vi "myRIO_BRig_RT_v0,82__PortC.vi"() -> ()   [LabVIEW 2014]
uses:
  myRIO_BRig_RT__Case_Exp_stateList.ctl
  myRIO_BRig_RT__Case_NonExp_stateList.ctl
  <vilib>/Platform/TimedLoop/XDataNode/timing_clust.ctl
  <vilib>/Platform/TimedLoop/XDataNode/nitl_modes.ctl
  <vilib>/Platform/TimedLoop/XDataNode/wakeup.ctl
  <vilib>/WebDAVClient/Advanced/SessionHandle.ctl
  <vilib>/myRIO/Common/Instrument Driver Framework/myRIO v1.0/UART/vis/myRIO v1.0 Close UART.vi
  <vilib>/FPGAPlugInAG/myRIO-1900/niLvFpga_Open_myRIO-1900.vi
  <vilib>/rvi/interface/common/dynamic/niFpgaDynamicAddResources.vi
  <vilib>/Utility/error.llb/Error Cluster From Error Code.vi
  <vilib>/rvi/errors/niLvFpgaAdjustHostInterfaceError.vi
  <vilib>/FPGAPlugInAG/Dynamic/niLvFpga_Close_Dynamic.vi
  <vilib>/myRIO/Common/Instrument Driver Framework/Utilities/vis/FPGA Ref Manager.vi
  <vilib>/myRIO/Common/Instrument Driver Framework/myRIO v1.0/myRIO v1.0 Reset FPGA.vi
  <vilib>/myRIO/Common/Instrument Driver Framework/myRIO v1.0/IRQ/vis/myRIO v1.0 IRQ Info FGV.vi
  <vilib>/myRIO/Common/Instrument Driver Framework/myRIO v1.0/IRQ/vis/myRIO v1.0 Timer IRQ Info FGV.vi
  <vilib>/myRIO/Common/Instrument Driver Framework/myRIO v1.0/IRQ/vis/myRIO v1.0 ISR Agent.vi
  <vilib>/rvi/interface/nirviOpenFPGA/nirviOpenFPGA.xnode
  myRIO_BRig_FPGA_v3,71__PortC__build.lvbitx
  myRIO_BRig_FPGA_v3,71__PortC.vi
  <vilib>/rvi/interface/nirviReadWriteControl/nirviReadWriteControl.xnode
  <vilib>/Platform/TimedLoop/XDataNode/XDataNode.xnode
  <vilib>/rvi/interface/nirviCloseFPGA/nirviCloseFPGA.xnode
  <vilib>/Platform/TimedLoop/XDataNode/XDNodeRunTimeDep.lvlib
  <vilib>/rvi/interface/Simulation/niFpgaSimulationCallBeginRW.vi
  <vilib>/myRIO/Instrument Drivers/Utilities/Utilities.lvlib
  <vilib>/WebDAVClient/NI_WebDAV.lvlib
  NiFpgaLv.dll
panel:
  in  "MTrig_CueLed":bool
  out "Threshold":bool
  out "tLoop":dbl
  in  "Tcycle_Cue_LED_max":u16=1000 caption="Max" min=5 max=5000 step=5
  in  "Tcycle_Cue_LED_min":u16=1000 caption="Min" min=5 max=5000 step=5
  in  "Tcycle_CuePenalty_LED":u16=1000 caption="Penalty" min=1 max=10000 step=1
  out "power_l2":dbl
  in  "MTrig_Laser_Switch":bool
  in  "Cue1Param_AudioLed_Count_NS":u16
  in  "Cue1Param_AudioLed_Count_Switch":u16
  in  "Cue1Param_AudioLed_Probability_NS":u16
  in  "Cue1Param_CueType_NS":u16(slide) max=2 step=1 scale=0.0..2.0
  in  "Cue1Param_AudioLed_Probability_Switch":u16
  in  "Cue1Param_CueType_Switch":u16(slide) max=2 step=1 scale=0.0..2.0
  in  "CueLed_Freq":dbl=10.0
  in  "CueLed_Tpeak":dbl=2.0
  in  "Laser_power_step_l2":dbl
  in  "Laser_power_max_l2":dbl
  in  "Laser_power_min_l2":dbl
  in  "Laser_Tshutter_l2":dbl=2.0
  in  "Laser_Freq_l2":dbl=10.0
  in  "Laser_Tpeak_l2":dbl=2.0
  in  "Laser_duration_l2":u16
  in  "LC_Sel_Count_NS_l2":u16
  in  "LC_Sel_Count_Switch_l2":u16
  in  "LC_Sel_Probability_NS_l2":u16
  in  "LC_Sel_Block_NS_l2":u16(slide) max=2 step=1 scale=0.0..2.0
  in  "LC_Sel_OnOff_NS_l2":bool
  in  "LC_Sel_Probability_Switch_l2":u16
  in  "LC_Sel_Block_Switch_l2":u16(slide) max=2 step=1 scale=0.0..2.0
  in  "LC_Sel_OnOff_Switch_l2":bool
  in  "LC_Sel_Tdelay_NS_l2":u16
  in  "LC_Sel_Tdelay_Switch_l2":u16
  in  "LC_Cue1_Count_NS_l2":u16
  in  "LC_Cue1_Count_Switch_l2":u16
  in  "LC_Cue1_delayOpt_NS_l2":bool
  in  "LC_ENL1_delayOpt_NS_l2":bool
  in  "LC_ENL1_Count_NS_l2":u16
  in  "LC_ENL1_Count_Switch_l2":u16
  in  "LC_Cue1_delayOpt_Switch_l2":bool
  in  "LC_ENL1_delayOpt_Switch_l2":bool
  in  "LC_Cue1_Probability_NS_l2":u16
  in  "LC_Cue1_Block_NS_l2":u16(slide) max=2 step=1 scale=0.0..2.0
  in  "LC_Cue1_OnOff_NS_l2":bool
  in  "LC_Cue1_Probability_Switch_l2":u16
  in  "LC_Cue1_Block_Switch_l2":u16(slide) max=2 step=1 scale=0.0..2.0
  in  "LC_Cue1_OnOff_Switch_l2":bool
  in  "LC_ENL1_Probability_NS_l2":u16 max=100 step=1
  in  "LC_ENL1_Block_NS_l2":u16(slide) max=2 step=1 scale=0.0..2.0
  in  "LC_ENL1_OnOff_NS_l2":bool
  in  "LC_ENL1_Probability_Switch_l2":u16 max=100 step=1
  in  "LC_ENL1_Block_Switch_l2":u16(slide) max=2 step=1 scale=0.0..2.0
  in  "LC_Cue1_Tdelay_NS_l2":u16
  in  "LC_ENL1_Tdelay_NS_l2":u16
  in  "LC_Cue1_Tdelay_Switch_l2":u16
  in  "LC_ENL1_Tdelay_Switch_l2":u16
  in  "LC_ENL1_OnOff_Switch_l2":bool
  in  "LC_Wrong_Probability_l2":u16
  in  "LC_Wrong_Trial_l2":u16(slide) max=2 step=1 scale=0.0..2.0
  in  "LC_Wrong_Block_l2":u16(slide) max=2 step=1 scale=0.0..2.0
  in  "LC_Wrong_OnOff_l2":bool
  in  "LC_Reward_Probability_l2":u16
  in  "LC_Reward_Trial_l2":u16(slide) max=2 step=1 scale=0.0..2.0
  in  "LC_Reward_Block_l2":u16(slide) max=2 step=1 scale=0.0..2.0
  in  "LC_Reward_OnOff_l2":bool
  in  "LC_Wrong_Tdelay_l2":u16
  in  "LC_Reward_Tdelay_l2":u16
  in  "LC_Sel_Count_NS_l1":u16
  in  "LC_Sel_Count_Switch_l1":u16
  in  "LC_Sel_Probability_NS_l1":u16
  in  "LC_Sel_Block_NS_l1":u16(slide) max=2 step=1 scale=0.0..2.0
  in  "LC_Sel_OnOff_NS_l1":bool
  in  "LC_Sel_Probability_Switch_l1":u16
  in  "LC_Sel_Block_Switch_l1":u16(slide) max=2 step=1 scale=0.0..2.0
  in  "LC_Sel_OnOff_Switch_l1":bool
  in  "LC_Sel_Tdelay_NS_l1":u16
  in  "LC_Sel_Tdelay_Switch_l1":u16
  out "I_connect_TCP":bool
  in  "get_countPerMS":bool
  in  "count_warmup_R_reset":bool
  in  "count_warmup_L_reset":bool
  out "count_warmup_R":u16
  out "count_warmup_L":u16
  out "SolenoidReward":bool
  in  "SolenoidProbability_L":u16=100 caption="Reward Time [ms]" min=1 max=1000 step=1
  in  "SolenoidProbability_R":u16=100 caption="Reward Time [ms]" min=1 max=1000 step=1
  out "power_l1":dbl caption="LaserPower"
  in  "Laser_power_step_l1":dbl
  in  "Laser_power_max_l1":dbl
  in  "Recording":bool
  in  "Laser_power_min_l1":dbl
  in  "FPGA_count2ms":dbl=159.0
  in  "Laser_Tshutter_l1":dbl=2.0
  in  "Laser_Freq_l1":dbl=10.0
  in  "Laser_Tpeak_l1":dbl=2.0
  in  "Laser_duration_l1":u16
  out "error out":errorcluster
  in  "LC_Cue1_Count_NS_l1":u16
  in  "LC_Cue1_Count_Switch_l1":u16
  in  "LC_Cue1_delayOpt_NS_l1":bool
  in  "LC_ENL1_delayOpt_NS_l1":bool
  in  "LC_ENL1_Count_NS_l1":u16
  in  "LC_ENL1_Count_Switch_l1":u16
  in  "LC_Cue1_delayOpt_Switch_l1":bool
  in  "LC_ENL1_delayOpt_Switch_l1":bool
  in  "Tcycle_Cue_Audio_max":u16=1000 caption="Max" min=5 max=5000 step=5
  in  "Tcycle_Cue_Audio_min":u16=1000 caption="Min" min=5 max=5000 step=5
  in  "SendData":bool
  out "cSpout":enum16{"Left", "Right"}(ring) caption="Left or Right Spout"
  out "A4":u32 caption="LickCounter_Right"
  out "A2":u32 caption="LickCounter_Left"
  in  "LR_wrong_Event":bool
  out "SelectWrong":bool
  out "SelectReward":bool
  in  "Left(F)_or_Right(T)":bool
  in  "ignoreWrong":bool
  in  "SelectionState":bool
  in  "LR_wrong_Laser":bool
  in  "LR_reward_Laser":bool
  in  "LR_reward_Event":bool
  out "nRewards_Right":u16 caption="# Rewards Total (Right)"
  out "nRewards_Left":u16 caption="# Rewards Total (Left)"
  out "nRewards_cur":u16 caption="# Rewards in Current Block"
  out "TpB_target":u16 caption="Target Trials Per Block"
  out "cState_NonExp":T1 caption="WarmUp State"
  out "iBlock":u16 caption="Current Block"
  out "cState":T2 caption="Experimental State"
  out "iTrial":u16 caption="Current Trial"
  in  "warmupType":u8(slide) max=2 step=1 scale=0.0..2.0
  in  "TestConnection":bool
  in  "warmup":bool caption="WarmUp"
  in  "Data Set Prefix":string="Exp1_TM2"
  out "Connected To Host?":bool
  in  "Host Password":string="sabalab"
  in  "Host UserName":string="Test2"
  in  "sp_RightSpout":u16(slide)=2 max=2 step=1 scale=0.0..2.0
  in  "sp_LeftSpout":u16(slide)=2 max=2 step=1 scale=0.0..2.0
  in  "BUR_max":u16 caption="Count Reward Structure  (0 = off)"
  in  "LC_Wrong_Probability_l1":u16
  in  "LC_Wrong_Trial_l1":u16(slide) max=2 step=1 scale=0.0..2.0
  in  "LC_Wrong_Block_l1":u16(slide) max=2 step=1 scale=0.0..2.0
  in  "LC_Wrong_OnOff_l1":bool
  in  "LC_Reward_Probability_l1":u16
  in  "LC_Reward_Trial_l1":u16(slide) max=2 step=1 scale=0.0..2.0
  in  "LC_Reward_Block_l1":u16(slide) max=2 step=1 scale=0.0..2.0
  in  "LC_Reward_OnOff_l1":bool
  in  "LC_Cue1_Probability_NS_l1":u16
  in  "LC_Cue1_Block_NS_l1":u16(slide) max=2 step=1 scale=0.0..2.0
  in  "LC_Cue1_OnOff_NS_l1":bool
  in  "LC_Cue1_Probability_Switch_l1":u16
  in  "LC_Cue1_Block_Switch_l1":u16(slide) max=2 step=1 scale=0.0..2.0
  in  "LC_Cue1_OnOff_Switch_l1":bool
  in  "LC_ENL1_Probability_NS_l1":u16 max=100 step=1
  in  "LC_ENL1_Block_NS_l1":u16(slide) max=2 step=1 scale=0.0..2.0
  in  "LC_ENL1_OnOff_NS_l1":bool
  in  "LC_ENL1_Probability_Switch_l1":u16 max=100 step=1
  in  "LC_ENL1_Block_Switch_l1":u16(slide) max=2 step=1 scale=0.0..2.0
  in  "Tcycle_Timeout":u16=1000 caption="Timeout Time [ms]" min=10 max=10000 step=1
  in  "Tcycle_Wrong":u16=1000 caption="Wrong Time [ms]" min=10 max=10000 step=1
  in  "Tcycle_Selection":u16=1000 caption="Answer Time [ms]" min=1 max=10000 step=1
  in  "Tcycle_RewardPost":u16=1000 caption="Consumption Time [ms]" min=250 max=10000 step=250
  in  "Tcycle_Reward_L":u16=500 caption="Reward Time [ms]" min=1 max=1000 step=1
  in  "Tcycle_Reward_R":u16=500 caption="Reward Time [ms]" min=1 max=1000 step=1
  in  "TpB_Max_R":u16=4 caption="Max TrialsPerBlock" min=1 max=12 step=1
  in  "TpB_Min_R":u16=4 caption="Min TrialsPerBlock" min=1 max=12 step=1
  in  "TpB_Max_L":u16=4 caption="Max TrialsPerBlock" min=1 max=12 step=1
  in  "TpB_Min_L":u16=4 caption="Min TrialsPerBlock" min=1 max=12 step=1
  in  "BUR_min":u16 caption="Count Reward Structure\n(0 = off)"
  in  "TrialUntilReward":bool caption="Ignore Wrong Selection"
  in  "CueCycles":u16=1 caption="Cue Structure" min=1 max=1 step=1
  in  "MTrig_Laser_Tcycle":u16=10 caption="Time [ms]"
  in  "MTrig_Laser_trig":bool
  in  "MTrig_Audio_trig__R":bool caption="Trigger Audio"
  in  "MTrig_Audio_trig__L":bool caption="Trigger Audio"
  in  "RewCalib_Trig_R":bool caption="Calibrate_R"
  in  "RewCalib_Trig_L":bool caption="Calibrate_L"
  in  "MTrig_Solenoid_Tcycle__R":u16=300 caption="Time [ms]"
  in  "MTrig_Solenoid_Tcycle__L":u16=300 caption="Time [ms]"
  in  "MTrig_Solenoid_trig__R":bool caption="Solenoid"
  in  "MTrig_Solenoid_trig__L":bool caption="Solenoid"
  in  "STOP_abort":bool caption="Stop LabView\n(Stops myRio and FPGA)"
  in  "STOP_endBlock":bool caption="Stop Experiment\n@ End of Block"
  in  "STOP_endTrial":bool caption="Stop Experiment\n@ End of Trial"
  in  "START":bool caption="Start Experiment"
  in  "Tcycle_CuePenalty_Audio":u16=1000 caption="Penalty" min=1 max=10000 step=1
  in  "Audio_Amp__R":u16=100 caption="Amp"
  in  "Audio_Freq__R":u8=5 caption="Freq [kHz]" max=14 step=1
  in  "Audio_Amp__L":u16=100 caption="Amp"
  in  "Audio_Freq__L":u8=5 caption="Freq [kHz]" max=14 step=1
  in  "LC_Wrong_Tdelay_l1":u16
  in  "LC_Cue1_Tdelay_NS_l1":u16
  in  "LC_ENL1_Tdelay_NS_l1":u16
  in  "LC_Reward_Tdelay_l1":u16
  in  "LC_Cue1_Tdelay_Switch_l1":u16
  in  "LC_ENL1_Tdelay_Switch_l1":u16
  in  "LC_ENL1_OnOff_Switch_l1":bool
  in  "Tcycle_ENLPenalty":u16=100 caption="Penalty" min=10 max=10000 step=10
  in  "Tcycle_ENL_max":u16=1000 caption="Max" min=250 max=10000 step=250
  in  "Tcycle_ENL_min":u16=1000 caption="Min" min=250 max=10000 step=250
  # "Communication (Host PC)"
  # "Recording Rig"
  # "Experimental Run"
  # "Current State"
  # "STOP experiment at"
  # "Global Parameters                                                         Trial Parameters"
  # "Left/Right        Give Reward?        Laser Power [V]"
  # "Laser1      Laser2"
  # "FPGA Count per [ms]"
  # "Experiment Task Structure"
  # "Block                   Trial            Target Trials       # Rewards \n                                                            Per Block             Current"
  # "Min            Max            Penalty"
  # "(1) = Switching\n(2) = Two Choice"
  # "WarmUp State"
  # "Lick Counter"
  # "Enforced\nNonLick"
  # "WarmUp"
  # "Left           Right"
  # "Cue then reward (no lick)\n \nLeft                    Right"
  # "# Rewards Total\n                                                                  Left                    Right"
  # "Cue Audio"
  # "Experimental State"
  # "Cue LED"
  # "Selection\n \n\n \nReward\n    Dispense\n    Time\n \n    Dispense\n    Probability\n \n\n    Consumption\n    Time\n\nWrong Choice\n \n \nTimeout Penalty"
  # "Left                  Right"
  # "Manual Control"
  # "Min"
  # "Max"
  # "Solenoid\n \nLeft              Right"
  # "Speaker\n \nLeft                    Right"
  # "Laser 1  |  Laser 2"
  # "Trial Per Block Structure \n               Left                        Right"
  # "Time\n[ms]"
  # "Time\n[ms]"
  # "Time = Cue Min"
  # "Min"
  # "Cue LED"
  # "Power = Min"
  # "Max"
  # "Cue1 Control\n                                  Cue Type           LED Probability [%]      Count"
  # "Laser1 Control\n                               On/Off      Block        Probability [%]   Delay [ms]                              Count"
  # "Laser2 Control\n                               On/Off      Block        Probability [%]   Delay [ms]                              Count"
  # "Audio or LED"
  # "Cue 1"
  # "Enforced\nNonLick\n      1"
  # "Enforced\nNonLick\n      1"
  # "from end"
  # "from end"
  # "Switch\nTrial"
  # "Switch\nTrial"
  # "Switch\nTrial"
  # "from start"
  # "from start"
  # "from end"
  # "from end"
  # "NonSwitch\nTrials"
  # "NonSwitch\nTrials"
  # "NonSwitch\nTrials"
  # "from start"
  # "from start"
  # "Cue 1"
  # "Cue 1"
  # "from end"
  # "from end"
  # "Switch\nTrial"
  # "Switch\nTrial"
  # "Cue Audio Parameters"
  # "Cue LED Parameters"
  # "from start"
  # "from start"
  # "Left                  Right"
  # "Frequency\n[Hz]"
  # "Frequency\n[kHz]"
  # "from end"
  # "from end"
  # "NonSwitch\nTrials"
  # "NonSwitch\nTrials"
  # "Timing [ms]\n                    Peak Width"
  # "from start"
  # "from start"
  # "Amp\n(0 - 32,000)"
  # "Selection"
  # "Selection"
  # "from start"
  # "from start"
  # "Switch\nTrial"
  # "Switch\nTrial"
  # "Speaker\nPattern\nDuring Cue"
  # "from start"
  # "from start"
  # "NonSwitch\nTrials"
  # "NonSwitch\nTrials"
  # "Laser1 Parameters"
  # "Laser2 Parameters"
  # "Laser1 Response\n                               On/Off      Block       Trial       Probability [%]   Delay [ms]"
  # "Laser2 Response\n                               On/Off      Block       Trial       Probability [%]   Delay [ms]"
  # "Frequency\n[Hz]"
  # "Frequency\n[Hz]"
  # "Timing [ms]\n Duration     Peak Width   Shutter"
  # "Timing [ms]\n Duration     Peak Width   Shutter"
  # "Selection Reward"
  # "Selection Reward"
  # "Laser Power [V]\nMin          Max              Step"
  # "Laser Power [V]\nMin          Max              Step"
  # "Selection Wrong"
  # "Selection Wrong"
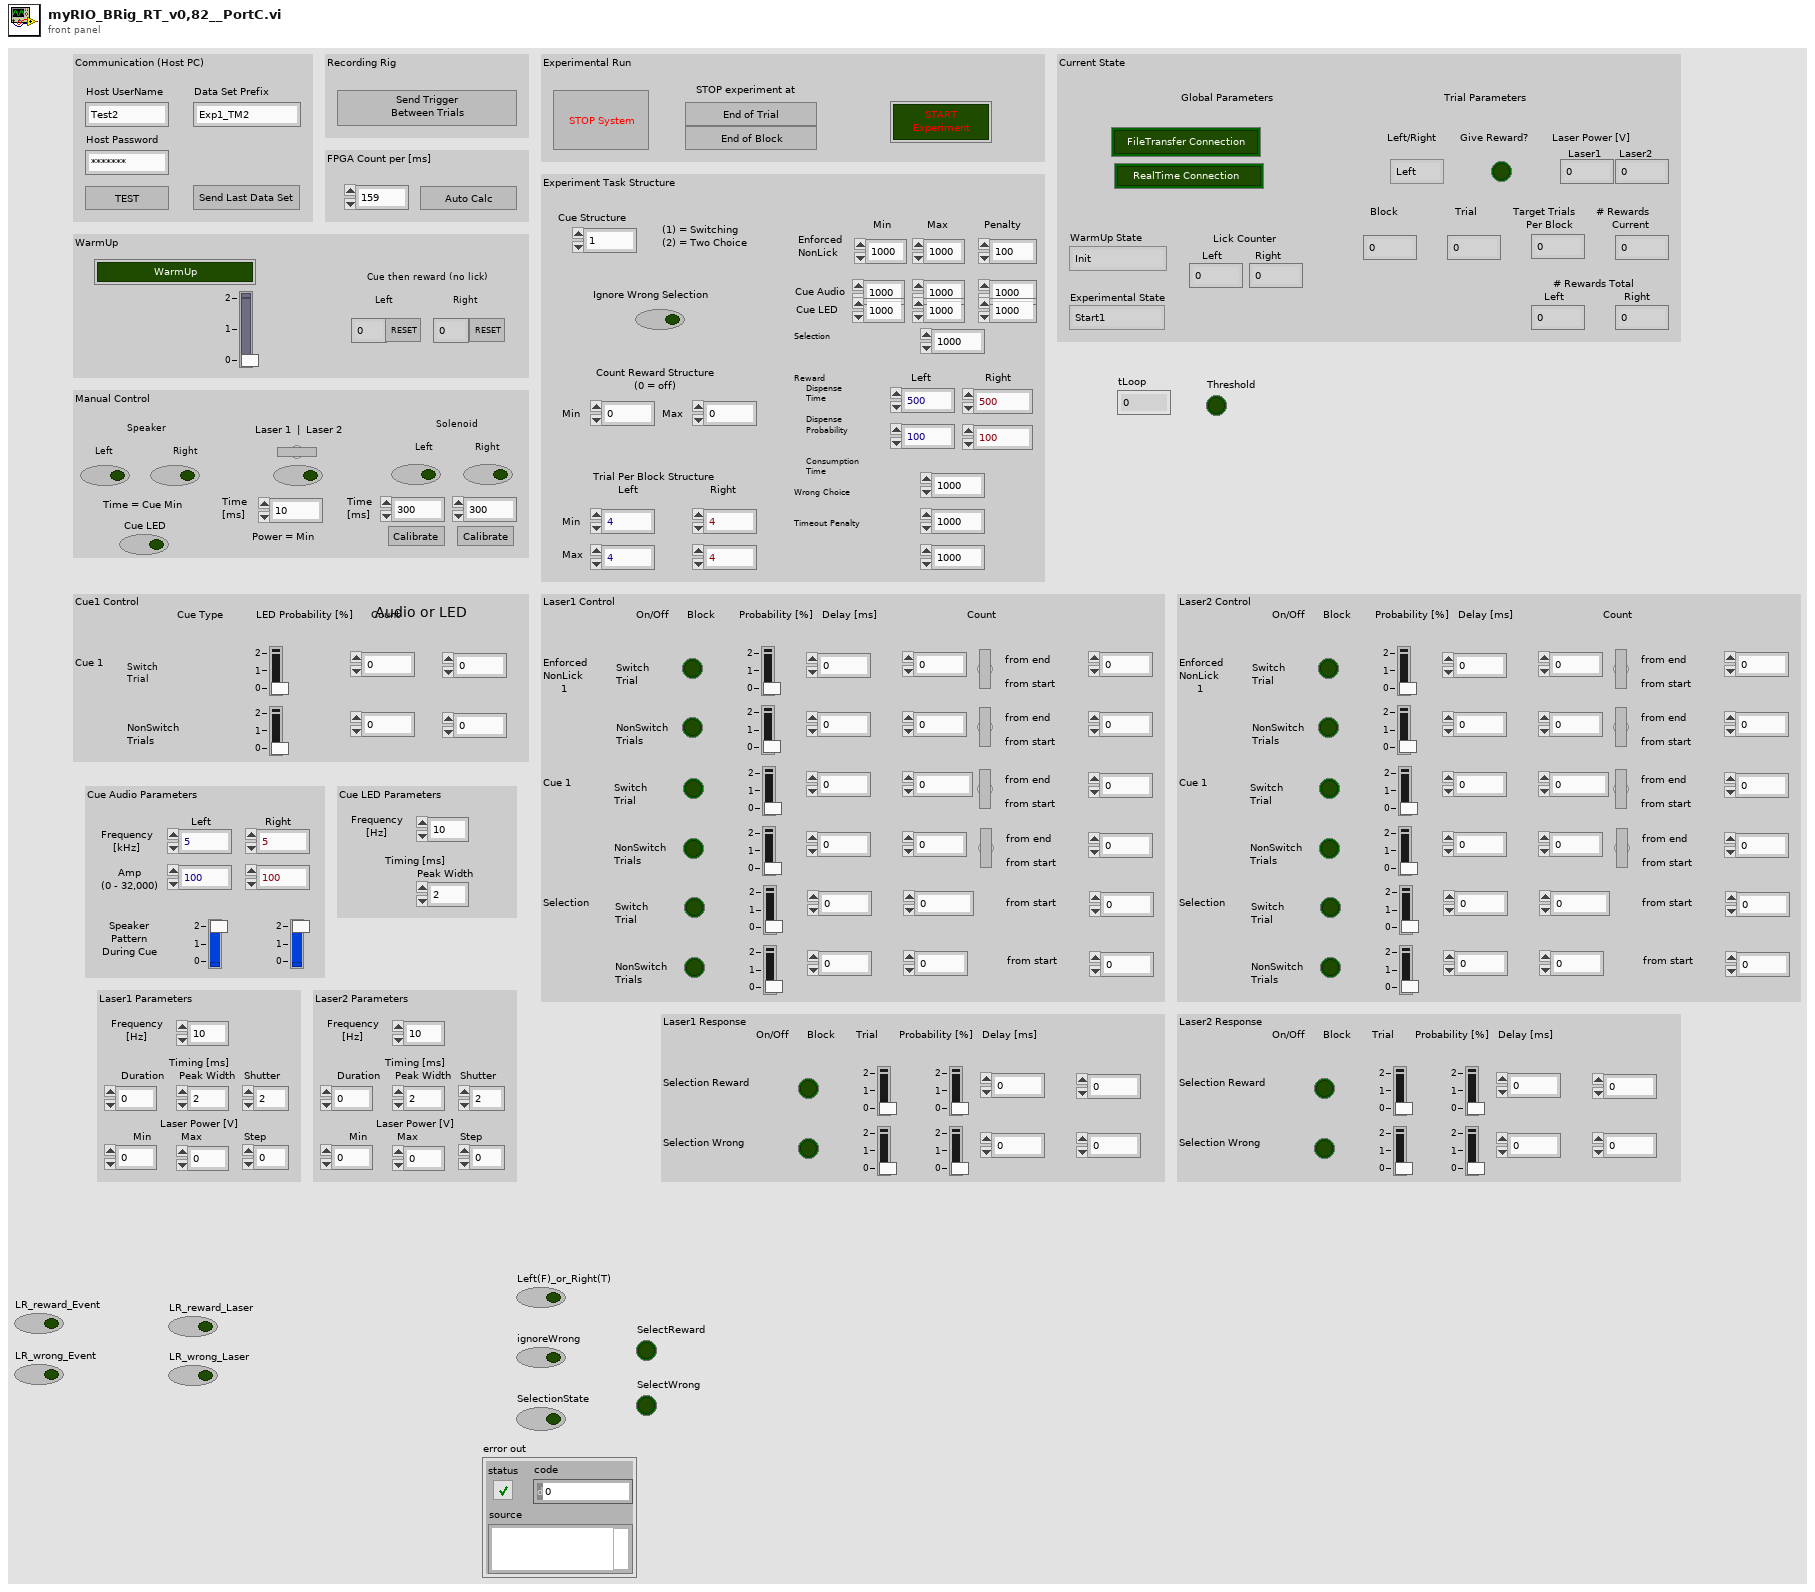
[diagram p1: front panel]
types:
  T1 = typedef "myRIO_BRig_RT__Case_NonExp_stateList.ctl" = enum16{"Init", "UploadSettings_pre", "UploadSettings_Read_dataExp", "UploadSettings_dataExp_1", "UploadSettings_dataExp_2", "UploadSettings_Read_dataLC", "UploadSettings_dataLC_1", "UploadSettings_dataLC_2", "UploadSettings_dataLC_3", "UploadSettings_dataLC_4", "UploadSettings_Read_dataMTrig", "UploadSettings_dataMTrig_1", "UploadSettings_post", "Idle_pre", "IdleEmpty", "IdleEmpty2", "IdleEmpty3", "IdleEmpty4", "Idle", "Idle_2", "Idle_3", "Idle_4", "Idle_5", "Idle_6", "Idle_post", "Cue_pre__pre", "Cue_pre", "Cue", "Cue_LED", "Cue_post", "RewardCalibration_pre", "DispenseWater_pre__pre", "DispenseWater_pre", "DispenseWater", "DispenseWater_post", "TestConnection", "SendData", "Get_FPGA_count_per_ms", "End"}
  T2 = typedef "myRIO_BRig_RT__Case_Exp_stateList.ctl" = enum16{"Start1", "Start2", "Start3", "saveSettings1", "saveSettings2", "saveSettings3", "saveSettings4", "saveSettings_LC_ENL_l1", "saveSettings_LC_ENL_l2", "saveSettings_LC_Cue_l1", "saveSettings_LC_Cue_l2", "saveSettings6_LC_l1_Other", "SaveSettings6_LC_l2_Other", "setSettings_Audio", "setSettings_Laser", "initBlock_pre", "initBlock", "initBlock2", "initBlock_post", "initTrial_pre", "initTrial", "initTrial2", "initTrial3", "initTrial4", "initTrial_LC_ENL1", "initTrial_LC_Cue1", "initTrial_LC_Cue1_2", "initTrial_LC_Sel", "initTrial_post", "ENL1_pre", "ENL1", "ENL1_post", "ENL1Penalty_pre", "ENL1Penalty", "ENL2_pre", "ENL2", "ENL2Penalty_pre", "ENL2Penalty", "Cue1_pre", "Cue1", "Cue1_post", "Cue1Penalty_pre", "Cue1Penalty", "Cue2_pre", "Cue2", "Cue2Penalty_pre", "Cue2Penalty", "Selection_pre", "Selection", "Select_post", "SelectReward_pre", "SelectReward", "SelectRewardPost_pre", "SelectRewardPost", "SelectWrong_pre", "SelectWrong", "SelectWrong_post", "SelectTimeout_pre", "SelectTimeout", "SelectTimeout_post", "endTrial_pre", "endTrial1", "endTrial2", "endTrial3", "endTrial_post", "endBlock_pre", "endBlock", "endBlock_post", "endExp", "commConnect", "commUpload_pre", "commUpload_dataBlock", "commUpload_dataCurrent", "commUpload_dataExp", "commUpload_dataLC", "commUpload_dataTrial", "commUpload_post", "saveData_pre", "saveData_dataBlock", "saveData_dataCurrent", "saveData_dataExp", "saveData_dataLC", "saveData_dataTrial", "saveData_post", "empty_endBlock1", "empty_endBlock2", "empty_endTrial1", "empty_endTrial2", "empty_endTrial3", "empty_endTrial4", "empty_endTrial5", "dummyState", "dummyState_endBlock"}
  T3 = typedef "XDNodeRunTimeDep.lvlib/timing_clust.ctl" = cluster{"Expected End [f-1]":u64, "Actual End [f-1]":u64, "Finished Late? [f-1]":bool, "Expected End [i-1]":u64, "Actual End [i-1]":u64, "Finished Late? [i-1]":bool, "Expected Start [i]":u64, "Actual Start [i]":u64, "Expected Start [f]":u64, "Actual Start [f]":u64, "Source Name":string, "Structure Name":string, "Period":i64, "Deadline":i64, "Offset":i64, "Start":i64, "Priority":i32, "Timeout":i32, "Mode":T4, "Wakeup Reason":T5, "Error":errorcluster, "Source Type":string, "Secondary Source Type":string, "Global End Time":u64, "Global Start Time":u64, "Frame Duration":u64, "Iteration Duration":u64, "Assigned CPU":i32, "I/O Scan Engine Mode":u32}
  T4 = typedef "XDNodeRunTimeDep.lvlib/nitl_modes.ctl" = enum32{"No Change", "Process missed periods, maintain original phase", "Discard missed periods, maintain original phase", "Process missed periods, ignore original phase", "Discard missed periods, ignore original phase"}
  T5 = typedef "XDNodeRunTimeDep.lvlib/wakeup.ctl" = enum32{"Normal", "Aborted", "Asynchronous wakeup", "Timing source error", "Timed loop error", "Timeout"}
  T6 = typedef "NI_WebDAV.lvlib/SessionHandle.ctl" = refnum<k1>
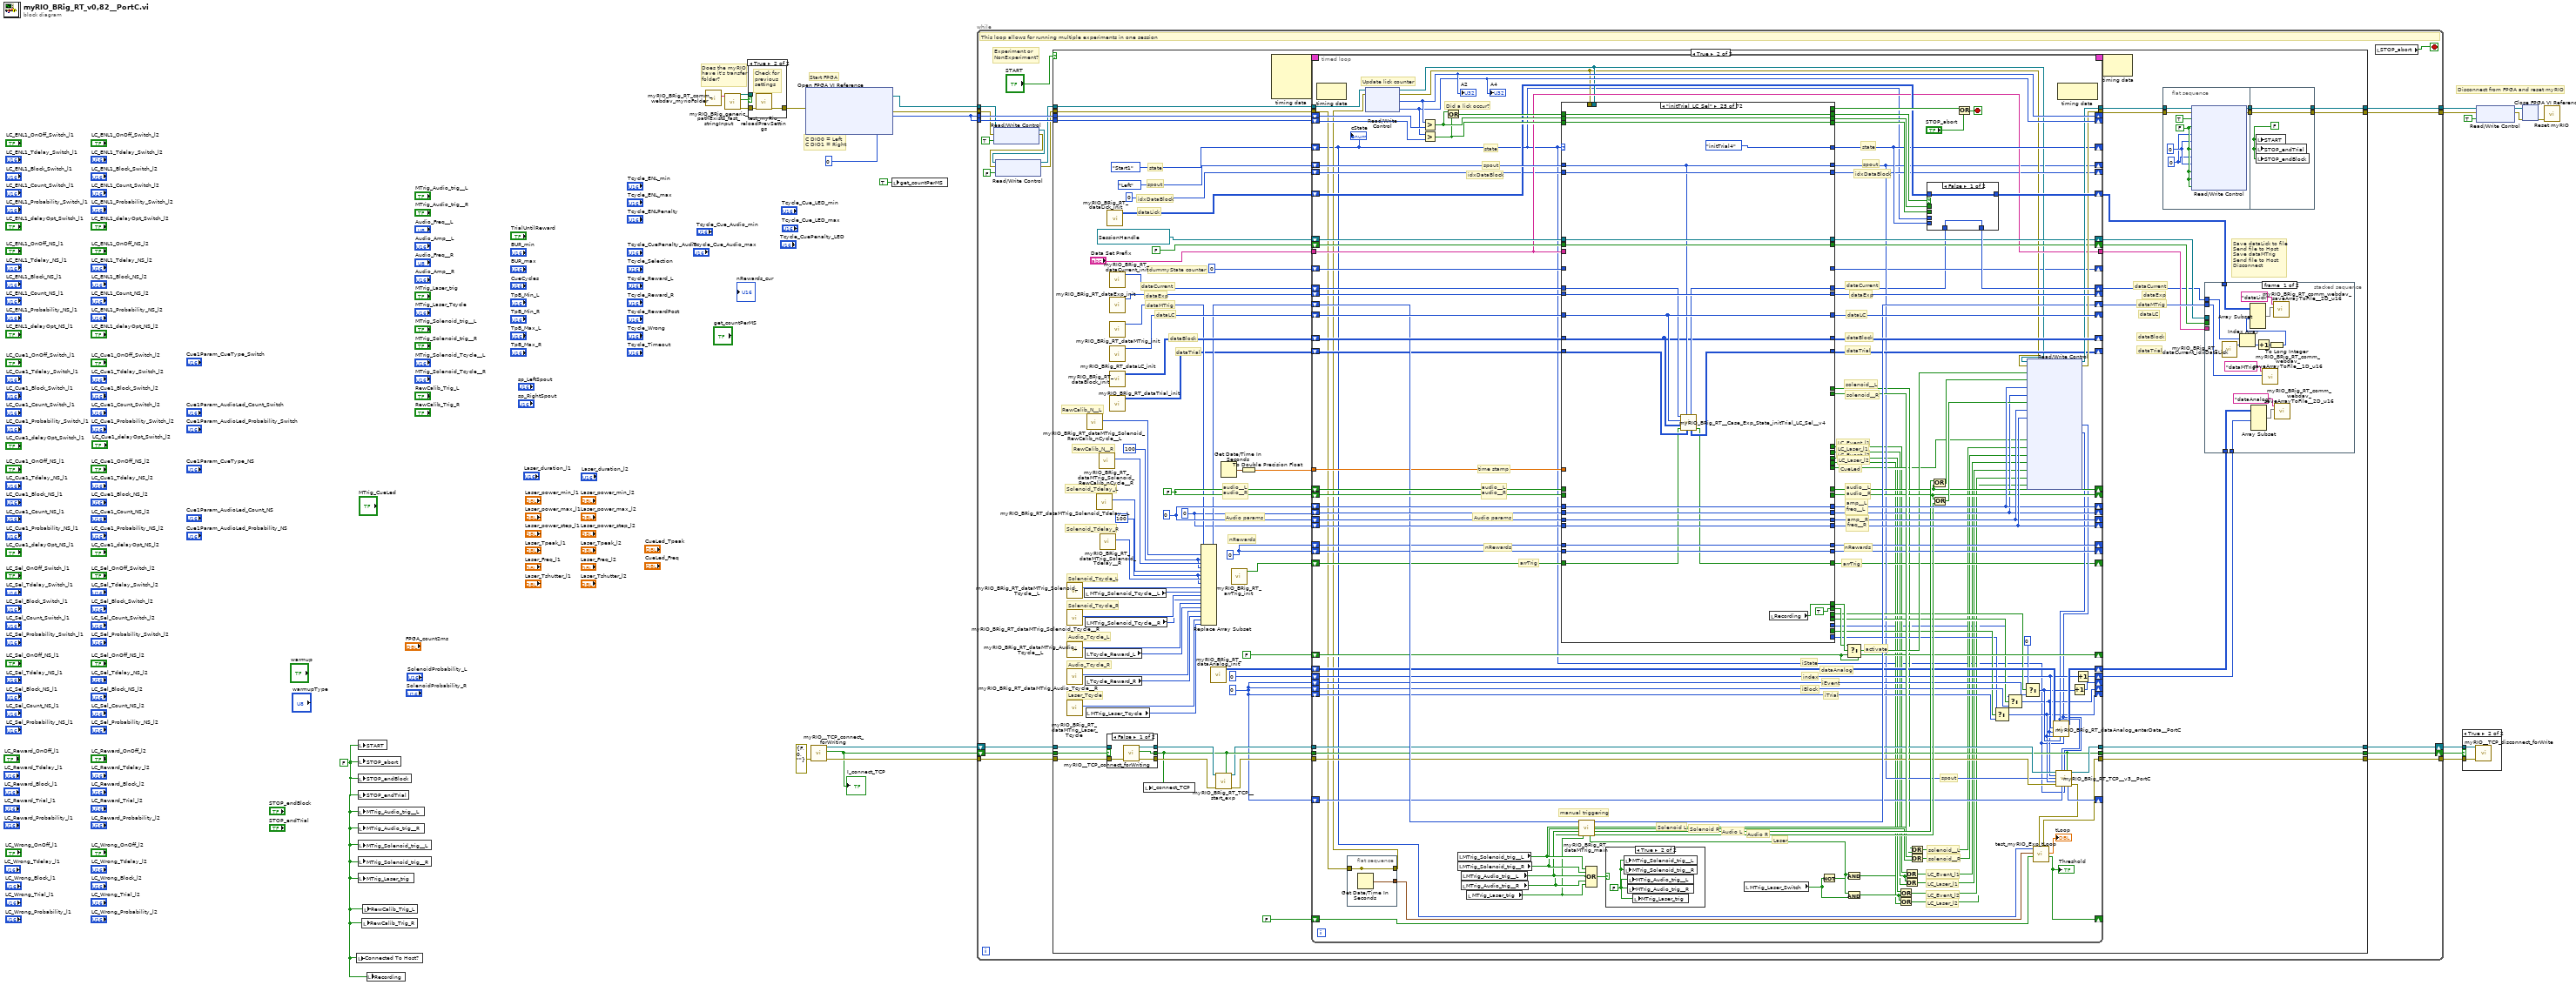
[diagram p0: block diagram]
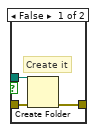
[diagram p3: hidden frame]
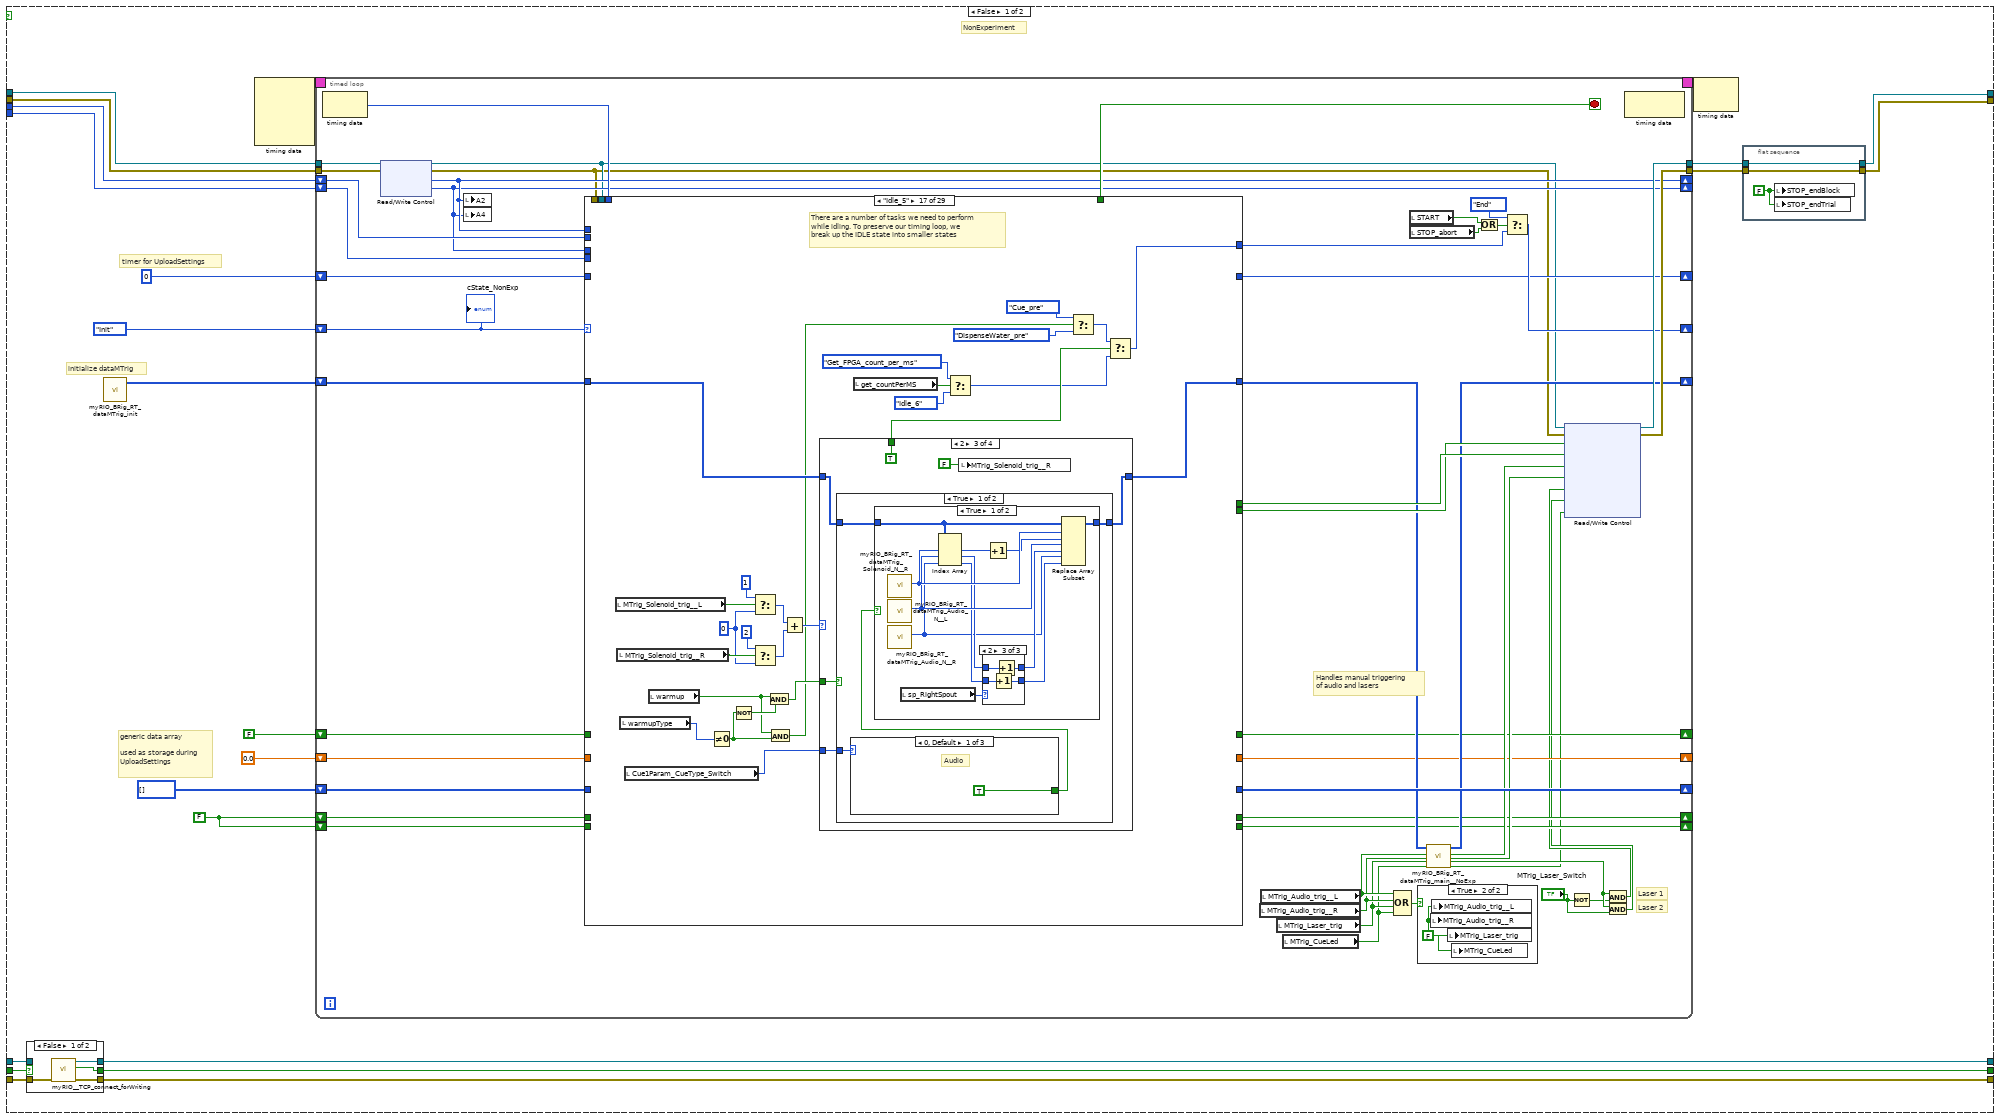
[diagram p4: hidden frame]
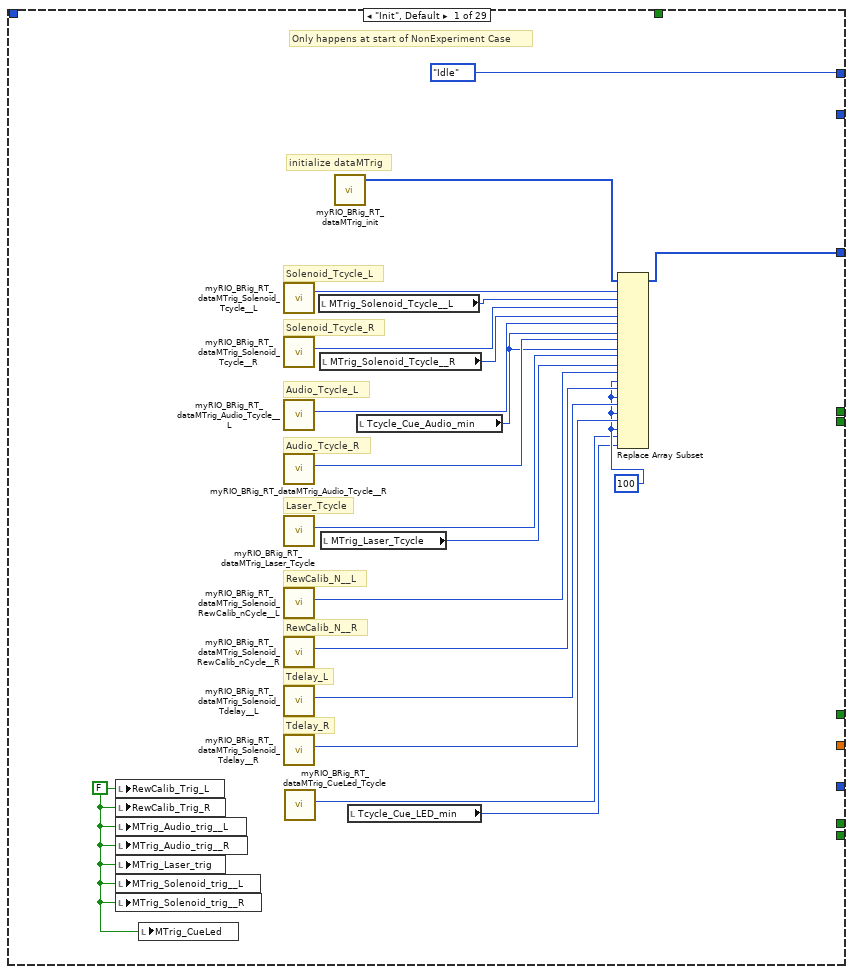
[diagram p7: hidden frame]
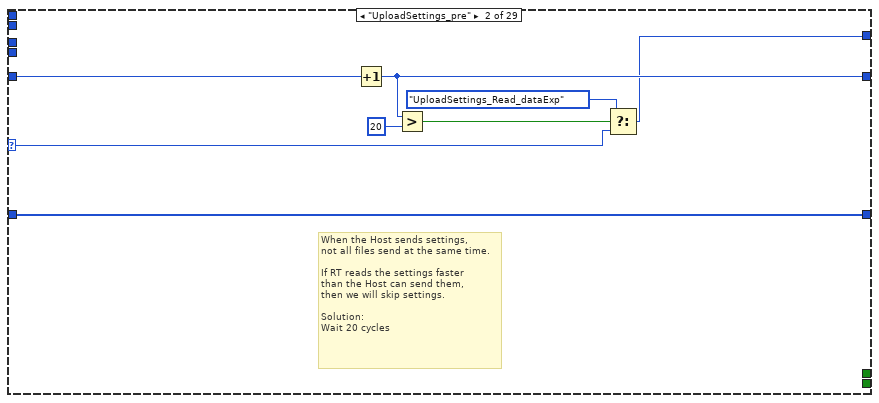
[diagram p8: hidden frame]
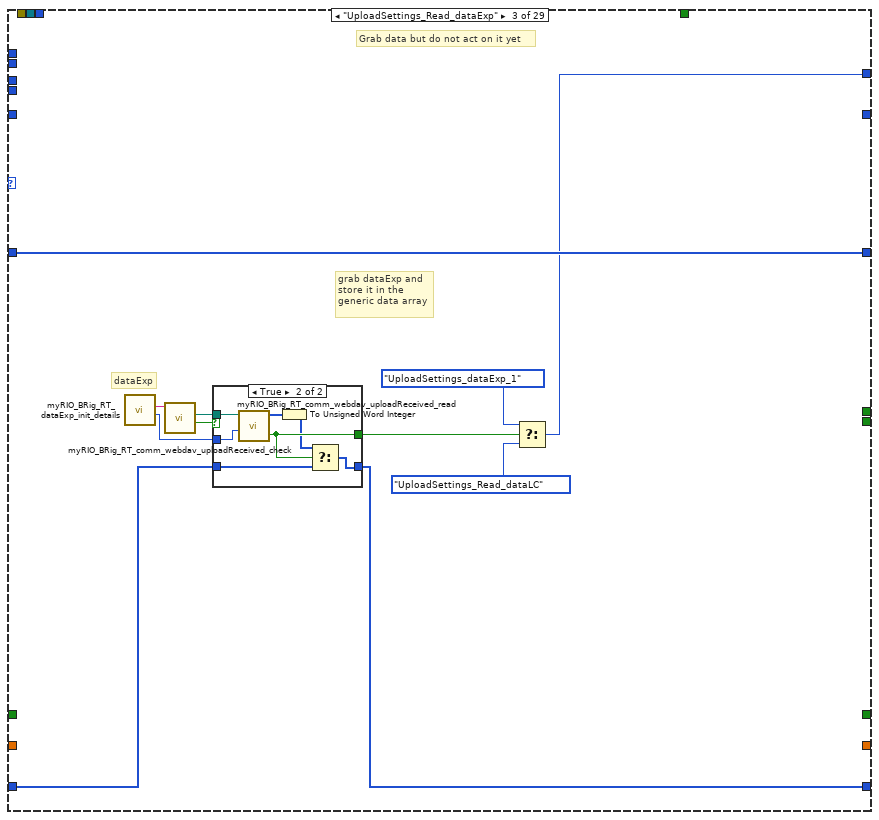
[diagram p9: hidden frame]
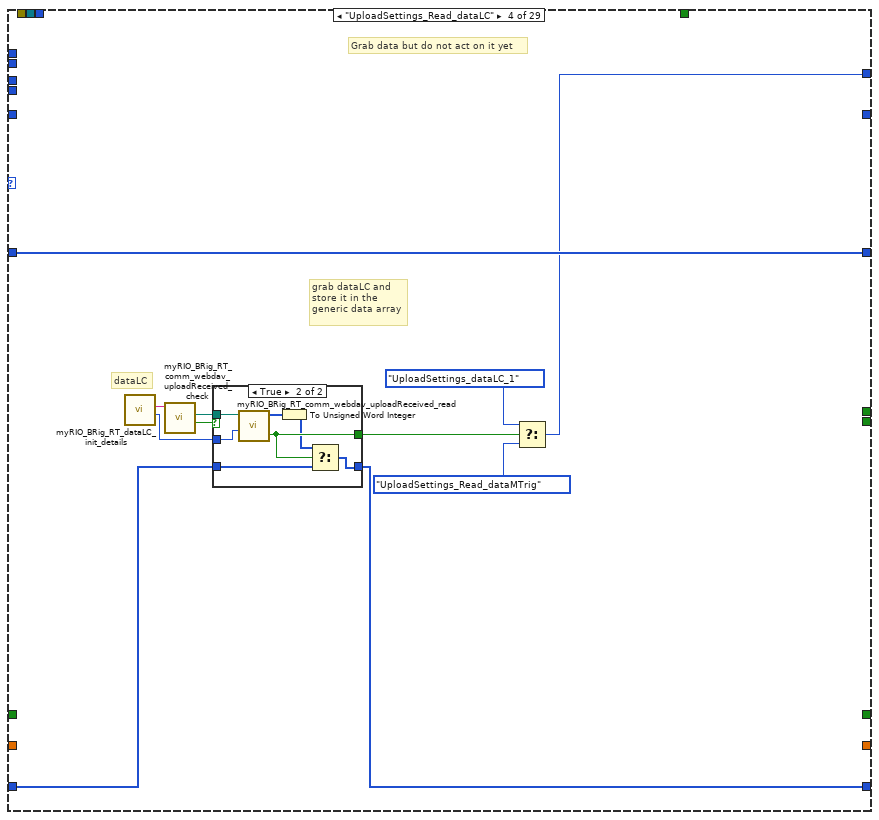
[diagram p11: hidden frame]
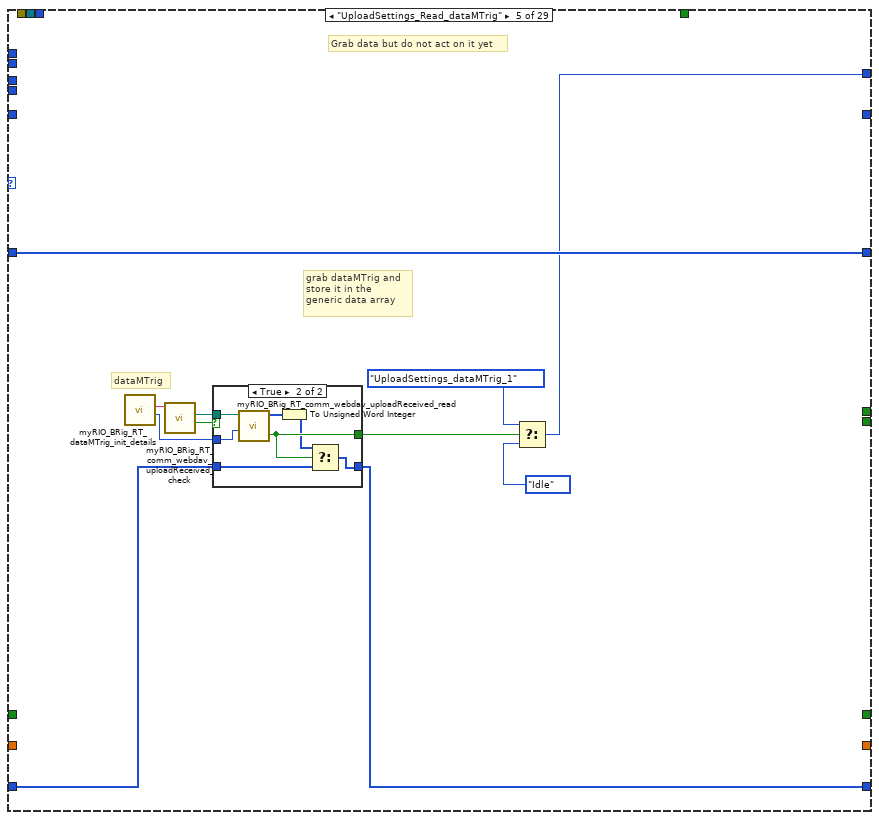
[diagram p13: hidden frame]
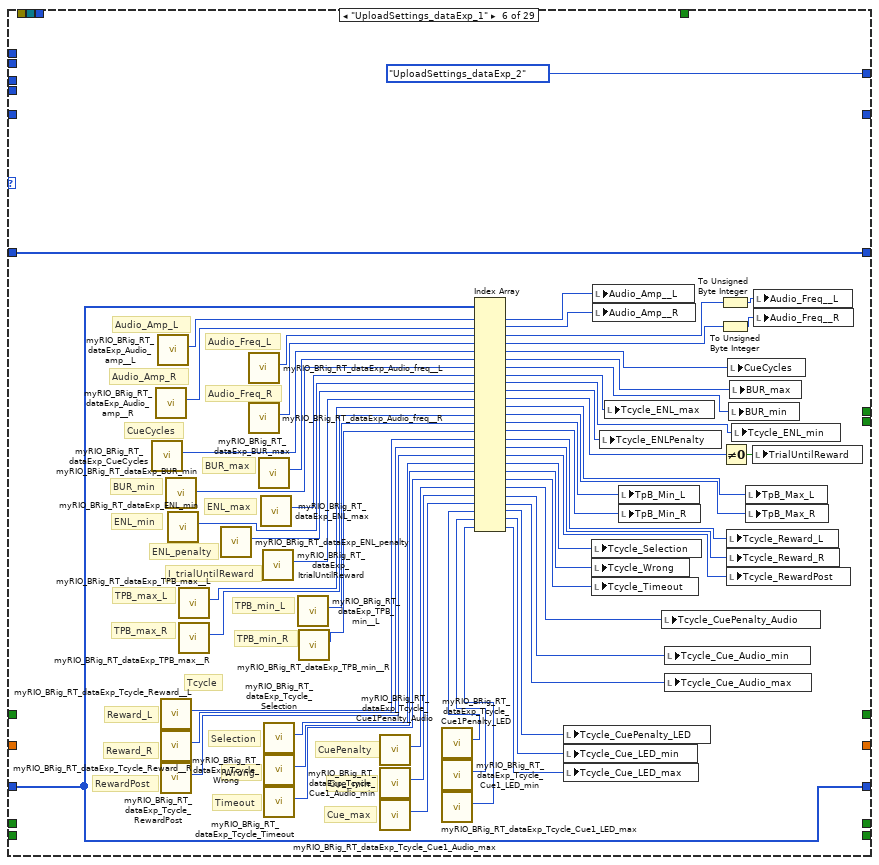
[diagram p15: hidden frame]
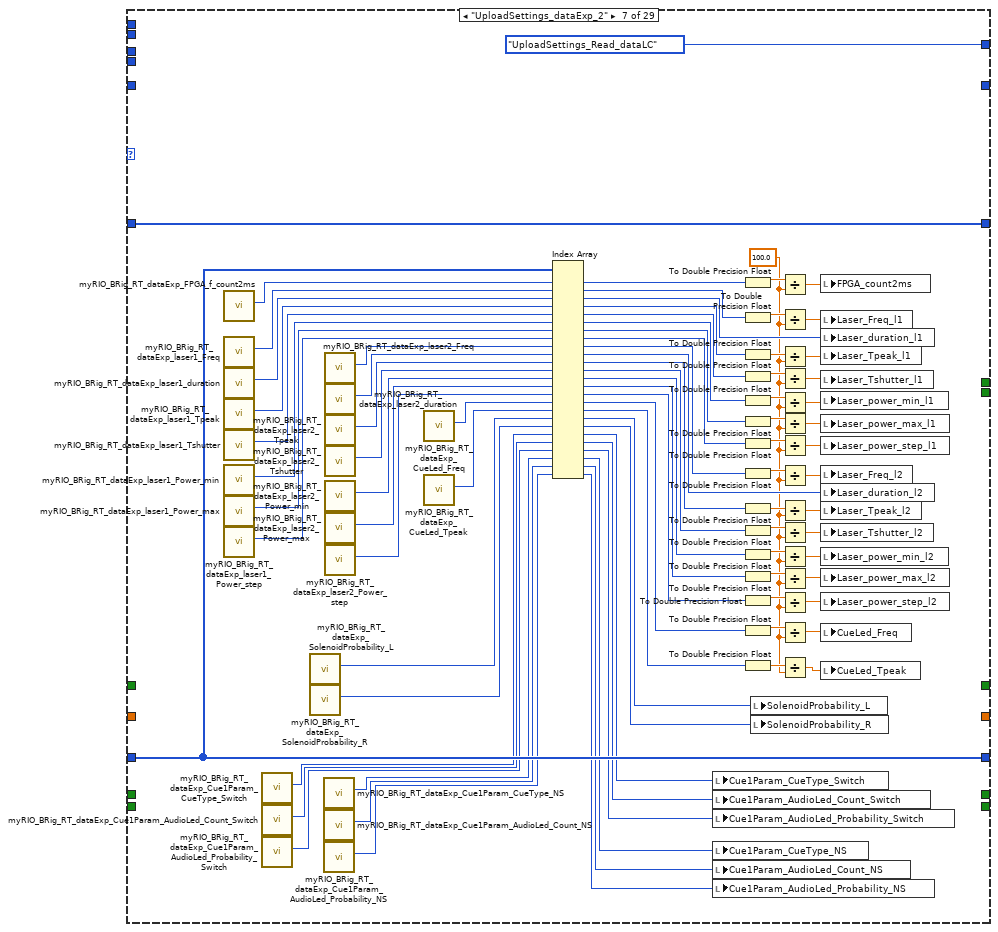
[diagram p16: hidden frame]
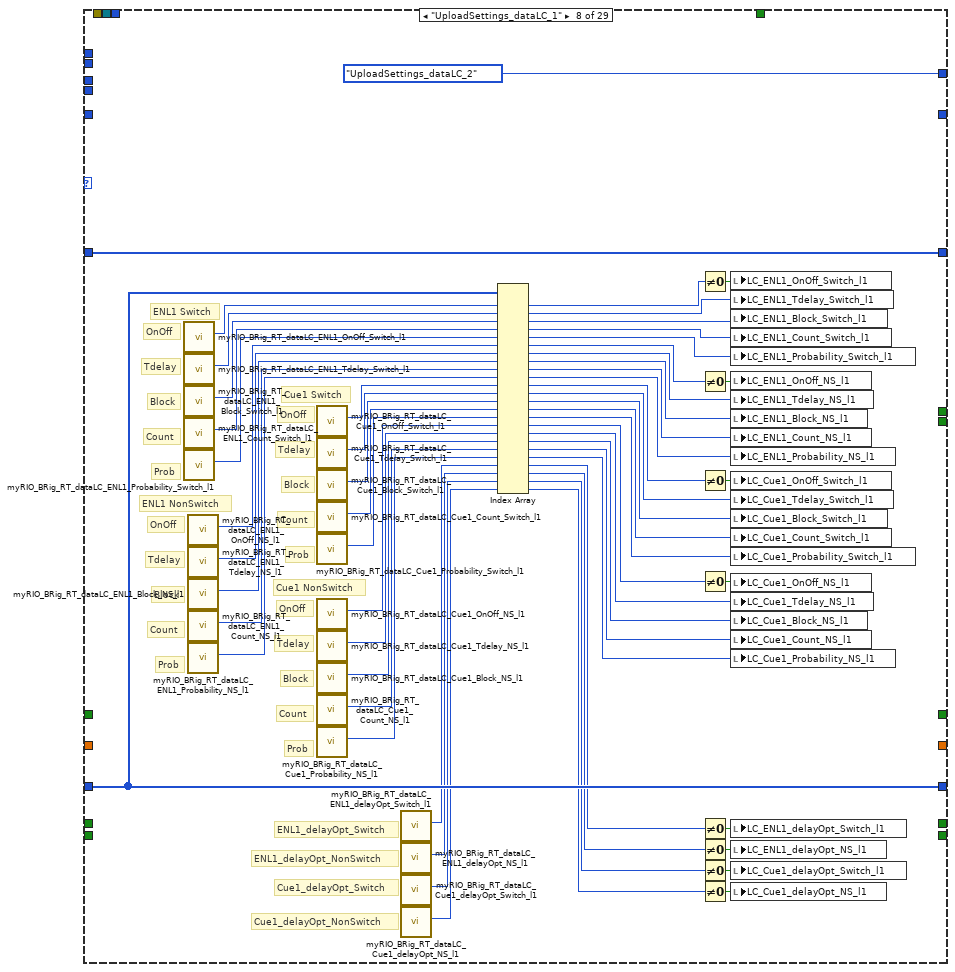
[diagram p17: hidden frame]
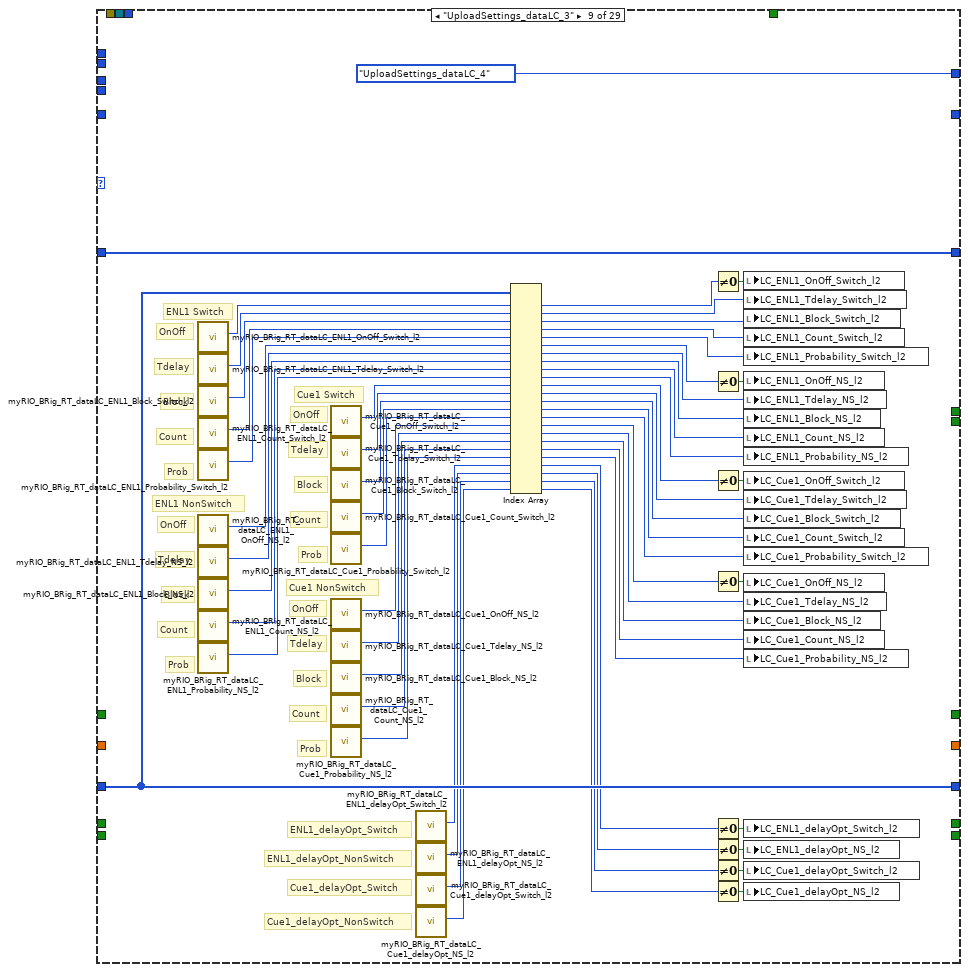
[diagram p18: hidden frame]
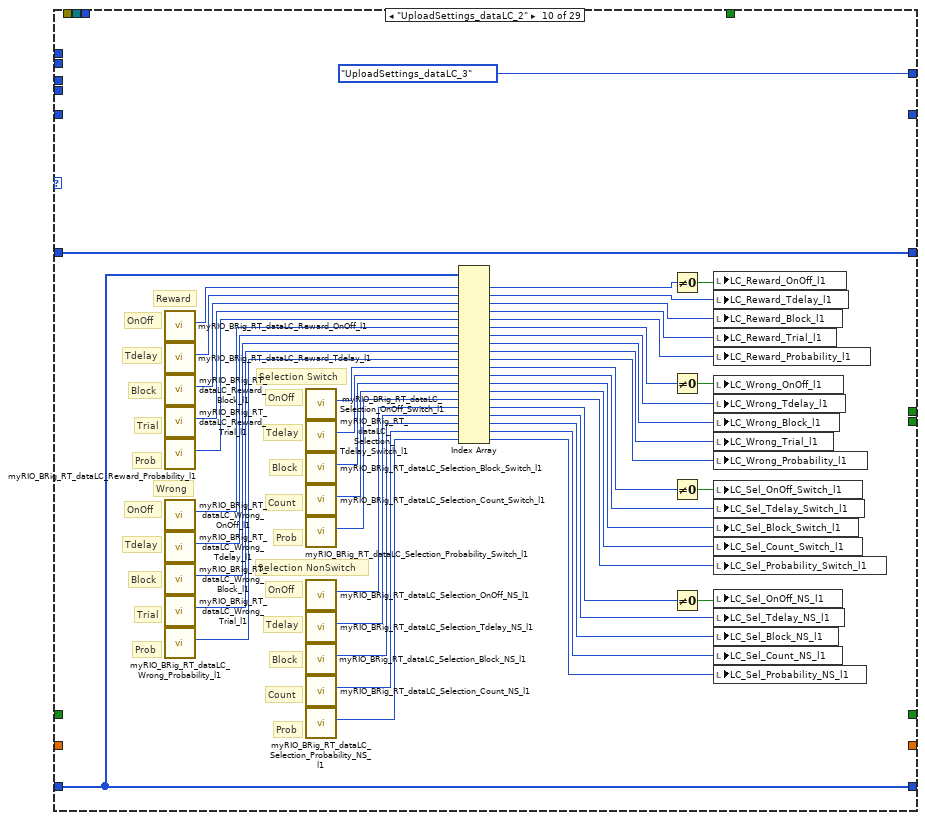
[diagram p19: hidden frame]
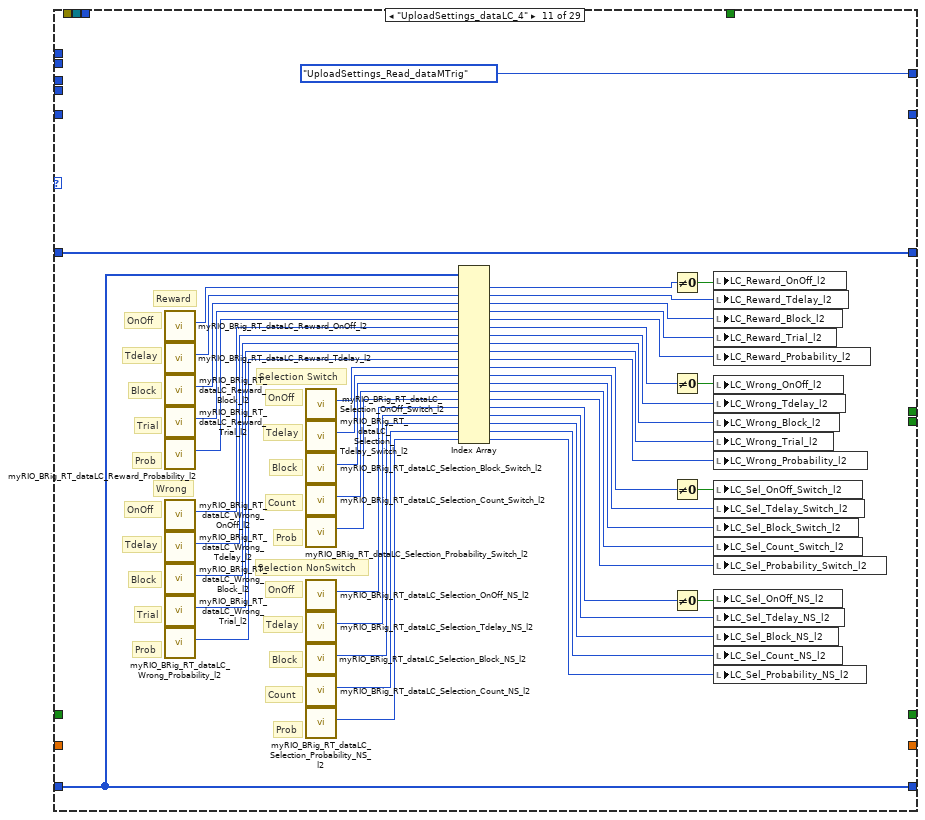
[diagram p20: hidden frame]
diagram:
  w17 = u32 0
  w1 = FALSE
  # "Does the myRIO\nhave it's transfer\nfolder?"
  # "C DIO0 = Left\nC DIO1 = Right"
  # "Start FPGA"
  # "Disconnect from FPGA and reset myRIO"
  n1 = local write "Connected To Host?"(w1) -> ()
  n2 = local write "START"(w1) -> ()
  n3 = local write "STOP_abort"(w1) -> ()
  n4 = local write "STOP_endBlock"(w1) -> ()
  n5 = local write "STOP_endTrial"(w1) -> ()
  n6 = local write "MTrig_Audio_trig__L"(w1) -> ()
  n7 = local write "MTrig_Audio_trig__R"(w1) -> ()
  n8 = local write "MTrig_Solenoid_trig__L"(w1) -> ()
  n9 = local write "MTrig_Solenoid_trig__R"(w1) -> ()
  n10 = local write "MTrig_Laser_trig"(w1) -> ()
  n11 = local write "RewCalib_Trig_R"(w1) -> ()
  n12 = local write "RewCalib_Trig_L"(w1) -> ()
  n13 = local write "Recording"(w1) -> ()
  n14 = call "myRIO_BRig_RT_comm_webdav_myrioFolder.vi"() -> ("output_myrioFolder"=w14:string)  [unwired: 11 in]
  n15 = call "myRIO_BRig_generic_pathExists_fast_stringInput.vi"("input_filePath"=w14) -> ("output_error"=w13:errorcluster, "output_Iexist"=w12:bool, "output_filePath"=w11:path)  [unwired: 8 in]
  n16 = case shown="True" w12 {
    tunnel: w11 -> [w26 _]
    tunnel: w13 -> [w25 w28]
    tunnel: [w24 w27] -> w9
    frame False {
      # "Create it"
      n17 = Create Folder(path (use dialog)=w26, error in=w25) -> (error out=w24:errorcluster)  [unwired: 1 in, 2 out]
    }
    frame True {
      # "Check for\nprevious\nsettings"
      n18 = call "test_myRio_reloadPrevSettings.vi"("input_error"=w28) -> ("output_error"=w27:errorcluster)  [unwired: 10 in]
    }
  }
  n19 = xnode "Open FPGA VI Reference"("error in"=w9) -> ("FPGA VI Reference Out"=w19:refnum<k20>, "error out"=w18:errorcluster)  [unwired: 1 in]
  n20 = call "myRIO__TCP_connect_forWriting.vi"("input_error"=errorcluster {"status"=FALSE, "code"=0, "source"=""}) -> ("output_error"=w7:errorcluster, "output_connected"=w6:bool, "output_hTCP"=w10:refnum<k5>)  [unwired: 8 in]
  "I_connect_TCP" <- w6
  n21 = local write "get_countPerMS"(TRUE ("get_countPerMS")) -> ()
  n22 = while {
    tunnel: w19 -> [w38]
    tunnel: w18 -> [w43]
    tunnel: w17 -> [w46]
    tunnel: w17 -> [w45]
    tunnel: [w36] -> w16
    tunnel: [w35] -> w15
    shift-right: [w32] -> w5
    shift-left: w6 -> [w33]
    tunnel: w7 -> [w31]
    shift-right: [w30] -> w4
    shift-left: w10 -> [w34]
    tunnel: [w29] -> w3
    stop <- w44 stop-if-true
    # "Experiment or\nNonExperiment?"
    # "This loop allows for running multiple experiments in one session"
    n23 = xnode "Read/Write Control"("FPGA VI Reference In"=w38, "error in"=w43, "Counts_Reset"=TRUE) -> ("FPGA VI Reference Out"=w40:refnum<k20>, "error out"=w41:errorcluster)
    n24 = xnode "Read/Write Control"("FPGA VI Reference In"=w40, "error in"=w41, "Counts_Reset"=FALSE) -> ("FPGA VI Reference Out"=w37:refnum<k20>, "error out"=w39:errorcluster)
    n25 = case shown="True" "START" {
      tunnel: w46 -> [w67 w1517]
      tunnel: w45 -> [w66 w1516]
      tunnel: w39 -> [w64 w1448]
      tunnel: w37 -> [w65 w1449]
      tunnel: [w62 w1513] -> w36
      tunnel: [w60 w1508] -> w35
      tunnel: w34 -> [w53 w1459]
      tunnel: [w51 w1463] -> w30
      tunnel: w33 -> [w52 w1461]
      tunnel: [w50 w1462] -> w32
      tunnel: w31 -> [w54 w1460]
      tunnel: [w49 w1458] -> w29
      frame False {
        w57 = FALSE
        # "generic data array\n\nused as storage during\nUploadSettings"
        # "timer for UploadSettings"
        # "initialize dataMTrig"
        # "NonExperiment"
        n26 = case shown="False" w52 {
          selector: w52 -> [_ w76]
          tunnel: w54 -> [w73 w78]
          tunnel: [w74 w78] -> w49
          tunnel: w53 -> [_ w77]
          tunnel: [w75 w77] -> w51
          tunnel: [w72 w76] -> w50
          frame False {
            n27 = call "myRIO__TCP_connect_forWriting.vi"("input_error"=w73) -> ("output_error"=w74:errorcluster, "output_connected"=w72:bool, "output_hTCP"=w75:refnum<k5>)  [unwired: 8 in]
          }
          frame True {
          }
        }
        n28 = call "myRIO_BRig_RT_dataMTrig_init.vi"() -> ("output_dataMTrig"=w68:u16[])  [unwired: 5 in]
        n29 = node-c288() -> (w71:T3)  [unwired: 4 in]
        n30 = timed-loop {
          timing: w71 -> [_]
          timing-out: [_] -> w70
          shift-right: [w117] -> _
          shift-left: w68 -> [w129]
          shift-right: [w111] -> _
          shift-left: myRIO_BRig_RT__Case_NonExp_stateList."Init" ("Enum") -> [w123]
          shift-right: [w105] -> _
          shift-left: w67 -> [w106]
          shift-right: [w103] -> _
          shift-left: w66 -> [w104]
          tunnel: [w125] -> w63
          tunnel: [w124] -> w61
          tunnel: w64 -> [w127]
          tunnel: w65 -> [w126]
          shift-right: [w122] -> _
          shift-left: u16[] [] ("output_data") -> [w121]
          shift-right: [w107] -> _
          shift-left: u16 0 ("Audio_Amp__L") -> [w108]
          shift-right: [w100] -> _
          shift-left: w57 -> [w102]
          shift-right: [w99] -> _
          shift-left: w57 -> [w101]
          shift-right: [w95] -> _
          shift-left: FALSE -> [w96]
          shift-right: [w93] -> _
          shift-left: 0.0 -> [w94]
          stop <- w130 stop-if-true
          # "Laser 2"
          # "Laser 1"
          # "Handles manual triggering\nof audio and lasers"
          n31 = node-c288() -> (w128:i64)  [unwired: 1 in]
          n32 = xnode "Read/Write Control"("FPGA VI Reference In"=w126, "error in"=w127) -> ("FPGA VI Reference Out"=w98:refnum<k20>, "error out"=w97:errorcluster, "A2_LickL"=w105:u32, "A4_LickR"=w103:u32)
          n33 = local write "A2"(w105) -> ()
          n34 = local write "A4"(w103) -> ()
          n35 = case shown="\"Idle_5\"" w123 {
            selector: w123 -> [_ w155 _ _ _ _ _ _ _ _ _ _ _ _ _ _ _ _ _ w1063 w1122 _ _ w1327 _ _ _ w1400 w1441]
            tunnel: [myRIO_BRig_RT__Case_NonExp_stateList."Idle" ("Enum") w153 w160 w179 w198 myRIO_BRig_RT__Case_NonExp_stateList."UploadSettings_dataExp_2" ("Enum") myRIO_BRig_RT__Case_NonExp_stateList."UploadSettings_Read_dataLC" ("Enum") myRIO_BRig_RT__Case_NonExp_stateList."UploadSettings_dataLC_2" ("Enum") myRIO_BRig_RT__Case_NonExp_stateList."UploadSettings_dataLC_4" ("Enum") myRIO_BRig_RT__Case_NonExp_stateList."UploadSettings_dataLC_3" ("f") myRIO_BRig_RT__Case_NonExp_stateList."UploadSettings_Read_dataMTrig" ("f") myRIO_BRig_RT__Case_NonExp_stateList."Idle" ("Enum") w610 w646 myRIO_BRig_RT__Case_NonExp_stateList."Idle_5" ("Enum") w719 w837 w999 w1030 w1058 w1117 myRIO_BRig_RT__Case_NonExp_stateList."DispenseWater_pre" ("Enum") w1273 w1325 w1347 myRIO_BRig_RT__Case_NonExp_stateList."Idle" ("Enum") myRIO_BRig_RT__Case_NonExp_stateList."Idle" ("Enum") w1399 w1441] -> w112
            tunnel: [w143 w152 w170 w189 w208 w276 w360 w413 w472 w525 w572 w588 w614 w661 w705 w724 w842 w997 w1037 w1064 w1123 w1184 w1310 w1332 w1358 w1392 w1397 w1409 w1439] -> w118
            tunnel: [_ _ _ _ _ _ _ _ _ _ _ _ _ _ _ _ _ _ _ _ _ _ _ _ _ _ _ _ TRUE] -> w130
            tunnel: w129 -> [_ w152 w170 w189 w208 w276 w360 w413 w472 w525 w572 w589 w613 w661 w705 w725 w843 w997 w1038 w1065 w1124 w1170 w1306 w1333 w1359 w1392 w1397 w1409 w1439]
            tunnel: w128 -> [_ _ _ _ _ _ _ _ _ _ _ _ _ _ _ _ _ _ _ _ _ _ _ w1337 _ _ _ _ _]
            tunnel: [_ _ w161 w180 w199 w225 w358 w414 w473 w521 w568 w573 _ _ _ _ _ _ w1026 _ w1111 _ _ _ _ _ _ _ _] -> w122
            tunnel: w121 -> [_ _ w162 w181 w200 w225 w358 w414 w473 w521 w568 w573 _ _ _ _ _ _ _ _ w1112 _ _ _ _ _ _ _ _]
            tunnel: [_ _ _ _ _ _ _ _ _ _ _ _ _ _ _ _ _ _ _ _ _ _ _ w1334 _ _ _ _ _] -> w120
            tunnel: [_ _ _ _ _ _ _ _ _ _ _ _ _ _ _ _ _ _ _ _ _ _ _ w1316 _ _ _ _ _] -> w119
            tunnel: w108 -> [_ w159 _ _ _ _ _ _ _ _ _ _ _ _ _ _ _ _ _ _ _ _ _ _ _ _ _ _ _]
            tunnel: [_ w158 _ _ _ _ _ _ _ _ _ _ _ _ _ _ _ _ _ _ _ _ _ _ _ _ _ _ _] -> w107
            tunnel: w106 -> [_ _ _ _ _ _ _ _ _ _ _ _ _ _ _ _ _ _ _ w1069 w1128 _ _ _ _ _ _ _ _]
            tunnel: w105 -> [_ _ _ _ _ _ _ _ _ _ _ _ _ _ _ _ _ _ _ w1070 w1129 _ _ _ _ _ _ _ _]
            tunnel: w104 -> [_ _ _ _ _ _ _ _ _ _ _ _ _ _ _ _ _ _ _ w1067 w1126 _ _ _ _ _ _ _ _]
            tunnel: w103 -> [_ _ _ _ _ _ _ _ _ _ _ _ _ _ _ _ _ _ _ w1068 w1127 _ _ _ _ _ _ _ _]
            tunnel: w102 -> [_ _ _ _ _ _ _ _ _ _ _ _ _ _ _ _ _ _ _ w1055 w1114 _ _ _ _ _ _ _ _]
            tunnel: w101 -> [_ _ _ _ _ _ _ _ _ _ _ _ _ _ _ _ _ _ _ w1054 w1113 _ _ _ _ _ _ _ _]
            tunnel: [_ _ _ _ _ _ _ _ _ _ _ _ _ _ _ _ _ _ w1028 w1055 w1114 _ _ _ _ _ _ _ _] -> w100
            tunnel: [_ _ _ _ _ _ _ _ _ _ _ _ _ _ _ _ _ _ w1027 w1054 w1113 _ _ _ _ _ _ _ _] -> w99
            tunnel: w98 -> [_ _ _ _ _ _ _ _ _ _ _ _ w603 w619 w707 _ _ _ _ _ w1110 _ _ _ _ _ _ w1404 _]
            tunnel: w97 -> [_ _ _ _ _ _ _ _ _ _ _ _ w602 w620 w706 _ _ _ _ _ w1109 _ _ _ _ _ _ w1403 _]
            tunnel: w96 -> [_ _ _ _ _ _ _ _ _ _ _ _ _ _ _ _ _ _ _ _ _ _ _ _ _ _ _ w1408 _]
            tunnel: [_ _ _ _ _ _ _ _ _ _ _ _ _ _ _ _ _ _ _ _ _ _ _ _ _ _ _ TRUE _] -> w95
            tunnel: w94 -> [_ _ _ _ _ _ _ _ _ _ _ _ _ _ _ _ _ _ _ _ _ _ _ _ _ _ _ w1406 _]
            tunnel: [_ _ _ _ _ _ _ _ _ _ _ _ _ _ _ _ _ _ _ _ _ _ _ _ _ _ _ w1405 _] -> w93
            frame "Init", Default {
              w134 = FALSE ("RewCalib_Trig_L")
              w135 = u16 100 ("new element/subarray")
              # "Only happens at start of NonExperiment Case"
              # "Tdelay_R"
              # "Tdelay_L"
              # "RewCalib_N__R"
              # "RewCalib_N__L"
              # "Solenoid_Tcycle_R"
              # "Solenoid_Tcycle_L"
              # "Laser_Tcycle"
              # "Audio_Tcycle_R"
              # "Audio_Tcycle_L"
              # "initialize dataMTrig"
              n36 = local write "RewCalib_Trig_L"(w134) -> ()
              n37 = local write "RewCalib_Trig_R"(w134) -> ()
              n38 = local write "MTrig_Audio_trig__L"(w134) -> ()
              n39 = local write "MTrig_Audio_trig__R"(w134) -> ()
              n40 = local write "MTrig_Laser_trig"(w134) -> ()
              n41 = local write "MTrig_Solenoid_trig__L"(w134) -> ()
              n42 = local write "MTrig_Solenoid_trig__R"(w134) -> ()
              n43 = local write "MTrig_CueLed"(w134) -> ()
              n44 = call "myRIO_BRig_RT_dataMTrig_Solenoid_Tcycle__L.vi"() -> ("output_Solenoid_Tcycle__L"=w145:i32)  [unwired: 11 in]
              n45 = call "myRIO_BRig_RT_dataMTrig_Solenoid_Tcycle__R.vi"() -> ("output_Solenoid_Tcycle__R"=w146:i32)  [unwired: 11 in]
              n46 = call "myRIO_BRig_RT_dataMTrig_Audio_Tcycle__L.vi"() -> ("output_Audio_Tcycle__L"=w147:i32)  [unwired: 11 in]
              n47 = call "myRIO_BRig_RT_dataMTrig_Audio_Tcycle__R.vi"() -> ("output_Audio_Tcycle__R"=w148:i32)  [unwired: 11 in]
              n48 = call "myRIO_BRig_RT_dataMTrig_Laser_Tcycle.vi"() -> ("output_Laser_Tcycle"=w149:i32)  [unwired: 11 in]
              n49 = call "myRIO_BRig_RT_dataMTrig_Solenoid_RewCalib_nCycle__L.vi"() -> ("output_Solenoid_RewCalib_nCycle__L"=w141:i32)  [unwired: 11 in]
              n50 = call "myRIO_BRig_RT_dataMTrig_Solenoid_RewCalib_nCycle__R.vi"() -> ("output_Solenoid_RewCalib_nCycle__R"=w140:i32)  [unwired: 11 in]
              n51 = call "myRIO_BRig_RT_dataMTrig_Solenoid_Tdelay__L.vi"() -> ("output_Solenoid_Tdelay__L"=w139:i32)  [unwired: 11 in]
              n52 = call "myRIO_BRig_RT_dataMTrig_Solenoid_Tdelay__R.vi"() -> ("output_Solenoid_Tdelay__R"=w138:i32)  [unwired: 11 in]
              n53 = call "myRIO_BRig_RT_dataMTrig_CueLed_Tcycle.vi"() -> ("output_CueLed_Tcycle"=w133:i32)  [unwired: 11 in]
              n54 = local read "MTrig_Solenoid_Tcycle__L"() -> (w150:u16)
              n55 = local read "MTrig_Solenoid_Tcycle__R"() -> (w151:u16)
              n56 = local read "MTrig_Laser_Tcycle"() -> (w136:u16)
              n57 = call "myRIO_BRig_RT_dataMTrig_init.vi"() -> ("output_dataMTrig"=w144:u16[])  [unwired: 5 in]
              n58 = local read "Tcycle_Cue_LED_min"() -> (w132:u16)
              n59 = local read "Tcycle_Cue_Audio_min"() -> (w137:u16)
              n60 = Replace Array Subset(array=w144, new element #1=w150, index #1=w145, new element #2=w151, index #2=w146, new element #3=w137, index #3=w147, new element #4=w137, index #4=w148, new element #5=w136, index #5=w149, new element #6=w135, index #6=w141, new element #7=w135, index #7=w140, new element #8=w135, index #8=w139, new element #9=w135, index #9=w138, new element #10=w132, index #10=w133) -> (w143:u16[])
            }
            frame "UploadSettings_pre" {
              # "When the Host sends settings,\nnot all files send at the same time.\n\nIf RT reads the settings faster\nthan the Host can send them,\nthen we will skip settings.\n\nSolution:\nWait 20 cycles"
              n61 = Increment(x=w159) -> (x+1=w158:u16)
              n62 = Greater?(x=w158, y=u16 20) -> (0:w156:bool)
              n63 = Select(t=myRIO_BRig_RT__Case_NonExp_stateList."UploadSettings_Read_dataExp", s=w156, f=w155) -> (s? t:f=w153:T1)
            }
            frame "UploadSettings_Read_dataExp" {
              # "Grab data but do not act on it yet"
              # "grab dataExp and\nstore it in the\ngeneric data array"
              # "dataExp"
              n64 = call "myRIO_BRig_RT_dataExp_init_details.vi"() -> ("output_dataSize"=w166:i32, "output_dataName"=w169:string)  [unwired: 10 in]
              n65 = call "myRIO_BRig_RT_comm_webdav_uploadReceived_check.vi"("input_dataName"=w169) -> ("output_Iexist"=w168:bool, "output_dataPath"=w167:path)  [unwired: 9 in]
              n66 = case shown="True" w168 {
                tunnel: w167 -> [_ w178]
                tunnel: w166 -> [_ w177]
                tunnel: [_ w176] -> w165
                tunnel: w162 -> [w171 w175]
                tunnel: [w171 w172] -> w161
                frame False {
                }
                frame True {
                  n67 = call "myRIO_BRig_RT_comm_webdav_uploadReceived_read.vi"("input_dataSize"=w177, "input_filePath"=w178) -> ("output_Ivalid"=w176:bool, "output_data"=w174:i64[])  [unwired: 8 in]
                  n68 = To Unsigned Word Integer(number=w174) -> (unsigned 16bit integer=w173:u16[])
                  n69 = Select(t=w173, s=w176, f=w175) -> (s? t:f=w172:u16[])
                }
              }
              n70 = Select(t=myRIO_BRig_RT__Case_NonExp_stateList."UploadSettings_dataExp_1", s=w165, f=myRIO_BRig_RT__Case_NonExp_stateList."UploadSettings_Read_dataLC" ("t")) -> (s? t:f=w160:T1)
            }
            frame "UploadSettings_Read_dataLC" {
              # "Grab data but do not act on it yet"
              # "grab dataLC and\nstore it in the\ngeneric data array"
              # "dataLC"
              n71 = call "myRIO_BRig_RT_dataLC_init_details.vi"() -> ("output_dataSize"=w185:i32, "output_dataName"=w188:string)  [unwired: 10 in]
              n72 = call "myRIO_BRig_RT_comm_webdav_uploadReceived_check.vi"("input_dataName"=w188) -> ("output_Iexist"=w187:bool, "output_dataPath"=w186:path)  [unwired: 9 in]
              n73 = case shown="True" w187 {
                tunnel: w186 -> [_ w197]
                tunnel: w185 -> [_ w196]
                tunnel: [_ w195] -> w184
                tunnel: w181 -> [w190 w194]
                tunnel: [w190 w191] -> w180
                frame False {
                }
                frame True {
                  n74 = call "myRIO_BRig_RT_comm_webdav_uploadReceived_read.vi"("input_dataSize"=w196, "input_filePath"=w197) -> ("output_Ivalid"=w195:bool, "output_data"=w193:i64[])  [unwired: 8 in]
                  n75 = To Unsigned Word Integer(number=w193) -> (unsigned 16bit integer=w192:u16[])
                  n76 = Select(t=w192, s=w195, f=w194) -> (s? t:f=w191:u16[])
                }
              }
              n77 = Select(t=myRIO_BRig_RT__Case_NonExp_stateList."UploadSettings_dataLC_1", s=w184, f=myRIO_BRig_RT__Case_NonExp_stateList."UploadSettings_Read_dataMTrig" ("t")) -> (s? t:f=w179:T1)
            }
            frame "UploadSettings_Read_dataMTrig" {
              # "Grab data but do not act on it yet"
              # "grab dataMTrig and\nstore it in the\ngeneric data array"
              # "dataMTrig"
              n78 = call "myRIO_BRig_RT_dataMTrig_init_details.vi"() -> ("output_dataSize"=w204:i32, "output_dataName"=w207:string)  [unwired: 10 in]
              n79 = call "myRIO_BRig_RT_comm_webdav_uploadReceived_check.vi"("input_dataName"=w207) -> ("output_Iexist"=w206:bool, "output_dataPath"=w205:path)  [unwired: 9 in]
              n80 = case shown="True" w206 {
                tunnel: w205 -> [_ w216]
                tunnel: w204 -> [_ w215]
                tunnel: [_ w214] -> w203
                tunnel: w200 -> [w209 w213]
                tunnel: [w209 w210] -> w199
                frame False {
                }
                frame True {
                  n81 = call "myRIO_BRig_RT_comm_webdav_uploadReceived_read.vi"("input_dataSize"=w215, "input_filePath"=w216) -> ("output_Ivalid"=w214:bool, "output_data"=w212:i64[])  [unwired: 8 in]
                  n82 = To Unsigned Word Integer(number=w212) -> (unsigned 16bit integer=w211:u16[])
                  n83 = Select(t=w211, s=w214, f=w213) -> (s? t:f=w210:u16[])
                }
              }
              n84 = Select(t=myRIO_BRig_RT__Case_NonExp_stateList."UploadSettings_dataMTrig_1", s=w203, f=myRIO_BRig_RT__Case_NonExp_stateList."Idle" ("t")) -> (s? t:f=w198:T1)
            }
            frame "UploadSettings_dataExp_1" {
              # "Cue_max"
              # "Cue_min"
              # "CuePenalty"
              # "Timeout"
              # "Wrong"
              # "Selection"
              # "RewardPost"
              # "Reward_R"
              # "Reward_L"
              # "Tcycle"
              # "TPB_min_R"
              # "TPB_min_L"
              # "TPB_max_R"
              # "TPB_max_L"
              # "I_trialUntilReward"
              # "ENL_penalty"
              # "ENL_min"
              # "ENL_max"
              # "BUR_max"
              # "BUR_min"
              # "CueCycles"
              # "Audio_Freq_R"
              # "Audio_Freq_L"
              # "Audio_Amp_R"
              # "Audio_Amp_L"
              n85 = call "myRIO_BRig_RT_dataExp_CueCycles.vi"() -> ("output_CueCycles"=w268:i32)  [unwired: 11 in]
              n86 = call "myRIO_BRig_RT_dataExp_Audio_amp__R.vi"() -> ("output_Audio_amp__R"=w272:i32)  [unwired: 11 in]
              n87 = call "myRIO_BRig_RT_dataExp_Audio_amp__L.vi"() -> ("output_Audio_amp__L"=w274:i32)  [unwired: 11 in]
              n88 = call "myRIO_BRig_RT_dataExp_Tcycle_Reward__L.vi"() -> ("output_Tcycle_Reward__L"=w245:i32)  [unwired: 11 in]
              n89 = call "myRIO_BRig_RT_dataExp_Tcycle_Reward__R.vi"() -> ("output_Tcycle_Reward__R"=w244:i32)  [unwired: 11 in]
              n90 = call "myRIO_BRig_RT_dataExp_Tcycle_RewardPost.vi"() -> ("output_Tcycle_RewardPost"=w243:i32)  [unwired: 11 in]
              n91 = call "myRIO_BRig_RT_dataExp_BUR_min.vi"() -> ("output_BUR_min"=w265:i32)  [unwired: 11 in]
              n92 = call "myRIO_BRig_RT_dataExp_ENL_min.vi"() -> ("output_ENL_min"=w261:i32)  [unwired: 11 in]
              n93 = call "myRIO_BRig_RT_dataExp_TPB_max__L.vi"() -> ("output_TPB_max__L"=w253:i32)  [unwired: 11 in]
              n94 = call "myRIO_BRig_RT_dataExp_TPB_max__R.vi"() -> ("output_TPB_max__R"=w252:i32)  [unwired: 11 in]
              n95 = call "myRIO_BRig_RT_dataExp_ENL_penalty.vi"() -> ("output_ENL_penalty"=w260:i32)  [unwired: 11 in]
              n96 = call "myRIO_BRig_RT_dataExp_Audio_freq__L.vi"() -> ("output_Audio_freq__L"=w270:i32)  [unwired: 11 in]
              n97 = call "myRIO_BRig_RT_dataExp_Audio_freq__R.vi"() -> ("output_Audio_freq__R"=w269:i32)  [unwired: 11 in]
              n98 = call "myRIO_BRig_RT_dataExp_BUR_max.vi"() -> ("output_BUR_max"=w266:i32)  [unwired: 11 in]
              n99 = call "myRIO_BRig_RT_dataExp_ENL_max.vi"() -> ("output_ENL_max"=w262:i32)  [unwired: 11 in]
              n100 = call "myRIO_BRig_RT_dataExp_ItrialUntilReward.vi"() -> ("output_I_trialUntilReward"=w256:i32)  [unwired: 11 in]
              n101 = call "myRIO_BRig_RT_dataExp_Tcycle_Selection.vi"() -> ("output_Tcycle_Selection"=w242:i32)  [unwired: 11 in]
              n102 = call "myRIO_BRig_RT_dataExp_Tcycle_Wrong.vi"() -> ("output_Tcycle_Wrong"=w241:i32)  [unwired: 11 in]
              n103 = call "myRIO_BRig_RT_dataExp_Tcycle_Timeout.vi"() -> ("output_Tcycle_Timeout"=w240:i32)  [unwired: 11 in]
              n104 = call "myRIO_BRig_RT_dataExp_TPB_min__L.vi"() -> ("output_TPB_min__L"=w251:i32)  [unwired: 11 in]
              n105 = call "myRIO_BRig_RT_dataExp_TPB_min__R.vi"() -> ("output_TPB_min__R"=w250:i32)  [unwired: 11 in]
              n106 = call "myRIO_BRig_RT_dataExp_Tcycle_Cue1Penalty_Audio.vi"() -> ("output_Tcycle_Cue1Penalty_Audio"=w233:i32)  [unwired: 11 in]
              n107 = call "myRIO_BRig_RT_dataExp_Tcycle_Cue1_Audio_min.vi"() -> ("output_Tcycle_Cue1_Audio_min"=w232:i32)  [unwired: 11 in]
              n108 = call "myRIO_BRig_RT_dataExp_Tcycle_Cue1_Audio_max.vi"() -> ("output_Tcycle_Cue1_Audio_max"=w231:i32)  [unwired: 11 in]
              n109 = call "myRIO_BRig_RT_dataExp_Tcycle_Cue1Penalty_LED.vi"() -> ("output_Tcycle_Cue1Penalty_LED"=w222:i32)  [unwired: 11 in]
              n110 = call "myRIO_BRig_RT_dataExp_Tcycle_Cue1_LED_min.vi"() -> ("output_Tcycle_Cue1_LED_min"=w221:i32)  [unwired: 11 in]
              n111 = call "myRIO_BRig_RT_dataExp_Tcycle_Cue1_LED_max.vi"() -> ("output_Tcycle_Cue1_LED_max"=w220:i32)  [unwired: 11 in]
              n112 = Index Array(array=w225, index #1=w274, index #2=w272, index #3=w270, index #4=w269, index #5=w268, index #6=w266, index #7=w265, index #8=w262, index #9=w261, index #10=w260, index #11=w256, index #12=w253, index #13=w252, index #14=w251, index #15=w250, index #16=w245, index #17=w244, index #18=w243, index #19=w242, index #20=w241, index #21=w240, index #22=w233, index #23=w232, index #24=w231, index #25=w222, index #26=w221, index #27=w220) -> (element #1=w273:u16, element #2=w271:u16, element #3=w228:u16, element #4=w227:u16, element #5=w267:u16, element #6=w264:u16, element #7=w263:u16, element #8=w259:u16, element #9=w258:u16, element #10=w257:u16, element #11=w254:u16, element #12=w249:u16, element #13=w248:u16, element #14=w247:u16, element #15=w246:u16, element #16=w239:u16, element #17=w238:u16, element #18=w237:u16, element #19=w236:u16, element #20=w235:u16, element #21=w234:u16, element #22=w230:u16, element #23=w224:u16, element #24=w223:u16, element #25=w219:u16, element #26=w218:u16, element #27=w217:u16)
              n113 = local write "Tcycle_CuePenalty_LED"(w219) -> ()
              n114 = local write "Tcycle_Cue_LED_min"(w218) -> ()
              n115 = local write "Tcycle_Cue_LED_max"(w217) -> ()
              n116 = local write "Tcycle_Selection"(w236) -> ()
              n117 = local write "Tcycle_Wrong"(w235) -> ()
              n118 = local write "Tcycle_Timeout"(w234) -> ()
              n119 = local write "Audio_Amp__L"(w273) -> ()
              n120 = local write "Audio_Amp__R"(w271) -> ()
              n121 = local write "Tcycle_ENLPenalty"(w257) -> ()
              n122 = local write "Tcycle_ENL_max"(w259) -> ()
              n123 = local write "TpB_Min_L"(w247) -> ()
              n124 = local write "TpB_Min_R"(w246) -> ()
              n125 = local write "Tcycle_CuePenalty_Audio"(w230) -> ()
              n126 = local write "Tcycle_Cue_Audio_min"(w224) -> ()
              n127 = local write "Tcycle_Cue_Audio_max"(w223) -> ()
              n128 = To Unsigned Byte Integer(number=w228) -> (unsigned 8bit integer=w229:u8)
              n129 = To Unsigned Byte Integer(number=w227) -> (unsigned 8bit integer=w226:u8)
              n130 = Not Equal To 0?(x=w254) -> (x != 0?=w255:bool)
              n131 = local write "Tcycle_Reward_L"(w239) -> ()
              n132 = local write "Tcycle_Reward_R"(w238) -> ()
              n133 = local write "Tcycle_RewardPost"(w237) -> ()
              n134 = local write "CueCycles"(w267) -> ()
              n135 = local write "BUR_min"(w263) -> ()
              n136 = local write "BUR_max"(w264) -> ()
              n137 = local write "Tcycle_ENL_min"(w258) -> ()
              n138 = local write "TpB_Max_L"(w249) -> ()
              n139 = local write "TpB_Max_R"(w248) -> ()
              n140 = local write "TrialUntilReward"(w255) -> ()
              n141 = local write "Audio_Freq__L"(w229) -> ()
              n142 = local write "Audio_Freq__R"(w226) -> ()
            }
            frame "UploadSettings_dataExp_2" {
              w296 = 100.0 ("y")
              n143 = call "myRIO_BRig_RT_dataExp_FPGA_f_count2ms.vi"() -> ("output_FPGA_f_count2ms"=w357:i32)  [unwired: 11 in]
              n144 = call "myRIO_BRig_RT_dataExp_laser1_Freq.vi"() -> ("output_laser1_Freq"=w345:i32)  [unwired: 11 in]
              n145 = call "myRIO_BRig_RT_dataExp_laser1_duration.vi"() -> ("output_laser1_duration"=w344:i32)  [unwired: 11 in]
              n146 = call "myRIO_BRig_RT_dataExp_laser1_Tpeak.vi"() -> ("output_laser1_Tpeak"=w343:i32)  [unwired: 11 in]
              n147 = call "myRIO_BRig_RT_dataExp_laser1_Tshutter.vi"() -> ("output_laser1_Tshutter"=w342:i32)  [unwired: 11 in]
              n148 = call "myRIO_BRig_RT_dataExp_laser1_Power_min.vi"() -> ("output_laser1_Power_min"=w341:i32)  [unwired: 11 in]
              n149 = call "myRIO_BRig_RT_dataExp_laser1_Power_max.vi"() -> ("output_laser1_Power_max"=w340:i32)  [unwired: 11 in]
              n150 = call "myRIO_BRig_RT_dataExp_laser1_Power_step.vi"() -> ("output_laser1_Power_step"=w339:i32)  [unwired: 11 in]
              n151 = call "myRIO_BRig_RT_dataExp_Cue1Param_CueType_Switch.vi"() -> ("output_Cue1Param_CueType_Switch"=w290:i32)  [unwired: 11 in]
              n152 = call "myRIO_BRig_RT_dataExp_Cue1Param_AudioLed_Count_Switch.vi"() -> ("output_Cue1Param_AudioLed_Count_Switch"=w289:i32)  [unwired: 11 in]
              n153 = call "myRIO_BRig_RT_dataExp_Cue1Param_AudioLed_Probability_Switch.vi"() -> ("output_Cue1Param_AudioLed_Probability_Switch"=w288:i32)  [unwired: 11 in]
              n154 = call "myRIO_BRig_RT_dataExp_SolenoidProbability_L.vi"() -> ("output_SolenoidProbability_L"=w292:i32)  [unwired: 11 in]
              n155 = call "myRIO_BRig_RT_dataExp_SolenoidProbability_R.vi"() -> ("output_SolenoidProbability_R"=w291:i32)  [unwired: 11 in]
              n156 = call "myRIO_BRig_RT_dataExp_Cue1Param_CueType_NS.vi"() -> ("output_Cue1Param_CueType_NS"=w287:i32)  [unwired: 11 in]
              n157 = call "myRIO_BRig_RT_dataExp_Cue1Param_AudioLed_Count_NS.vi"() -> ("output_Cue1Param_AudioLed_Count_NS"=w286:i32)  [unwired: 11 in]
              n158 = call "myRIO_BRig_RT_dataExp_Cue1Param_AudioLed_Probability_NS.vi"() -> ("output_Cue1Param_AudioLed_Probability_NS"=w285:i32)  [unwired: 11 in]
              n159 = call "myRIO_BRig_RT_dataExp_laser2_Freq.vi"() -> ("output_laser2_Freq"=w338:i32)  [unwired: 11 in]
              n160 = call "myRIO_BRig_RT_dataExp_laser2_duration.vi"() -> ("output_laser2_duration"=w337:i32)  [unwired: 11 in]
              n161 = call "myRIO_BRig_RT_dataExp_laser2_Tpeak.vi"() -> ("output_laser2_Tpeak"=w336:i32)  [unwired: 11 in]
              n162 = call "myRIO_BRig_RT_dataExp_laser2_Tshutter.vi"() -> ("output_laser2_Tshutter"=w335:i32)  [unwired: 11 in]
              n163 = call "myRIO_BRig_RT_dataExp_laser2_Power_min.vi"() -> ("output_laser2_Power_min"=w334:i32)  [unwired: 11 in]
              n164 = call "myRIO_BRig_RT_dataExp_laser2_Power_max.vi"() -> ("output_laser2_Power_max"=w333:i32)  [unwired: 11 in]
              n165 = call "myRIO_BRig_RT_dataExp_laser2_Power_step.vi"() -> ("output_laser2_Power_step"=w332:i32)  [unwired: 11 in]
              n166 = call "myRIO_BRig_RT_dataExp_CueLed_Freq.vi"() -> ("output_CueLed_Freq"=w301:i32)  [unwired: 11 in]
              n167 = call "myRIO_BRig_RT_dataExp_CueLed_Tpeak.vi"() -> ("output_CueLed_Tpeak"=w294:i32)  [unwired: 11 in]
              n168 = Index Array(array=w358, index #1=w357, index #2=w345, index #3=w344, index #4=w343, index #5=w342, index #6=w341, index #7=w340, index #8=w339, index #9=w338, index #10=w337, index #11=w336, index #12=w335, index #13=w334, index #14=w333, index #15=w332, index #16=w301, index #17=w294, index #18=w292, index #19=w291, index #20=w290, index #21=w289, index #22=w288, index #23=w287, index #24=w286, index #25=w285) -> (element #1=w356:u16, element #2=w331:u16, element #3=w330:u16, element #4=w329:u16, element #5=w328:u16, element #6=w327:u16, element #7=w317:u16, element #8=w316:u16, element #9=w312:u16, element #10=w311:u16, element #11=w310:u16, element #12=w309:u16, element #13=w308:u16, element #14=w303:u16, element #15=w302:u16, element #16=w295:u16, element #17=w293:u16, element #18=w284:u16, element #19=w283:u16, element #20=w282:u16, element #21=w281:u16, element #22=w280:u16, element #23=w279:u16, element #24=w278:u16, element #25=w277:u16)
              n169 = local write "Cue1Param_CueType_Switch"(w282) -> ()
              n170 = local write "Cue1Param_AudioLed_Count_Switch"(w281) -> ()
              n171 = local write "Cue1Param_AudioLed_Probability_Switch"(w280) -> ()
              n172 = local write "Cue1Param_CueType_NS"(w279) -> ()
              n173 = local write "Cue1Param_AudioLed_Count_NS"(w278) -> ()
              n174 = local write "Cue1Param_AudioLed_Probability_NS"(w277) -> ()
              n175 = To Double Precision Float(number=w356) -> (double precision float=w355:dbl)
              n176 = To Double Precision Float(number=w331) -> (double precision float=w353:dbl)
              n177 = To Double Precision Float(number=w329) -> (double precision float=w350:dbl)
              n178 = To Double Precision Float(number=w328) -> (double precision float=w349:dbl)
              n179 = To Double Precision Float(number=w327) -> (double precision float=w351:dbl)
              n180 = To Double Precision Float(number=w317) -> (double precision float=w322:dbl)
              n181 = To Double Precision Float(number=w316) -> (double precision float=w318:dbl)
              n182 = To Double Precision Float(number=w312) -> (double precision float=w323:dbl)
              n183 = To Double Precision Float(number=w310) -> (double precision float=w325:dbl)
              n184 = To Double Precision Float(number=w309) -> (double precision float=w326:dbl)
              n185 = To Double Precision Float(number=w308) -> (double precision float=w324:dbl)
              n186 = To Double Precision Float(number=w303) -> (double precision float=w306:dbl)
              n187 = To Double Precision Float(number=w302) -> (double precision float=w307:dbl)
              n188 = To Double Precision Float(number=w295) -> (double precision float=w300:dbl)
              n189 = To Double Precision Float(number=w293) -> (double precision float=w299:dbl)
              n190 = local write "SolenoidProbability_L"(w284) -> ()
              n191 = local write "SolenoidProbability_R"(w283) -> ()
              n192 = Divide(x=w355, y=w296) -> (x/y=w354:dbl)
              n193 = Divide(x=w353, y=w296) -> (x/y=w352:dbl)
              n194 = Divide(x=w350, y=w296) -> (x/y=w347:dbl)
              n195 = Divide(x=w349, y=w296) -> (x/y=w346:dbl)
              n196 = Divide(x=w351, y=w296) -> (x/y=w348:dbl)
              n197 = Divide(x=w322, y=w296) -> (x/y=w320:dbl)
              n198 = Divide(x=w318, y=w296) -> (x/y=w319:dbl)
              n199 = Divide(x=w323, y=w296) -> (x/y=w321:dbl)
              n200 = Divide(x=w325, y=w296) -> (x/y=w315:dbl)
              n201 = Divide(x=w326, y=w296) -> (x/y=w314:dbl)
              n202 = Divide(x=w324, y=w296) -> (x/y=w313:dbl)
              n203 = Divide(x=w306, y=w296) -> (x/y=w305:dbl)
              n204 = Divide(x=w307, y=w296) -> (x/y=w304:dbl)
              n205 = Divide(x=w300, y=w296) -> (x/y=w298:dbl)
              n206 = Divide(x=w299, y=w296) -> (x/y=w297:dbl)
              n207 = local write "FPGA_count2ms"(w354) -> ()
              n208 = local write "Laser_Freq_l1"(w352) -> ()
              n209 = local write "Laser_duration_l1"(w330) -> ()
              n210 = local write "Laser_Tpeak_l1"(w347) -> ()
              n211 = local write "Laser_Tshutter_l1"(w346) -> ()
              n212 = local write "Laser_power_min_l1"(w348) -> ()
              n213 = local write "Laser_power_max_l1"(w320) -> ()
              n214 = local write "Laser_power_step_l1"(w319) -> ()
              n215 = local write "Laser_Freq_l2"(w321) -> ()
              n216 = local write "Laser_duration_l2"(w311) -> ()
              n217 = local write "Laser_Tpeak_l2"(w315) -> ()
              n218 = local write "Laser_Tshutter_l2"(w314) -> ()
              n219 = local write "Laser_power_min_l2"(w313) -> ()
              n220 = local write "Laser_power_max_l2"(w305) -> ()
              n221 = local write "Laser_power_step_l2"(w304) -> ()
              n222 = local write "CueLed_Freq"(w298) -> ()
              n223 = local write "CueLed_Tpeak"(w297) -> ()
            }
            frame "UploadSettings_dataLC_1" {
              # "Cue1_delayOpt_NonSwitch"
              # "ENL1_delayOpt_NonSwitch"
              # "Cue1_delayOpt_Switch"
              # "ENL1_delayOpt_Switch"
              # "Count"
              # "Tdelay"
              # "Prob"
              # "OnOff"
              # "Block"
              # "Count"
              # "Tdelay"
              # "Prob"
              # "OnOff"
              # "Block"
              # "Count"
              # "Tdelay"
              # "Prob"
              # "OnOff"
              # "Block"
              # "ENL1 Switch"
              # "Cue1 NonSwitch"
              # "Cue1 Switch"
              # "ENL1 NonSwitch"
              # "Count"
              # "Tdelay"
              # "Prob"
              # "OnOff"
              # "Block"
              n224 = call "myRIO_BRig_RT_dataLC_ENL1_OnOff_Switch_l1.vi"() -> ("output_ENL1_OnOff_Switch_l1"=w412:i32)  [unwired: 11 in]
              n225 = call "myRIO_BRig_RT_dataLC_ENL1_Tdelay_Switch_l1.vi"() -> ("output_ENL1_Tdelay_Switch_l1"=w411:i32)  [unwired: 11 in]
              n226 = call "myRIO_BRig_RT_dataLC_ENL1_Block_Switch_l1.vi"() -> ("output_ENL1_Block_Switch_l1"=w410:i32)  [unwired: 11 in]
              n227 = call "myRIO_BRig_RT_dataLC_ENL1_Count_Switch_l1.vi"() -> ("output_ENL1_Count_Switch_l1"=w409:i32)  [unwired: 11 in]
              n228 = call "myRIO_BRig_RT_dataLC_ENL1_Probability_Switch_l1.vi"() -> ("output_ENL1_Probability_Switch_l1"=w408:i32)  [unwired: 11 in]
              n229 = call "myRIO_BRig_RT_dataLC_ENL1_OnOff_NS_l1.vi"() -> ("output_ENL1_OnOff_NS_l1"=w407:i32)  [unwired: 11 in]
              n230 = call "myRIO_BRig_RT_dataLC_ENL1_Tdelay_NS_l1.vi"() -> ("output_ENL1_Tdelay_NS_l1"=w406:i32)  [unwired: 11 in]
              n231 = call "myRIO_BRig_RT_dataLC_ENL1_Block_NS_l1.vi"() -> ("output_ENL1_All_Block"=w405:i32)  [unwired: 11 in]
              n232 = call "myRIO_BRig_RT_dataLC_ENL1_Count_NS_l1.vi"() -> ("output_ENL1_Count_NS_l1"=w404:i32)  [unwired: 11 in]
              n233 = call "myRIO_BRig_RT_dataLC_ENL1_Probability_NS_l1.vi"() -> ("output_ENL1_Probability_NS_l1"=w403:i32)  [unwired: 11 in]
              n234 = call "myRIO_BRig_RT_dataLC_Cue1_OnOff_Switch_l1.vi"() -> ("output_Cue1_OnOff_Switch_l1"=w402:i32)  [unwired: 11 in]
              n235 = call "myRIO_BRig_RT_dataLC_Cue1_Tdelay_Switch_l1.vi"() -> ("output_Cue1_Tdelay_Switch_l1"=w401:i32)  [unwired: 11 in]
              n236 = call "myRIO_BRig_RT_dataLC_Cue1_Block_Switch_l1.vi"() -> ("output_Cue1_Block_Switch_l1"=w400:i32)  [unwired: 11 in]
              n237 = call "myRIO_BRig_RT_dataLC_Cue1_Count_Switch_l1.vi"() -> ("output_Cue1_Count_Switch_l1"=w399:i32)  [unwired: 11 in]
              n238 = call "myRIO_BRig_RT_dataLC_Cue1_Probability_Switch_l1.vi"() -> ("output_Cue1_Probability_Switch_l1"=w398:i32)  [unwired: 11 in]
              n239 = call "myRIO_BRig_RT_dataLC_Cue1_OnOff_NS_l1.vi"() -> ("output_Cue1_OnOff_NS_l1"=w397:i32)  [unwired: 11 in]
              n240 = call "myRIO_BRig_RT_dataLC_Cue1_Tdelay_NS_l1.vi"() -> ("output_Cue1_Tdelay_NS_l1"=w396:i32)  [unwired: 11 in]
              n241 = call "myRIO_BRig_RT_dataLC_Cue1_Block_NS_l1.vi"() -> ("output_Cue1_Block_NS_l1"=w395:i32)  [unwired: 11 in]
              n242 = call "myRIO_BRig_RT_dataLC_Cue1_Count_NS_l1.vi"() -> ("output_Cue1_Count_NS_l1"=w394:i32)  [unwired: 11 in]
              n243 = call "myRIO_BRig_RT_dataLC_Cue1_Probability_NS_l1.vi"() -> ("output_Cue1_l1_All_Probability"=w393:i32)  [unwired: 11 in]
              n244 = call "myRIO_BRig_RT_dataLC_ENL1_delayOpt_Switch_l1.vi"() -> ("output_ENL1_delayOpt_Switch_l1"=w372:i32)  [unwired: 11 in]
              n245 = call "myRIO_BRig_RT_dataLC_ENL1_delayOpt_NS_l1.vi"() -> ("output_ENL1_delayOpt_NS_l1"=w371:i32)  [unwired: 11 in]
              n246 = call "myRIO_BRig_RT_dataLC_Cue1_delayOpt_Switch_l1.vi"() -> ("output_Cue1_delayOpt_Switch_l1"=w370:i32)  [unwired: 11 in]
              n247 = call "myRIO_BRig_RT_dataLC_Cue1_delayOpt_NS_l1.vi"() -> ("output_Cue1_delayOpt_NS_l1"=w369:i32)  [unwired: 11 in]
              n248 = Index Array(array=w414, index #1=w412, index #2=w411, index #3=w410, index #4=w409, index #5=w408, index #6=w407, index #7=w406, index #8=w405, index #9=w404, index #10=w403, index #11=w402, index #12=w401, index #13=w400, index #14=w399, index #15=w398, index #16=w397, index #17=w396, index #18=w395, index #19=w394, index #20=w393, index #21=w372, index #22=w371, index #23=w370, index #24=w369) -> (element #1=w392:u16, element #2=w391:u16, element #3=w390:u16, element #4=w389:u16, element #5=w388:u16, element #6=w387:u16, element #7=w386:u16, element #8=w385:u16, element #9=w384:u16, element #10=w383:u16, element #11=w382:u16, element #12=w381:u16, element #13=w380:u16, element #14=w379:u16, element #15=w378:u16, element #16=w377:u16, element #17=w376:u16, element #18=w375:u16, element #19=w374:u16, element #20=w373:u16, element #21=w364:u16, element #22=w363:u16, element #23=w362:u16, element #24=w361:u16)
              n249 = Not Equal To 0?(x=w392) -> (x != 0?=w416:bool)
              n250 = Not Equal To 0?(x=w387) -> (x != 0?=w415:bool)
              n251 = Not Equal To 0?(x=w382) -> (x != 0?=w418:bool)
              n252 = Not Equal To 0?(x=w377) -> (x != 0?=w417:bool)
              n253 = Not Equal To 0?(x=w364) -> (x != 0?=w366:bool)
              n254 = Not Equal To 0?(x=w363) -> (x != 0?=w367:bool)
              n255 = Not Equal To 0?(x=w362) -> (x != 0?=w368:bool)
              n256 = Not Equal To 0?(x=w361) -> (x != 0?=w365:bool)
              n257 = local write "LC_ENL1_OnOff_Switch_l1"(w416) -> ()
              n258 = local write "LC_ENL1_Tdelay_Switch_l1"(w391) -> ()
              n259 = local write "LC_ENL1_Block_Switch_l1"(w390) -> ()
              n260 = local write "LC_ENL1_Count_Switch_l1"(w389) -> ()
              n261 = local write "LC_ENL1_Probability_Switch_l1"(w388) -> ()
              n262 = local write "LC_ENL1_OnOff_NS_l1"(w415) -> ()
              n263 = local write "LC_ENL1_Tdelay_NS_l1"(w386) -> ()
              n264 = local write "LC_ENL1_Block_NS_l1"(w385) -> ()
              n265 = local write "LC_ENL1_Count_NS_l1"(w384) -> ()
              n266 = local write "LC_ENL1_Probability_NS_l1"(w383) -> ()
              n267 = local write "LC_Cue1_OnOff_Switch_l1"(w418) -> ()
              n268 = local write "LC_Cue1_Tdelay_Switch_l1"(w381) -> ()
              n269 = local write "LC_Cue1_Block_Switch_l1"(w380) -> ()
              n270 = local write "LC_Cue1_Count_Switch_l1"(w379) -> ()
              n271 = local write "LC_Cue1_Probability_Switch_l1"(w378) -> ()
              n272 = local write "LC_Cue1_OnOff_NS_l1"(w417) -> ()
              n273 = local write "LC_Cue1_Tdelay_NS_l1"(w376) -> ()
              n274 = local write "LC_Cue1_Block_NS_l1"(w375) -> ()
              n275 = local write "LC_Cue1_Count_NS_l1"(w374) -> ()
              n276 = local write "LC_Cue1_Probability_NS_l1"(w373) -> ()
              n277 = local write "LC_ENL1_delayOpt_Switch_l1"(w366) -> ()
              n278 = local write "LC_ENL1_delayOpt_NS_l1"(w367) -> ()
              n279 = local write "LC_Cue1_delayOpt_Switch_l1"(w368) -> ()
              n280 = local write "LC_Cue1_delayOpt_NS_l1"(w365) -> ()
            }
            frame "UploadSettings_dataLC_3" {
              # "Cue1_delayOpt_NonSwitch"
              # "ENL1_delayOpt_NonSwitch"
              # "Cue1_delayOpt_Switch"
              # "ENL1_delayOpt_Switch"
              # "Count"
              # "Tdelay"
              # "Prob"
              # "OnOff"
              # "Block"
              # "Count"
              # "Tdelay"
              # "Prob"
              # "OnOff"
              # "Block"
              # "Count"
              # "Tdelay"
              # "Prob"
              # "OnOff"
              # "Block"
              # "ENL1 Switch"
              # "Cue1 NonSwitch"
              # "Cue1 Switch"
              # "ENL1 NonSwitch"
              # "Count"
              # "Tdelay"
              # "Prob"
              # "OnOff"
              # "Block"
              n281 = call "myRIO_BRig_RT_dataLC_ENL1_OnOff_Switch_l2.vi"() -> ("output_ENL1_OnOff_Switch_l2"=w439:i32)  [unwired: 11 in]
              n282 = call "myRIO_BRig_RT_dataLC_ENL1_Tdelay_Switch_l2.vi"() -> ("output_ENL1_Tdelay_Switch_l2"=w440:i32)  [unwired: 11 in]
              n283 = call "myRIO_BRig_RT_dataLC_ENL1_Block_Switch_l2.vi"() -> ("output_ENL1_Block_Switch_l2"=w441:i32)  [unwired: 11 in]
              n284 = call "myRIO_BRig_RT_dataLC_ENL1_Count_Switch_l2.vi"() -> ("output_ENL1_Count_Switch_l2"=w442:i32)  [unwired: 11 in]
              n285 = call "myRIO_BRig_RT_dataLC_ENL1_Probability_Switch_l2.vi"() -> ("output_ENL1_Probability_Switch_l2"=w443:i32)  [unwired: 11 in]
              n286 = call "myRIO_BRig_RT_dataLC_ENL1_OnOff_NS_l2.vi"() -> ("output_ENL1_OnOff_NS_l2"=w434:i32)  [unwired: 11 in]
              n287 = call "myRIO_BRig_RT_dataLC_ENL1_Tdelay_NS_l2.vi"() -> ("output_ENL1_Tdelay_NS_l2"=w435:i32)  [unwired: 11 in]
              n288 = call "myRIO_BRig_RT_dataLC_ENL1_Block_NS_l2.vi"() -> ("output_ENL1_Block_NS_l2"=w436:i32)  [unwired: 11 in]
              n289 = call "myRIO_BRig_RT_dataLC_ENL1_Count_NS_l2.vi"() -> ("output_ENL1_Count_NS_l2"=w437:i32)  [unwired: 11 in]
              n290 = call "myRIO_BRig_RT_dataLC_ENL1_Probability_NS_l2.vi"() -> ("output_ENL1_Probability_NS_l2"=w438:i32)  [unwired: 11 in]
              n291 = call "myRIO_BRig_RT_dataLC_Cue1_OnOff_Switch_l2.vi"() -> ("output_Cue1_OnOff_Switch_l2"=w429:i32)  [unwired: 11 in]
              n292 = call "myRIO_BRig_RT_dataLC_Cue1_Tdelay_Switch_l2.vi"() -> ("output_Cue1_Tdelay_Switch_l2"=w430:i32)  [unwired: 11 in]
              n293 = call "myRIO_BRig_RT_dataLC_Cue1_Block_Switch_l2.vi"() -> ("output_Cue1_Block_Switch_l2"=w431:i32)  [unwired: 11 in]
              n294 = call "myRIO_BRig_RT_dataLC_Cue1_Count_Switch_l2.vi"() -> ("output_Cue1_Count_Switch_l2"=w432:i32)  [unwired: 11 in]
              n295 = call "myRIO_BRig_RT_dataLC_Cue1_Probability_Switch_l2.vi"() -> ("output_Cue1_l2_First_Probability"=w433:i32)  [unwired: 11 in]
              n296 = call "myRIO_BRig_RT_dataLC_Cue1_OnOff_NS_l2.vi"() -> ("output_Cue1_OnOff_NS_l2"=w424:i32)  [unwired: 11 in]
              n297 = call "myRIO_BRig_RT_dataLC_Cue1_Tdelay_NS_l2.vi"() -> ("output_Cue1_Tdelay_NS_l2"=w425:i32)  [unwired: 11 in]
              n298 = call "myRIO_BRig_RT_dataLC_Cue1_Block_NS_l2.vi"() -> ("output_Cue1_Block_NS_l2"=w426:i32)  [unwired: 11 in]
              n299 = call "myRIO_BRig_RT_dataLC_Cue1_Count_NS_l2.vi"() -> ("output_Cue1_Count_NS_l2"=w427:i32)  [unwired: 11 in]
              n300 = call "myRIO_BRig_RT_dataLC_Cue1_Probability_NS_l2.vi"() -> ("output_Cue1_l2_All_Probability"=w428:i32)  [unwired: 11 in]
              n301 = call "myRIO_BRig_RT_dataLC_ENL1_delayOpt_Switch_l2.vi"() -> ("output_ENL1_delayOpt_Switch_l2"=w420:i32)  [unwired: 11 in]
              n302 = call "myRIO_BRig_RT_dataLC_ENL1_delayOpt_NS_l2.vi"() -> ("output_ENL1_delayOpt_NS_l2"=w421:i32)  [unwired: 11 in]
              n303 = call "myRIO_BRig_RT_dataLC_Cue1_delayOpt_Switch_l2.vi"() -> ("output_Cue1_delayOpt_Switch_l2"=w422:i32)  [unwired: 11 in]
              n304 = call "myRIO_BRig_RT_dataLC_Cue1_delayOpt_NS_l2.vi"() -> ("output_Cue1_delayOpt_NS_l2"=w423:i32)  [unwired: 11 in]
              n305 = Index Array(array=w473, index #1=w439, index #2=w440, index #3=w441, index #4=w442, index #5=w443, index #6=w434, index #7=w435, index #8=w436, index #9=w437, index #10=w438, index #11=w429, index #12=w430, index #13=w431, index #14=w432, index #15=w433, index #16=w424, index #17=w425, index #18=w426, index #19=w427, index #20=w428, index #21=w420, index #22=w421, index #23=w422, index #24=w423) -> (element #1=w471:u16, element #2=w470:u16, element #3=w469:u16, element #4=w468:u16, element #5=w467:u16, element #6=w466:u16, element #7=w465:u16, element #8=w464:u16, element #9=w463:u16, element #10=w462:u16, element #11=w461:u16, element #12=w460:u16, element #13=w459:u16, element #14=w458:u16, element #15=w457:u16, element #16=w456:u16, element #17=w455:u16, element #18=w454:u16, element #19=w453:u16, element #20=w452:u16, element #21=w447:u16, element #22=w446:u16, element #23=w445:u16, element #24=w444:u16)
              n306 = Not Equal To 0?(x=w471) -> (x != 0?=w475:bool)
              n307 = Not Equal To 0?(x=w466) -> (x != 0?=w474:bool)
              n308 = Not Equal To 0?(x=w461) -> (x != 0?=w477:bool)
              n309 = Not Equal To 0?(x=w456) -> (x != 0?=w476:bool)
              n310 = Not Equal To 0?(x=w447) -> (x != 0?=w449:bool)
              n311 = Not Equal To 0?(x=w446) -> (x != 0?=w450:bool)
              n312 = Not Equal To 0?(x=w445) -> (x != 0?=w451:bool)
              n313 = Not Equal To 0?(x=w444) -> (x != 0?=w448:bool)
              n314 = local write "LC_ENL1_OnOff_Switch_l2"(w475) -> ()
              n315 = local write "LC_ENL1_Tdelay_Switch_l2"(w470) -> ()
              n316 = local write "LC_ENL1_Block_Switch_l2"(w469) -> ()
              n317 = local write "LC_ENL1_Count_Switch_l2"(w468) -> ()
              n318 = local write "LC_ENL1_Probability_Switch_l2"(w467) -> ()
              n319 = local write "LC_ENL1_OnOff_NS_l2"(w474) -> ()
              n320 = local write "LC_ENL1_Tdelay_NS_l2"(w465) -> ()
              n321 = local write "LC_ENL1_Block_NS_l2"(w464) -> ()
              n322 = local write "LC_ENL1_Count_NS_l2"(w463) -> ()
              n323 = local write "LC_ENL1_Probability_NS_l2"(w462) -> ()
              n324 = local write "LC_Cue1_OnOff_Switch_l2"(w477) -> ()
              n325 = local write "LC_Cue1_Tdelay_Switch_l2"(w460) -> ()
              n326 = local write "LC_Cue1_Block_Switch_l2"(w459) -> ()
              n327 = local write "LC_Cue1_Count_Switch_l2"(w458) -> ()
              n328 = local write "LC_Cue1_Probability_Switch_l2"(w457) -> ()
              n329 = local write "LC_Cue1_OnOff_NS_l2"(w476) -> ()
              n330 = local write "LC_Cue1_Tdelay_NS_l2"(w455) -> ()
              n331 = local write "LC_Cue1_Block_NS_l2"(w454) -> ()
              n332 = local write "LC_Cue1_Count_NS_l2"(w453) -> ()
              n333 = local write "LC_Cue1_Probability_NS_l2"(w452) -> ()
              n334 = local write "LC_ENL1_delayOpt_Switch_l2"(w449) -> ()
              n335 = local write "LC_ENL1_delayOpt_NS_l2"(w450) -> ()
              n336 = local write "LC_Cue1_delayOpt_Switch_l2"(w451) -> ()
              n337 = local write "LC_Cue1_delayOpt_NS_l2"(w448) -> ()
            }
            frame "UploadSettings_dataLC_2" {
              # "Count"
              # "Tdelay"
              # "Prob"
              # "OnOff"
              # "Block"
              # "Selection NonSwitch"
              # "Count"
              # "Tdelay"
              # "Prob"
              # "OnOff"
              # "Block"
              # "Selection Switch"
              # "Trial"
              # "Tdelay"
              # "Prob"
              # "OnOff"
              # "Block"
              # "Wrong"
              # "Reward"
              # "Trial"
              # "Tdelay"
              # "Prob"
              # "OnOff"
              # "Block"
              n338 = call "myRIO_BRig_RT_dataLC_Reward_OnOff_l1.vi"() -> ("output_Reward_OnOff_l1"=w520:i32)  [unwired: 11 in]
              n339 = call "myRIO_BRig_RT_dataLC_Reward_Tdelay_l1.vi"() -> ("output_Reward_Tdelay_l1"=w519:i32)  [unwired: 11 in]
              n340 = call "myRIO_BRig_RT_dataLC_Reward_Block_l1.vi"() -> ("output_Reward_Block_l1"=w518:i32)  [unwired: 11 in]
              n341 = call "myRIO_BRig_RT_dataLC_Reward_Trial_l1.vi"() -> ("output_Reward_Trial_l1"=w517:i32)  [unwired: 11 in]
              n342 = call "myRIO_BRig_RT_dataLC_Reward_Probability_l1.vi"() -> ("output_Reward_Probability_l1"=w516:i32)  [unwired: 11 in]
              n343 = call "myRIO_BRig_RT_dataLC_Wrong_OnOff_l1.vi"() -> ("output_Wrong_OnOff_l1"=w509:i32)  [unwired: 11 in]
              n344 = call "myRIO_BRig_RT_dataLC_Wrong_Tdelay_l1.vi"() -> ("output_Wrong_Tdelay_l1"=w508:i32)  [unwired: 11 in]
              n345 = call "myRIO_BRig_RT_dataLC_Wrong_Block_l1.vi"() -> ("output_Wrong_Block_l1"=w507:i32)  [unwired: 11 in]
              n346 = call "myRIO_BRig_RT_dataLC_Wrong_Trial_l1.vi"() -> ("output_Wrong_Trial_l1"=w506:i32)  [unwired: 11 in]
              n347 = call "myRIO_BRig_RT_dataLC_Wrong_Probability_l1.vi"() -> ("output_Wrong_Probability_l1"=w505:i32)  [unwired: 11 in]
              n348 = call "myRIO_BRig_RT_dataLC_Selection_OnOff_Switch_l1.vi"() -> ("output_Selection_OnOff_Switch_l1"=w500:i32)  [unwired: 11 in]
              n349 = call "myRIO_BRig_RT_dataLC_Selection_Tdelay_Switch_l1.vi"() -> ("output_Selection_Tdelay_Switch_l1"=w499:i32)  [unwired: 11 in]
              n350 = call "myRIO_BRig_RT_dataLC_Selection_Block_Switch_l1.vi"() -> ("output_Selection_Block_Switch_l1"=w498:i32)  [unwired: 11 in]
              n351 = call "myRIO_BRig_RT_dataLC_Selection_Count_Switch_l1.vi"() -> ("output_Selection_Count_Switch_l1"=w497:i32)  [unwired: 11 in]
              n352 = call "myRIO_BRig_RT_dataLC_Selection_Probability_Switch_l1.vi"() -> ("output_Selection_Probability_Switch_l1"=w496:i32)  [unwired: 11 in]
              n353 = call "myRIO_BRig_RT_dataLC_Selection_OnOff_NS_l1.vi"() -> ("output_Selection_OnOff_NS_l1"=w495:i32)  [unwired: 11 in]
              n354 = call "myRIO_BRig_RT_dataLC_Selection_Tdelay_NS_l1.vi"() -> ("output_Selection_Tdelay_NS_l1"=w494:i32)  [unwired: 11 in]
              n355 = call "myRIO_BRig_RT_dataLC_Selection_Block_NS_l1.vi"() -> ("output_Selection_Block_NS_l1"=w493:i32)  [unwired: 11 in]
              n356 = call "myRIO_BRig_RT_dataLC_Selection_Count_NS_l1.vi"() -> ("output_Selection_Count_NS_l1"=w492:i32)  [unwired: 11 in]
              n357 = call "myRIO_BRig_RT_dataLC_Selection_Probability_NS_l1.vi"() -> ("output_Selection_Probability_NS_l1"=w491:i32)  [unwired: 11 in]
              n358 = Index Array(array=w521, index #1=w520, index #2=w519, index #3=w518, index #4=w517, index #5=w516, index #6=w509, index #7=w508, index #8=w507, index #9=w506, index #10=w505, index #11=w500, index #12=w499, index #13=w498, index #14=w497, index #15=w496, index #16=w495, index #17=w494, index #18=w493, index #19=w492, index #20=w491) -> (element #1=w515:u16, element #2=w514:u16, element #3=w513:u16, element #4=w512:u16, element #5=w511:u16, element #6=w510:u16, element #7=w504:u16, element #8=w503:u16, element #9=w502:u16, element #10=w501:u16, element #11=w488:u16, element #12=w487:u16, element #13=w486:u16, element #14=w485:u16, element #15=w484:u16, element #16=w483:u16, element #17=w482:u16, element #18=w481:u16, element #19=w480:u16, element #20=w479:u16)
              n359 = Not Equal To 0?(x=w515) -> (x != 0?=w523:bool)
              n360 = Not Equal To 0?(x=w510) -> (x != 0?=w522:bool)
              n361 = Not Equal To 0?(x=w488) -> (x != 0?=w490:bool)
              n362 = Not Equal To 0?(x=w483) -> (x != 0?=w489:bool)
              n363 = local write "LC_Reward_OnOff_l1"(w523) -> ()
              n364 = local write "LC_Reward_Tdelay_l1"(w514) -> ()
              n365 = local write "LC_Reward_Block_l1"(w513) -> ()
              n366 = local write "LC_Reward_Trial_l1"(w512) -> ()
              n367 = local write "LC_Reward_Probability_l1"(w511) -> ()
              n368 = local write "LC_Wrong_OnOff_l1"(w522) -> ()
              n369 = local write "LC_Wrong_Tdelay_l1"(w504) -> ()
              n370 = local write "LC_Wrong_Block_l1"(w503) -> ()
              n371 = local write "LC_Wrong_Trial_l1"(w502) -> ()
              n372 = local write "LC_Wrong_Probability_l1"(w501) -> ()
              n373 = local write "LC_Sel_OnOff_Switch_l1"(w490) -> ()
              n374 = local write "LC_Sel_Tdelay_Switch_l1"(w487) -> ()
              n375 = local write "LC_Sel_Block_Switch_l1"(w486) -> ()
              n376 = local write "LC_Sel_Count_Switch_l1"(w485) -> ()
              n377 = local write "LC_Sel_Probability_Switch_l1"(w484) -> ()
              n378 = local write "LC_Sel_OnOff_NS_l1"(w489) -> ()
              n379 = local write "LC_Sel_Tdelay_NS_l1"(w482) -> ()
              n380 = local write "LC_Sel_Block_NS_l1"(w481) -> ()
              n381 = local write "LC_Sel_Count_NS_l1"(w480) -> ()
              n382 = local write "LC_Sel_Probability_NS_l1"(w479) -> ()
            }
            frame "UploadSettings_dataLC_4" {
              # "Count"
              # "Tdelay"
              # "Prob"
              # "OnOff"
              # "Block"
              # "Selection NonSwitch"
              # "Count"
              # "Tdelay"
              # "Prob"
              # "OnOff"
              # "Block"
              # "Selection Switch"
              # "Trial"
              # "Tdelay"
              # "Prob"
              # "OnOff"
              # "Block"
              # "Wrong"
              # "Reward"
              # "Trial"
              # "Tdelay"
              # "Prob"
              # "OnOff"
              # "Block"
              n383 = call "myRIO_BRig_RT_dataLC_Reward_OnOff_l2.vi"() -> ("output_Reward_OnOff_l2"=w531:i32)  [unwired: 11 in]
              n384 = call "myRIO_BRig_RT_dataLC_Reward_Tdelay_l2.vi"() -> ("output_Reward_Tdelay_l2"=w532:i32)  [unwired: 11 in]
              n385 = call "myRIO_BRig_RT_dataLC_Reward_Block_l2.vi"() -> ("output_Reward_Block_l2"=w533:i32)  [unwired: 11 in]
              n386 = call "myRIO_BRig_RT_dataLC_Reward_Trial_l2.vi"() -> ("output_Reward_Trial_l2"=w534:i32)  [unwired: 11 in]
              n387 = call "myRIO_BRig_RT_dataLC_Reward_Probability_l2.vi"() -> ("output_Reward_Probability_l2"=w535:i32)  [unwired: 11 in]
              n388 = call "myRIO_BRig_RT_dataLC_Wrong_OnOff_l2.vi"() -> ("output_Wrong_OnOff_l2"=w526:i32)  [unwired: 11 in]
              n389 = call "myRIO_BRig_RT_dataLC_Wrong_Tdelay_l2.vi"() -> ("output_Wrong_Tdelay_l2"=w527:i32)  [unwired: 11 in]
              n390 = call "myRIO_BRig_RT_dataLC_Wrong_Block_l2.vi"() -> ("output_Wrong_Block_l2"=w528:i32)  [unwired: 11 in]
              n391 = call "myRIO_BRig_RT_dataLC_Wrong_Trial_l2.vi"() -> ("output_Wrong_Trial_l2"=w529:i32)  [unwired: 11 in]
              n392 = call "myRIO_BRig_RT_dataLC_Wrong_Probability_l2.vi"() -> ("output_Wrong_Probability_l2"=w530:i32)  [unwired: 11 in]
              n393 = call "myRIO_BRig_RT_dataLC_Selection_OnOff_Switch_l2.vi"() -> ("output_Selection_OnOff_Switch_l2"=w541:i32)  [unwired: 11 in]
              n394 = call "myRIO_BRig_RT_dataLC_Selection_Tdelay_Switch_l2.vi"() -> ("output_Selection_Tdelay_Switch_l2"=w542:i32)  [unwired: 11 in]
              n395 = call "myRIO_BRig_RT_dataLC_Selection_Block_Switch_l2.vi"() -> ("output_Selection_Block_Switch_l2"=w543:i32)  [unwired: 11 in]
              n396 = call "myRIO_BRig_RT_dataLC_Selection_Count_Switch_l2.vi"() -> ("output_Selection_Count_Switch_l2"=w544:i32)  [unwired: 11 in]
              n397 = call "myRIO_BRig_RT_dataLC_Selection_Probability_Switch_l2.vi"() -> ("output_Selection_Probability_Switch_l1"=w545:i32)  [unwired: 11 in]
              n398 = call "myRIO_BRig_RT_dataLC_Selection_OnOff_NS_l2.vi"() -> ("output_Selection_OnOff_NS_l2"=w536:i32)  [unwired: 11 in]
              n399 = call "myRIO_BRig_RT_dataLC_Selection_Tdelay_NS_l2.vi"() -> ("output_Selection_Tdelay_NS_l2"=w537:i32)  [unwired: 11 in]
              n400 = call "myRIO_BRig_RT_dataLC_Selection_Block_NS_l2.vi"() -> ("output_Selection_Block_NS_l2"=w538:i32)  [unwired: 11 in]
              n401 = call "myRIO_BRig_RT_dataLC_Selection_Count_NS_l2.vi"() -> ("output_Selection_Count_NS_l2"=w539:i32)  [unwired: 11 in]
              n402 = call "myRIO_BRig_RT_dataLC_Selection_Probability_NS_l2.vi"() -> ("output_Selection_Probability_NS_l2"=w540:i32)  [unwired: 11 in]
              n403 = Index Array(array=w568, index #1=w531, index #2=w532, index #3=w533, index #4=w534, index #5=w535, index #6=w526, index #7=w527, index #8=w528, index #9=w529, index #10=w530, index #11=w541, index #12=w542, index #13=w543, index #14=w544, index #15=w545, index #16=w536, index #17=w537, index #18=w538, index #19=w539, index #20=w540) -> (element #1=w567:u16, element #2=w566:u16, element #3=w565:u16, element #4=w564:u16, element #5=w563:u16, element #6=w562:u16, element #7=w561:u16, element #8=w560:u16, element #9=w559:u16, element #10=w558:u16, element #11=w555:u16, element #12=w554:u16, element #13=w553:u16, element #14=w552:u16, element #15=w551:u16, element #16=w550:u16, element #17=w549:u16, element #18=w548:u16, element #19=w547:u16, element #20=w546:u16)
              n404 = Not Equal To 0?(x=w567) -> (x != 0?=w570:bool)
              n405 = Not Equal To 0?(x=w562) -> (x != 0?=w569:bool)
              n406 = Not Equal To 0?(x=w555) -> (x != 0?=w557:bool)
              n407 = Not Equal To 0?(x=w550) -> (x != 0?=w556:bool)
              n408 = local write "LC_Reward_OnOff_l2"(w570) -> ()
              n409 = local write "LC_Reward_Tdelay_l2"(w566) -> ()
              n410 = local write "LC_Reward_Block_l2"(w565) -> ()
              n411 = local write "LC_Reward_Trial_l2"(w564) -> ()
              n412 = local write "LC_Reward_Probability_l2"(w563) -> ()
              n413 = local write "LC_Wrong_OnOff_l2"(w569) -> ()
              n414 = local write "LC_Wrong_Tdelay_l2"(w561) -> ()
              n415 = local write "LC_Wrong_Block_l2"(w560) -> ()
              n416 = local write "LC_Wrong_Trial_l2"(w559) -> ()
              n417 = local write "LC_Wrong_Probability_l2"(w558) -> ()
              n418 = local write "LC_Sel_OnOff_Switch_l2"(w557) -> ()
              n419 = local write "LC_Sel_Tdelay_Switch_l2"(w554) -> ()
              n420 = local write "LC_Sel_Block_Switch_l2"(w553) -> ()
              n421 = local write "LC_Sel_Count_Switch_l2"(w552) -> ()
              n422 = local write "LC_Sel_Probability_Switch_l2"(w551) -> ()
              n423 = local write "LC_Sel_OnOff_NS_l2"(w556) -> ()
              n424 = local write "LC_Sel_Tdelay_NS_l2"(w549) -> ()
              n425 = local write "LC_Sel_Block_NS_l2"(w548) -> ()
              n426 = local write "LC_Sel_Count_NS_l2"(w547) -> ()
              n427 = local write "LC_Sel_Probability_NS_l2"(w546) -> ()
            }
            frame "UploadSettings_dataMTrig_1" {
              # "Tdelay_R"
              # "Tdelay_L"
              # "Tcycle_R"
              # "Tcycle_L"
              # "RewCalib_nCycle_R"
              # "RewCalib_nCycle_L"
              # "Solenoid"
              # "Laser_Tcycle"
              n428 = call "myRIO_BRig_RT_dataMTrig_Laser_Tcycle.vi"() -> ("output_Laser_Tcycle"=w580:i32)  [unwired: 11 in]
              n429 = call "myRIO_BRig_RT_dataMTrig_Solenoid_RewCalib_nCycle__L.vi"() -> ("output_Solenoid_RewCalib_nCycle__L"=w579:i32)  [unwired: 11 in]
              n430 = call "myRIO_BRig_RT_dataMTrig_Solenoid_RewCalib_nCycle__R.vi"() -> ("output_Solenoid_RewCalib_nCycle__R"=w578:i32)  [unwired: 11 in]
              n431 = call "myRIO_BRig_RT_dataMTrig_Solenoid_Tdelay__L.vi"() -> ("output_Solenoid_Tdelay__L"=w575:i32)  [unwired: 11 in]
              n432 = call "myRIO_BRig_RT_dataMTrig_Solenoid_Tdelay__R.vi"() -> ("output_Solenoid_Tdelay__R"=w574:i32)  [unwired: 11 in]
              n433 = call "myRIO_BRig_RT_dataMTrig_Solenoid_Tcycle__L.vi"() -> ("output_Solenoid_Tcycle__L"=w577:i32)  [unwired: 11 in]
              n434 = call "myRIO_BRig_RT_dataMTrig_Solenoid_Tcycle__R.vi"() -> ("output_Solenoid_Tcycle__R"=w576:i32)  [unwired: 11 in]
              n435 = Index Array(array=w573, index #1=w580, index #2=w579, index #3=w578, index #4=w577, index #5=w576, index #6=w575, index #7=w574) -> (element #1=w587:u16, element #2=w586:u16, element #3=w585:u16, element #4=w584:u16, element #5=w583:u16, element #6=w582:u16, element #7=w581:u16)
              n436 = Replace Array Subset(array=w589, new element #1=w587, index #1=w580, new element #2=w586, index #2=w579, new element #3=w585, index #3=w578, new element #4=w584, index #4=w577, new element #5=w583, index #5=w576, new element #6=w582, index #6=w575, new element #7=w581, index #7=w574) -> (w588:u16[])
              n437 = local write "MTrig_Solenoid_Tcycle__L"(w584) -> ()
              n438 = local write "MTrig_Solenoid_Tcycle__R"(w583) -> ()
              n439 = local write "MTrig_Laser_Tcycle"(w587) -> ()
            }
            frame "Idle" {
              # "There are a number of tasks we need to perform\nwhile idling. To preserve our timing loop, we\nbreak up the IDLE state into smaller states"
              # "Laser_Tcycle"
              # "Audio_Tcycle_R"
              # "Audio_Tcycle_L"
              n440 = local read "Laser_power_min_l1"() -> (w597:dbl)
              n441 = local read "Laser_power_min_l2"() -> (w595:dbl)
              n442 = local read "Audio_Amp__R"() -> (w599:u16)
              n443 = local read "Audio_Amp__L"() -> (w601:u16)
              n444 = local read "Audio_Freq__R"() -> (w598:u8)
              n445 = local read "Audio_Freq__L"() -> (w600:u8)
              n446 = Select(t=myRIO_BRig_RT__Case_NonExp_stateList."SendData" ("Enum"), s="SendData", f=myRIO_BRig_RT__Case_NonExp_stateList."Idle_2" ("Enum")) -> (s? t:f=w606:T1)
              n447 = call "myRIO__convert__Voltage_to_FPGAvalue.vi"("input_voltage"=w597) -> ("output_PortC"=w596:i16)  [unwired: 9 in, 1 out]
              n448 = call "myRIO__convert__Voltage_to_FPGAvalue.vi"("input_voltage"=w595) -> ("output_PortC"=w594:i16)  [unwired: 9 in, 1 out]
              n449 = Select(t=myRIO_BRig_RT__Case_NonExp_stateList."TestConnection" ("Enum"), s="TestConnection", f=w606) -> (s? t:f=w610:T1)
              n450 = xnode "Read/Write Control"("FPGA VI Reference In"=w603, "error in"=w602, "audioAmp_L"=w601, "audioFreq_L_kHz"=w600, "audioAmp_R"=w599, "audioFreq_R_kHz"=w598, "AnaOut_0"=w596, "AnaOut_1"=w594) -> ("error out"=w593:errorcluster)  [unwired: 1 out]
              n451 = call "myRIO_BRig_RT_dataMTrig_Audio_Tcycle__L.vi"() -> ("output_Audio_Tcycle__L"=w617:i32)  [unwired: 11 in]
              n452 = call "myRIO_BRig_RT_dataMTrig_Audio_Tcycle__R.vi"() -> ("output_Audio_Tcycle__R"=w616:i32)  [unwired: 11 in]
              n453 = call "myRIO_BRig_RT_dataMTrig_Laser_Tcycle.vi"() -> ("output_Laser_Tcycle"=w615:i32)  [unwired: 11 in]
              n454 = call "myRIO_BRig_RT_dataMTrig_CueLed_Tcycle.vi"() -> ("output_CueLed_Tcycle"=w592:i32)  [unwired: 11 in]
              n455 = local write "error out"(w593) -> ()
              n456 = local read "Tcycle_Cue_Audio_min"() -> (w605:u16)
              n457 = local read "MTrig_Laser_Tcycle"() -> (w604:u16)
              n458 = local read "Tcycle_Cue_LED_min"() -> (w591:u16)
              n459 = Replace Array Subset(array=w613, new element #1=w605, index #1=w617, new element #2=w605, index #2=w616, new element #3=w604, index #3=w615, new element #4=w591, index #4=w592) -> (w614:u16[])
            }
            frame "Idle_2" {
              w640 = u16 0 ("t")
              # "There are a number of tasks we need to perform\nwhile idling. To preserve our timing loop, we\nbreak up the IDLE state into smaller states"
              # "Ncycles"
              # "Ncycles"
              # "RewCalib"
              # "RewCalib"
              # "Solenoid R"
              # "Solenoid L"
              n460 = local read "MTrig_Laser_Switch"() -> (w633:bool)
              n461 = local read "count_warmup_R"() -> (w639:u16)
              n462 = local read "count_warmup_L"() -> (w644:u16)
              n463 = call "myRIO_BRig_RT_dataMTrig_Solenoid_RewCalib_OnOff__R.vi"() -> ("output_Solenoid_RewCalib_OnOff__R"=w655:i32)  [unwired: 11 in]
              n464 = call "myRIO_BRig_RT_dataMTrig_Solenoid_N__R.vi"() -> ("output_Solenoid_N__R"=w654:i32)  [unwired: 11 in]
              n465 = call "myRIO_BRig_RT_dataMTrig_Solenoid_RewCalib_OnOff__L.vi"() -> ("output_Solenoid_RewCalib_OnOff__L"=w670:i32)  [unwired: 11 in]
              n466 = call "myRIO_BRig_RT_dataMTrig_Solenoid_N__L.vi"() -> ("output_Solenoid_N__L"=w658:i32)  [unwired: 11 in]
              n467 = case shown="False" w633 {
                tunnel: "LR_reward_Event" -> [w676 w680]
                tunnel: "LR_wrong_Event" -> [w675 w679]
                tunnel: "LR_reward_Laser" -> [w674 w678]
                tunnel: "LR_wrong_Laser" -> [w673 w677]
                tunnel: [w676 _] -> w628
                tunnel: [w675 _] -> w627
                tunnel: [w674 _] -> w626
                tunnel: [w673 _] -> w625
                tunnel: [_ w680] -> w624
                tunnel: [_ w679] -> w623
                tunnel: [_ w678] -> w622
                tunnel: [_ w677] -> w621
                frame False {
                }
                frame True {
                }
              }
              n468 = Index Array(array=w661, index #1=w670, index #2=w658, index #3=w655, index #4=w654) -> (element #1=w657:u16, element #2=w652:u16, element #3=w653:u16, element #4=w651:u16)
              n469 = Select(t=w640, s="count_warmup_L_reset", f=w644) -> (s? t:f=→"count_warmup_L":u16)
              n470 = Select(t=w640, s="count_warmup_R_reset", f=w639) -> (s? t:f=→"count_warmup_R":u16)
              n471 = local read "RewCalib_Trig_L"() -> (w650:bool)
              n472 = local read "RewCalib_Trig_R"() -> (w649:bool)
              n473 = Equal To 0?(x=w652) -> (x = 0?=w660:bool)
              n474 = Equal To 0?(x=w651) -> (x = 0?=w659:bool)
              n475 = Not Equal To 0?(x=w653) -> (x != 0?=w671:bool)
              n476 = Not Equal To 0?(x=w657) -> (x != 0?=w672:bool)
              n477 = And(x=w660, y=w659) -> (x .and. y?=w664:bool)
              n478 = Or(x=w650, y=w649) -> (x .or. y?=w665:bool)
              n479 = Not Exclusive Or(1:w672, 2:w650) -> (0:w667:bool)
              n480 = xnode "Read/Write Control"("FPGA VI Reference In"=w619, "error in"=w620, "Left(F)_or_Right(T)"="Left(F)_or_Right(T)", "SelectionState"="SelectionState", "ignoreWrong"="ignoreWrong", "LR_reward_Event_l1"=w628, "LR_wrong_Event_l1"=w627, "LR_reward_Laser_l1"=w626, "LR_wrong_Laser_l1"=w625, "LR_reward_Event_l2"=w624, "LR_wrong_Event_l2"=w623, "LR_reward_Laser_l2"=w622, "LR_wrong_laser_l2"=w621) -> ("error out"=w618:errorcluster, "SelectReward"=→"SelectReward":bool, "SelectWrong"=→"SelectWrong":bool)  [unwired: 1 out]
              n481 = Not Exclusive Or(1:w671, 2:w649) -> (0:w669:bool)
              n482 = And(x=w665, y=w664) -> (x .and. y?=w647:bool)
              n483 = Not(x=w667) -> (.not. x?=w666:bool)
              n484 = Not(x=w669) -> (.not. x?=w668:bool)
              n485 = Or(x=w666, y=w668) -> (x .or. y?=w648:bool)
              n486 = Or(x=w647, y=w648) -> (x .or. y?=w663:bool)
              n487 = local write "error out"(w618) -> ()
              n488 = Select(t=myRIO_BRig_RT__Case_NonExp_stateList."RewardCalibration_pre" ("Enum"), s=w663, f=myRIO_BRig_RT__Case_NonExp_stateList."Idle_3" ("Enum")) -> (s? t:f=w646:T1)
            }
            frame "Idle_3" {
              # "There are a number of tasks we need to perform\nwhile idling. To preserve our timing loop, we\nbreak up the IDLE state into smaller states"
              n489 = local read "Laser_Tshutter_l1"() -> (w699:dbl)
              n490 = local read "Laser_duration_l1"() -> (w698:u16)
              n491 = local read "Laser_Tshutter_l2"() -> (w695:dbl)
              n492 = local read "Laser_duration_l2"() -> (w694:u16)
              n493 = local read "Laser_Tpeak_l1"() -> (w701:dbl)
              n494 = local read "Laser_Tpeak_l2"() -> (w697:dbl)
              n495 = local read "CueLed_Tpeak"() -> (w692:dbl)
              n496 = local read "Laser_Freq_l1"() -> (w700:dbl)
              n497 = local read "Laser_Freq_l2"() -> (w696:dbl)
              n498 = local read "CueLed_Freq"() -> (w691:dbl)
              n499 = local read "FPGA_count2ms"() -> (w693:dbl)
              n500 = To Unsigned Word Integer(number=w693) -> (unsigned 16bit integer=w702:u16)
              n501 = call "myRIO_BRig_RT__calc_laser_FPGA_N.vi"("input_FPGA_ms2count"=w693, "input_Tpeak"=w701, "input_Freq"=w700, "input_Tshutter"=w699, "input_duration"=w698) -> ("output_laser_Npeak"=w690:u32, "output_laser_Nvalley"=w688:u32, "output_laser_Nshutter"=w686:u32, "output_laser_Nduration"=w684:u32)  [unwired: 6 in, 1 out]
              n502 = call "myRIO_BRig_RT__calc_laser_FPGA_N.vi"("input_FPGA_ms2count"=w693, "input_Tpeak"=w697, "input_Freq"=w696, "input_Tshutter"=w695, "input_duration"=w694) -> ("output_laser_Npeak"=w689:u32, "output_laser_Nvalley"=w687:u32, "output_laser_Nshutter"=w685:u32, "output_laser_Nduration"=w683:u32)  [unwired: 6 in, 1 out]
              n503 = call "myRIO_BRig_RT__calc_laser_FPGA_N__CueLed.vi"("input_FPGA_ms2count"=w693, "input_Tpeak"=w692, "input_Freq"=w691) -> ("output_laser_Npeak"=w682:u32, "output_laser_Nvalley"=w681:u32)  [unwired: 11 in]
              n504 = xnode "Read/Write Control"("FPGA VI Reference In"=w707, "error in"=w706, "k1__counter_per_ms"=w702, "LC_nPeak_l1"=w690, "LC_nPeak_l2"=w689, "LC_nValley_l1"=w688, "LC_nValley_l2"=w687, "LC_nShutter_l1"=w686, "LC_nShutter_l2"=w685, "LR_reward_nTotal_l1"=w684, "LR_wrong_nTotal_l1"=w684, "LR_reward_nTotal_l2"=w683, "LR_wrong_nTotal_l2"=w683, "CueLed_nPeak"=w682, "CueLed_nValley"=w681) -> ("error out"=w703:errorcluster)  [unwired: 1 out]
              n505 = local write "error out"(w703) -> ()
            }
            frame "Idle_4" {
              w729 = u8 0 ("f")
              # "There are a number of tasks we need to perform\nwhile idling. To preserve our timing loop, we\nbreak up the IDLE state into smaller states"
              n506 = local read "MTrig_Solenoid_trig__L"() -> (w720:bool)
              n507 = local read "MTrig_Solenoid_trig__R"() -> (w730:bool)
              n508 = local read "warmupType"() -> (w713:u8)
              n509 = local read "warmup"() -> (w722:bool)
              n510 = Not Equal To 0?(x=w713) -> (x != 0?=w712:bool)
              n511 = Not(x=w712) -> (.not. x?=w723:bool)
              n512 = Select(t=u8 1, s=w720, f=w729) -> (s? t:f=w728:u8)
              n513 = Select(t=u8 2, s=w730, f=w729) -> (s? t:f=w727:u8)
              n514 = And(x=w722, y=w723) -> (x .and. y?=w721:bool)
              n515 = And(x=w722, y=w712) -> (x .and. y?=w716:bool)
              n516 = Add(x=w728, y=w727) -> (x+y=w726:u8)
              n517 = case shown="3" w726 {
                tunnel: w725 -> [w733 w737 w770 w801]
                tunnel: [w733 w736 w769 w800] -> w724
                tunnel: w721 -> [_ w735 w768 w799]
                tunnel: [_ TRUE TRUE TRUE] -> w718
                frame 0, Default {
                }
                frame 1 {
                  n518 = case shown="False" w735 {
                    tunnel: w737 -> [w750 w765]
                    tunnel: [w749 w764] -> w736
                    frame True {
                      # "Audio_L"
                      # "Solenoid_L"
                      n519 = call "myRIO_BRig_RT_dataMTrig_Solenoid_N__L.vi"() -> ("output_Solenoid_N__L"=w747:i32)  [unwired: 11 in]
                      n520 = call "myRIO_BRig_RT_dataMTrig_Audio_N__L.vi"() -> ("output_Audio_N__L"=w745:i32)  [unwired: 11 in]
                      n521 = call "myRIO_BRig_RT_dataMTrig_Audio_N__R.vi"() -> ("output_Audio_N__R"=w740:i32)  [unwired: 11 in]
                      n522 = local read "sp_LeftSpout"() -> (w744:u16)
                      n523 = Index Array(array=w750, index #1=w747, index #2=w745, index #3=w740) -> (element #1=w748:u16, element #2=w743:u16, element #3=w742:u16)
                      n524 = Increment(x=w748) -> (x+1=w746:u16)
                      n525 = case shown="2" w744 {
                        tunnel: w743 -> [w753 w756 w758]
                        tunnel: w742 -> [w751 w755 w760]
                        tunnel: [w752 w756 w757] -> w741
                        tunnel: [w751 w754 w759] -> w739
                        frame 0, Default {
                          n526 = Increment(x=w753) -> (x+1=w752:u16)
                        }
                        frame 1 {
                          n527 = Increment(x=w755) -> (x+1=w754:u16)
                        }
                        frame 2 {
                          n528 = Increment(x=w760) -> (x+1=w759:u16)
                          n529 = Increment(x=w758) -> (x+1=w757:u16)
                        }
                      }
                      n530 = Replace Array Subset(array=w750, new element #1=w746, index #1=w747, new element #2=w741, index #2=w745, new element #3=w739, index #3=w740) -> (w749:u16[])
                    }
                    frame False {
                      # "Solenoid_L"
                      n531 = call "myRIO_BRig_RT_dataMTrig_Solenoid_N__L.vi"() -> ("output_Solenoid_N__L"=w762:i32)  [unwired: 11 in]
                      n532 = Index Array(array=w765, index=w762) -> (element=w763:u16)
                      n533 = Increment(x=w763) -> (x+1=w761:u16)
                      n534 = Replace Array Subset(array=w765, new element=w761, index=w762) -> (w764:u16[])
                    }
                  }
                  n535 = local write "MTrig_Solenoid_trig__L"(FALSE) -> ()
                }
                frame 2 {
                  n536 = case shown="True" w768 {
                    tunnel: w770 -> [w782 w797]
                    tunnel: [w781 w796] -> w769
                    frame True {
                      # "Solenoid_R"
                      n537 = call "myRIO_BRig_RT_dataMTrig_Solenoid_N__R.vi"() -> ("output_Solenoid_N__R"=w771:i32)  [unwired: 11 in]
                      n538 = call "myRIO_BRig_RT_dataMTrig_Audio_N__L.vi"() -> ("output_Audio_N__L"=w778:i32)  [unwired: 11 in]
                      n539 = call "myRIO_BRig_RT_dataMTrig_Audio_N__R.vi"() -> ("output_Audio_N__R"=w773:i32)  [unwired: 11 in]
                      n540 = local read "sp_RightSpout"() -> (w777:u16)
                      n541 = Index Array(array=w782, index #1=w771, index #2=w778, index #3=w773) -> (element #1=w780:u16, element #2=w776:u16, element #3=w775:u16)
                      n542 = Increment(x=w780) -> (x+1=w779:u16)
                      n543 = case shown="2" w777 {
                        tunnel: w776 -> [w785 w788 w790]
                        tunnel: w775 -> [w783 w787 w792]
                        tunnel: [w784 w788 w789] -> w774
                        tunnel: [w783 w786 w791] -> w772
                        frame 0, Default {
                          n544 = Increment(x=w785) -> (x+1=w784:u16)
                        }
                        frame 1 {
                          n545 = Increment(x=w787) -> (x+1=w786:u16)
                        }
                        frame 2 {
                          n546 = Increment(x=w792) -> (x+1=w791:u16)
                          n547 = Increment(x=w790) -> (x+1=w789:u16)
                        }
                      }
                      n548 = Replace Array Subset(array=w782, new element #1=w779, index #1=w771, new element #2=w774, index #2=w778, new element #3=w772, index #3=w773) -> (w781:u16[])
                    }
                    frame False {
                      # "Solenoid_R"
                      n549 = call "myRIO_BRig_RT_dataMTrig_Solenoid_N__R.vi"() -> ("output_Solenoid_N__R"=w793:i32)  [unwired: 11 in]
                      n550 = Index Array(array=w797, index=w793) -> (element=w795:u16)
                      n551 = Increment(x=w795) -> (x+1=w794:u16)
                      n552 = Replace Array Subset(array=w797, new element=w794, index=w793) -> (w796:u16[])
                    }
                  }
                  n553 = local write "MTrig_Solenoid_trig__R"(FALSE) -> ()
                }
                frame 3 {
                  w802 = FALSE
                  n554 = case shown="True" w799 {
                    tunnel: w801 -> [w816 w824]
                    tunnel: [w815 w823] -> w800
                    frame True {
                      # "Audio_R"
                      # "Solenoid_R"
                      # "Audio_L"
                      # "Solenoid_L"
                      n555 = call "myRIO_BRig_RT_dataMTrig_Solenoid_N__L.vi"() -> ("output_Solenoid_N__L"=w810:i32)  [unwired: 11 in]
                      n556 = call "myRIO_BRig_RT_dataMTrig_Audio_N__L.vi"() -> ("output_Audio_N__L"=w808:i32)  [unwired: 11 in]
                      n557 = call "myRIO_BRig_RT_dataMTrig_Solenoid_N__R.vi"() -> ("output_Solenoid_N__R"=w806:i32)  [unwired: 11 in]
                      n558 = call "myRIO_BRig_RT_dataMTrig_Audio_N__R.vi"() -> ("output_Audio_N__R"=w805:i32)  [unwired: 11 in]
                      n559 = Index Array(array=w816, index #1=w810, index #2=w808, index #3=w806, index #4=w805) -> (element #1=w814:u16, element #2=w813:u16, element #3=w812:u16, element #4=w811:u16)
                      n560 = Increment(x=w811) -> (x+1=w803:u16)
                      n561 = Increment(x=w814) -> (x+1=w809:u16)
                      n562 = Increment(x=w813) -> (x+1=w807:u16)
                      n563 = Increment(x=w812) -> (x+1=w804:u16)
                      n564 = Replace Array Subset(array=w816, new element #1=w809, index #1=w810, new element #2=w807, index #2=w808, new element #3=w804, index #3=w806, new element #4=w803, index #4=w805) -> (w815:u16[])
                    }
                    frame False {
                      # "Solenoid_R"
                      # "Solenoid_L"
                      n565 = call "myRIO_BRig_RT_dataMTrig_Solenoid_N__L.vi"() -> ("output_Solenoid_N__L"=w820:i32)  [unwired: 11 in]
                      n566 = call "myRIO_BRig_RT_dataMTrig_Solenoid_N__R.vi"() -> ("output_Solenoid_N__R"=w817:i32)  [unwired: 11 in]
                      n567 = Index Array(array=w824, index #1=w820, index #2=w817) -> (element #1=w822:u16, element #2=w821:u16)
                      n568 = Increment(x=w822) -> (x+1=w819:u16)
                      n569 = Increment(x=w821) -> (x+1=w818:u16)
                      n570 = Replace Array Subset(array=w824, new element #1=w819, index #1=w820, new element #2=w818, index #2=w817) -> (w823:u16[])
                    }
                  }
                  n571 = local write "MTrig_Solenoid_trig__L"(w802) -> ()
                  n572 = local write "MTrig_Solenoid_trig__R"(w802) -> ()
                }
              }
              n573 = local read "get_countPerMS"() -> (w711:bool)
              n574 = Select(t=myRIO_BRig_RT__Case_NonExp_stateList."Get_FPGA_count_per_ms" ("Enum"), s=w711, f=myRIO_BRig_RT__Case_NonExp_stateList."Idle_6" ("Enum")) -> (s? t:f=w709:T1)
              n575 = Select(t=myRIO_BRig_RT__Case_NonExp_stateList."Cue_pre", s=w716, f=myRIO_BRig_RT__Case_NonExp_stateList."DispenseWater_pre" ("Enum")) -> (s? t:f=w714:T1)
              n576 = Select(t=w714, s=w718, f=w709) -> (s? t:f=w719:T1)
            }
            frame "Idle_5" {
              w847 = u8 0 ("f")
              # "There are a number of tasks we need to perform\nwhile idling. To preserve our timing loop, we\nbreak up the IDLE state into smaller states"
              n577 = local read "MTrig_Solenoid_trig__L"() -> (w838:bool)
              n578 = local read "MTrig_Solenoid_trig__R"() -> (w848:bool)
              n579 = local read "warmupType"() -> (w826:u8)
              n580 = local read "Cue1Param_CueType_Switch"() -> (w825:u16)
              n581 = local read "warmup"() -> (w840:bool)
              n582 = Not Equal To 0?(x=w826) -> (x != 0?=w831:bool)
              n583 = Not(x=w831) -> (.not. x?=w841:bool)
              n584 = Select(t=u8 1, s=w838, f=w847) -> (s? t:f=w846:u8)
              n585 = Select(t=u8 2, s=w848, f=w847) -> (s? t:f=w845:u8)
              n586 = And(x=w840, y=w841) -> (x .and. y?=w839:bool)
              n587 = And(x=w840, y=w831) -> (x .and. y?=w834:bool)
              n588 = Add(x=w846, y=w845) -> (x+y=w844:u8)
              n589 = case shown="2" w844 {
                tunnel: w843 -> [w851 w856 w905 w955]
                tunnel: [w851 w855 w904 w954] -> w842
                tunnel: w839 -> [_ w854 w903 w953]
                tunnel: [_ TRUE TRUE TRUE] -> w836
                tunnel: w825 -> [_ w852 w901 w951]
                frame 0, Default {
                }
                frame 1 {
                  n590 = case shown="True" w854 {
                    tunnel: w856 -> [w861 w900]
                    tunnel: [w860 w899] -> w855
                    tunnel: w852 -> [w859 _]
                    frame True {
                      n591 = case shown="0, Default" w859 {
                        tunnel: [TRUE _ w893] -> w858
                        frame 0, Default {
                          # "Audio"
                        }
                        frame 1 {
                          # "LED"
                        }
                        frame 2 {
                          # "Audio or LED"
                          n592 = local read "Cue1Param_AudioLed_Probability_Switch"() -> (w895:u16)
                          n593 = call "myRIO__convert__Probability_to_TrueFalse.vi"("input_probability_u16"=w895) -> ("output_TF"=w894:bool)  [unwired: 10 in]
                          n594 = Not(x=w894) -> (.not. x?=w893:bool)
                        }
                      }
                      n595 = case shown="True" w858 {
                        tunnel: w861 -> [w873 w891]
                        tunnel: [w872 w890] -> w860
                        frame True {
                          n596 = call "myRIO_BRig_RT_dataMTrig_Solenoid_N__L.vi"() -> ("output_Solenoid_N__L"=w870:i32)  [unwired: 11 in]
                          n597 = call "myRIO_BRig_RT_dataMTrig_Audio_N__L.vi"() -> ("output_Audio_N__L"=w868:i32)  [unwired: 11 in]
                          n598 = call "myRIO_BRig_RT_dataMTrig_Audio_N__R.vi"() -> ("output_Audio_N__R"=w863:i32)  [unwired: 11 in]
                          n599 = local read "sp_LeftSpout"() -> (w867:u16)
                          n600 = Index Array(array=w873, index #1=w870, index #2=w868, index #3=w863) -> (element #1=w871:u16, element #2=w866:u16, element #3=w865:u16)
                          n601 = case shown="2" w867 {
                            tunnel: w866 -> [w876 w879 w881]
                            tunnel: w865 -> [w874 w878 w883]
                            tunnel: [w875 w879 w880] -> w864
                            tunnel: [w874 w877 w882] -> w862
                            frame 0, Default {
                              n602 = Increment(x=w876) -> (x+1=w875:u16)
                            }
                            frame 1 {
                              n603 = Increment(x=w878) -> (x+1=w877:u16)
                            }
                            frame 2 {
                              n604 = Increment(x=w883) -> (x+1=w882:u16)
                              n605 = Increment(x=w881) -> (x+1=w880:u16)
                            }
                          }
                          n606 = Increment(x=w871) -> (x+1=w869:u16)
                          n607 = Replace Array Subset(array=w873, new element #1=w869, index #1=w870, new element #2=w864, index #2=w868, new element #3=w862, index #3=w863) -> (w872:u16[])
                        }
                        frame False {
                          n608 = call "myRIO_BRig_RT_dataMTrig_Solenoid_N__L.vi"() -> ("output_Solenoid_N__L"=w888:i32)  [unwired: 11 in]
                          n609 = call "myRIO_BRig_RT_dataMTrig_CueLed_N.vi"() -> ("output_CueLed_N"=w886:i32)  [unwired: 11 in]
                          n610 = Index Array(array=w891, index #1=w888, index #2=w886) -> (element #1=w889:u16, element #2=w885:u16)
                          n611 = Increment(x=w889) -> (x+1=w887:u16)
                          n612 = Increment(x=w885) -> (x+1=w884:u16)
                          n613 = Replace Array Subset(array=w891, new element #1=w887, index #1=w888, new element #2=w884, index #2=w886) -> (w890:u16[])
                        }
                      }
                    }
                    frame False {
                      # "Solenoid_L"
                      n614 = call "myRIO_BRig_RT_dataMTrig_Solenoid_N__L.vi"() -> ("output_Solenoid_N__L"=w897:i32)  [unwired: 11 in]
                      n615 = Index Array(array=w900, index=w897) -> (element=w898:u16)
                      n616 = Increment(x=w898) -> (x+1=w896:u16)
                      n617 = Replace Array Subset(array=w900, new element=w896, index=w897) -> (w899:u16[])
                    }
                  }
                  n618 = local write "MTrig_Solenoid_trig__L"(FALSE) -> ()
                }
                frame 2 {
                  n619 = case shown="True" w903 {
                    tunnel: w905 -> [w910 w949]
                    tunnel: [w909 w948] -> w904
                    tunnel: w901 -> [w908 _]
                    frame True {
                      n620 = case shown="0, Default" w908 {
                        tunnel: [TRUE _ w942] -> w907
                        frame 0, Default {
                          # "Audio"
                        }
                        frame 1 {
                          # "LED"
                        }
                        frame 2 {
                          # "Audio or LED"
                          n621 = local read "Cue1Param_AudioLed_Probability_Switch"() -> (w944:u16)
                          n622 = call "myRIO__convert__Probability_to_TrueFalse.vi"("input_probability_u16"=w944) -> ("output_TF"=w943:bool)  [unwired: 10 in]
                          n623 = Not(x=w943) -> (.not. x?=w942:bool)
                        }
                      }
                      n624 = case shown="True" w907 {
                        tunnel: w910 -> [w922 w940]
                        tunnel: [w921 w939] -> w909
                        frame True {
                          n625 = call "myRIO_BRig_RT_dataMTrig_Solenoid_N__R.vi"() -> ("output_Solenoid_N__R"=w919:i32)  [unwired: 11 in]
                          n626 = call "myRIO_BRig_RT_dataMTrig_Audio_N__L.vi"() -> ("output_Audio_N__L"=w917:i32)  [unwired: 11 in]
                          n627 = call "myRIO_BRig_RT_dataMTrig_Audio_N__R.vi"() -> ("output_Audio_N__R"=w912:i32)  [unwired: 11 in]
                          n628 = local read "sp_RightSpout"() -> (w916:u16)
                          n629 = Index Array(array=w922, index #1=w919, index #2=w917, index #3=w912) -> (element #1=w920:u16, element #2=w915:u16, element #3=w914:u16)
                          n630 = case shown="2" w916 {
                            tunnel: w915 -> [w925 w928 w930]
                            tunnel: w914 -> [w923 w927 w932]
                            tunnel: [w924 w928 w929] -> w913
                            tunnel: [w923 w926 w931] -> w911
                            frame 0, Default {
                              n631 = Increment(x=w925) -> (x+1=w924:u16)
                            }
                            frame 1 {
                              n632 = Increment(x=w927) -> (x+1=w926:u16)
                            }
                            frame 2 {
                              n633 = Increment(x=w932) -> (x+1=w931:u16)
                              n634 = Increment(x=w930) -> (x+1=w929:u16)
                            }
                          }
                          n635 = Increment(x=w920) -> (x+1=w918:u16)
                          n636 = Replace Array Subset(array=w922, new element #1=w918, index #1=w919, new element #2=w913, index #2=w917, new element #3=w911, index #3=w912) -> (w921:u16[])
                        }
                        frame False {
                          n637 = call "myRIO_BRig_RT_dataMTrig_Solenoid_N__R.vi"() -> ("output_Solenoid_N__R"=w937:i32)  [unwired: 11 in]
                          n638 = call "myRIO_BRig_RT_dataMTrig_CueLed_N.vi"() -> ("output_CueLed_N"=w935:i32)  [unwired: 11 in]
                          n639 = Index Array(array=w940, index #1=w937, index #2=w935) -> (element #1=w938:u16, element #2=w934:u16)
                          n640 = Increment(x=w938) -> (x+1=w936:u16)
                          n641 = Increment(x=w934) -> (x+1=w933:u16)
                          n642 = Replace Array Subset(array=w940, new element #1=w936, index #1=w937, new element #2=w933, index #2=w935) -> (w939:u16[])
                        }
                      }
                    }
                    frame False {
                      # "Solenoid_R"
                      n643 = call "myRIO_BRig_RT_dataMTrig_Solenoid_N__R.vi"() -> ("output_Solenoid_N__R"=w946:i32)  [unwired: 11 in]
                      n644 = Index Array(array=w949, index=w946) -> (element=w947:u16)
                      n645 = Increment(x=w947) -> (x+1=w945:u16)
                      n646 = Replace Array Subset(array=w949, new element=w945, index=w946) -> (w948:u16[])
                    }
                  }
                  n647 = local write "MTrig_Solenoid_trig__R"(FALSE) -> ()
                }
                frame 3 {
                  w950 = FALSE
                  n648 = case shown="True" w953 {
                    tunnel: w955 -> [w959 w996]
                    tunnel: [w958 w995] -> w954
                    tunnel: w951 -> [w957 _]
                    frame True {
                      n649 = case shown="2" w957 {
                        tunnel: [TRUE _ w986] -> w956
                        frame 0, Default {
                          # "Audio"
                        }
                        frame 1 {
                          # "LED"
                        }
                        frame 2 {
                          # "Audio or LED"
                          n650 = local read "Cue1Param_AudioLed_Probability_Switch"() -> (w988:u16)
                          n651 = call "myRIO__convert__Probability_to_TrueFalse.vi"("input_probability_u16"=w988) -> ("output_TF"=w987:bool)  [unwired: 10 in]
                          n652 = Not(x=w987) -> (.not. x?=w986:bool)
                        }
                      }
                      n653 = case shown="True" w956 {
                        tunnel: w959 -> [w973 w984]
                        tunnel: [w972 w983] -> w958
                        frame True {
                          n654 = call "myRIO_BRig_RT_dataMTrig_Solenoid_N__L.vi"() -> ("output_Solenoid_N__L"=w961:i32)  [unwired: 11 in]
                          n655 = call "myRIO_BRig_RT_dataMTrig_Solenoid_N__R.vi"() -> ("output_Solenoid_N__R"=w970:i32)  [unwired: 11 in]
                          n656 = call "myRIO_BRig_RT_dataMTrig_Audio_N__L.vi"() -> ("output_Audio_N__L"=w968:i32)  [unwired: 11 in]
                          n657 = call "myRIO_BRig_RT_dataMTrig_Audio_N__R.vi"() -> ("output_Audio_N__R"=w964:i32)  [unwired: 11 in]
                          n658 = Index Array(array=w973, index #1=w961, index #2=w970, index #3=w968, index #4=w964) -> (element #1=w962:u16, element #2=w971:u16, element #3=w967:u16, element #4=w966:u16)
                          n659 = Increment(x=w962) -> (x+1=w960:u16)
                          n660 = Increment(x=w971) -> (x+1=w969:u16)
                          n661 = Increment(x=w966) -> (x+1=w963:u16)
                          n662 = Increment(x=w967) -> (x+1=w965:u16)
                          n663 = Replace Array Subset(array=w973, new element #1=w960, index #1=w961, new element #2=w969, index #2=w970, new element #3=w965, index #3=w968, new element #4=w963, index #4=w964) -> (w972:u16[])
                        }
                        frame False {
                          n664 = call "myRIO_BRig_RT_dataMTrig_Solenoid_N__L.vi"() -> ("output_Solenoid_N__L"=w974:i32)  [unwired: 11 in]
                          n665 = call "myRIO_BRig_RT_dataMTrig_Solenoid_N__R.vi"() -> ("output_Solenoid_N__R"=w981:i32)  [unwired: 11 in]
                          n666 = call "myRIO_BRig_RT_dataMTrig_CueLed_N.vi"() -> ("output_CueLed_N"=w979:i32)  [unwired: 11 in]
                          n667 = Index Array(array=w984, index #1=w974, index #2=w981, index #3=w979) -> (element #1=w976:u16, element #2=w982:u16, element #3=w978:u16)
                          n668 = Increment(x=w976) -> (x+1=w975:u16)
                          n669 = Increment(x=w982) -> (x+1=w980:u16)
                          n670 = Increment(x=w978) -> (x+1=w977:u16)
                          n671 = Replace Array Subset(array=w984, new element #1=w975, index #1=w974, new element #2=w980, index #2=w981, new element #3=w977, index #3=w979) -> (w983:u16[])
                        }
                      }
                    }
                    frame False {
                      n672 = call "myRIO_BRig_RT_dataMTrig_Solenoid_N__L.vi"() -> ("output_Solenoid_N__L"=w992:i32)  [unwired: 11 in]
                      n673 = call "myRIO_BRig_RT_dataMTrig_Solenoid_N__R.vi"() -> ("output_Solenoid_N__R"=w991:i32)  [unwired: 11 in]
                      n674 = Index Array(array=w996, index #1=w992, index #2=w991) -> (element #1=w994:u16, element #2=w990:u16)
                      n675 = Increment(x=w990) -> (x+1=w989:u16)
                      n676 = Increment(x=w994) -> (x+1=w993:u16)
                      n677 = Replace Array Subset(array=w996, new element #1=w993, index #1=w992, new element #2=w989, index #2=w991) -> (w995:u16[])
                    }
                  }
                  n678 = local write "MTrig_Solenoid_trig__L"(w950) -> ()
                  n679 = local write "MTrig_Solenoid_trig__R"(w950) -> ()
                }
              }
              n680 = local read "get_countPerMS"() -> (w830:bool)
              n681 = Select(t=myRIO_BRig_RT__Case_NonExp_stateList."Get_FPGA_count_per_ms" ("Enum"), s=w830, f=myRIO_BRig_RT__Case_NonExp_stateList."Idle_6" ("Enum")) -> (s? t:f=w828:T1)
              n682 = Select(t=myRIO_BRig_RT__Case_NonExp_stateList."Cue_pre", s=w834, f=myRIO_BRig_RT__Case_NonExp_stateList."DispenseWater_pre" ("Enum")) -> (s? t:f=w832:T1)
              n683 = Select(t=w832, s=w836, f=w828) -> (s? t:f=w837:T1)
            }
            frame "Idle_6" {
              # "There are a number of tasks we need to perform\nwhile idling. To preserve our timing loop, we\nbreak up the IDLE state into smaller states"
              # "use dataMTrig as it is one of the last to transfer"
              n684 = call "myRIO_BRig_RT_comm_webdav_uploadReceived_check_v2,0.vi"("input_dataName"="dataMTrig") -> ("output_Iexist"=w1001:bool)  [unwired: 9 in, 1 out]
              n685 = Select(t=myRIO_BRig_RT__Case_NonExp_stateList."UploadSettings_pre" ("Enum"), s=w1001, f=myRIO_BRig_RT__Case_NonExp_stateList."Idle") -> (s? t:f=w999:T1)
            }
            frame "Cue_pre" {
              w1008 = u16 0 ("new element/subarray")
              # "Audio cue or LED cue?"
              # "Audio, LED, or \"Audio or LED\""
              # "Right Audio?"
              # "Left Audio?"
              # "Left or Right?"
              # "Cue Audio?\n(T=Audio, F=LED)"
              # "Ncycle"
              # "count"
              # "Audio_R"
              # "Ncycle"
              # "count"
              # "Audio_L"
              n686 = local read "Cue1Param_CueType_Switch"() -> (w1032:u16)
              n687 = case shown="2" w1032 {
                tunnel: [TRUE _ w1050] -> w1004
                frame 0, Default {
                  # "Audio"
                }
                frame 1 {
                  # "LED"
                }
                frame 2 {
                  # "Audio or LED"
                  n688 = local read "Cue1Param_AudioLed_Probability_Switch"() -> (w1052:u16)
                  n689 = call "myRIO__convert__Probability_to_TrueFalse.vi"("input_probability_u16"=w1052) -> ("output_TF"=w1051:bool)  [unwired: 10 in]
                  n690 = Not(x=w1051) -> (.not. x?=w1050:bool)
                }
              }
              n691 = call "myRIO_BRig_RT_dataMTrig_Solenoid_N__L.vi"() -> ("output_Solenoid_N__L"=w1042:i32)  [unwired: 11 in]
              n692 = call "myRIO_BRig_RT_dataMTrig_Solenoid_N__R.vi"() -> ("output_Solenoid_N__R"=w1041:i32)  [unwired: 11 in]
              n693 = Index Array(array=w1038, index #1=w1042, index #2=w1041) -> (element #1=w1040:u16, element #2=w1039:u16)
              n694 = Not Equal To 0?(x=w1040) -> (x != 0?=w1028:bool)
              n695 = Not Equal To 0?(x=w1039) -> (x != 0?=w1027:bool)
              n696 = Not(x=w1004) -> (.not. x?=w1003:bool)
              n697 = And(x=w1004, y=w1028) -> (x .and. y?=w1022:bool)
              n698 = And(x=w1004, y=w1027) -> (x .and. y?=w1020:bool)
              n699 = Select(t=myRIO_BRig_RT__Case_NonExp_stateList."Cue", s=w1004, f=myRIO_BRig_RT__Case_NonExp_stateList."Cue") -> (s? t:f=w1030:T1)
              n700 = local read "sp_RightSpout"() -> (w1021:u16)
              n701 = local read "sp_LeftSpout"() -> (w1023:u16)
              n702 = Boolean To (0,1)(Boolean=w1003) -> (0, 1=w1006:i16)
              n703 = To Unsigned Word Integer(number=w1006) -> (unsigned 16bit integer=w1005:u16)
              n704 = case shown="0, Default" w1023 {
                tunnel: [w1046 _ w1048] -> w1019
                tunnel: [_ w1047 w1048] -> w1017
                tunnel: w1022 -> [w1046 w1047 w1048]
                frame 0, Default {
                }
                frame 1 {
                }
                frame 2 {
                }
              }
              n705 = case shown="0, Default" w1021 {
                tunnel: [w1043 _ w1045] -> w1018
                tunnel: [_ w1044 w1045] -> w1016
                tunnel: w1020 -> [w1043 w1044 w1045]
                frame 0, Default {
                }
                frame 1 {
                }
                frame 2 {
                }
              }
              n706 = call "myRIO_BRig_RT_dataMTrig_Audio_c__L.vi"() -> ("output_Audio_c__L"=w1036:i32)  [unwired: 11 in]
              n707 = call "myRIO_BRig_RT_dataMTrig_Audio_N__L.vi"() -> ("output_Audio_N__L"=w1035:i32)  [unwired: 11 in]
              n708 = call "myRIO_BRig_RT_dataMTrig_Audio_c__R.vi"() -> ("output_Audio_c__R"=w1034:i32)  [unwired: 11 in]
              n709 = call "myRIO_BRig_RT_dataMTrig_Audio_N__R.vi"() -> ("output_Audio_N__R"=w1033:i32)  [unwired: 11 in]
              n710 = call "myRIO_BRig_RT_dataMTrig_CueLed_c.vi"() -> ("output_CueLed_c"=w1009:i32)  [unwired: 11 in]
              n711 = call "myRIO_BRig_RT_dataMTrig_CueLed_N.vi"() -> ("output_CueLed_N"=w1007:i32)  [unwired: 11 in]
              n712 = Or(x=w1019, y=w1018) -> (x .or. y?=w1015:bool)
              n713 = Boolean To (0,1)(Boolean=w1015) -> (0, 1=w1013:i16)
              n714 = To Unsigned Word Integer(number=w1013) -> (unsigned 16bit integer=w1012:u16)
              n715 = Or(x=w1017, y=w1016) -> (x .or. y?=w1014:bool)
              n716 = Boolean To (0,1)(Boolean=w1014) -> (0, 1=w1011:i16)
              n717 = To Unsigned Word Integer(number=w1011) -> (unsigned 16bit integer=w1010:u16)
              n718 = Replace Array Subset(array=w1038, new element #1=w1008, index #1=w1036, new element #2=w1012, index #2=w1035, new element #3=w1008, index #3=w1034, new element #4=w1010, index #4=w1033, new element #5=w1008, index #5=w1009, new element #6=w1005, index #6=w1007) -> (w1037:u16[])
              n719 = Initialize Array(u16 0 ("element"), 1 ("dimension size")) -> (w1026:u16[])
            }
            frame "Cue" {
              # "warmupType\n0 = Cue with reward (not possible to be in this state with value==0)\n1 = Cue then reward\n2 = Cue then reward (no lick)"
              # "Audio cue"
              # "lick did not occur or warmupType==1"
              # "lick occurred?"
              # "Ncycle"
              # "Audio_R"
              # "Ncycle"
              # "Audio_L"
              n720 = local read "warmupType"() -> (w1062:u8)
              n721 = Greater?(x=w1068, y=w1067) -> (0:w1071:bool)
              n722 = Greater?(x=w1070, y=w1069) -> (0:w1066:bool)
              n723 = Or(x=w1066, y=w1071) -> (x .or. y?=w1060:bool)
              n724 = Equal?(x=w1062, y=u8 1) -> (x = y?=w1056:bool)
              n725 = Not(x=w1060) -> (.not. x?=w1059:bool)
              n726 = call "myRIO_BRig_RT_dataMTrig_Audio_N__L.vi"() -> ("output_Audio_N__L"=w1073:i32)  [unwired: 11 in]
              n727 = call "myRIO_BRig_RT_dataMTrig_Audio_N__R.vi"() -> ("output_Audio_N__R"=w1072:i32)  [unwired: 11 in]
              n728 = call "myRIO_BRig_RT_dataMTrig_CueLed_N.vi"() -> ("output_CueLed_N"=w1053:i32)  [unwired: 11 in]
              n729 = Or(x=w1059, y=w1056) -> (x .or. y?=w1057:bool)
              n730 = case shown="True" w1057 {
                tunnel: w1073 -> [w1079 w1100]
                tunnel: w1072 -> [w1078 w1099]
                tunnel: w1065 -> [w1081 w1094]
                tunnel: [w1080 w1094] -> w1064
                tunnel: w1063 -> [_ w1092]
                tunnel: [myRIO_BRig_RT__Case_NonExp_stateList."Idle" ("t") w1091] -> w1058
                tunnel: w1056 -> [_ w1090]
                tunnel: w1055 -> [_ w1086]
                tunnel: w1054 -> [_ w1085]
                tunnel: w1053 -> [_ w1084]
                frame False {
                  w1074 = u16 0 ("new element/subarray")
                  # "lick occurred and warmupType==2"
                  n731 = call "myRIO_BRig_RT_dataMTrig_Solenoid_N__R.vi"() -> ("output_Solenoid_N__R"=w1075:i32)  [unwired: 11 in]
                  n732 = call "myRIO_BRig_RT_dataMTrig_Solenoid_N__L.vi"() -> ("output_Solenoid_N__L"=w1076:i32)  [unwired: 11 in]
                  n733 = Replace Array Subset(array=w1081, new element #1=w1074, index #1=w1079, new element #2=w1074, index #2=w1078, new element #3=w1074, index #3=w1076, new element #4=w1074, index #4=w1075) -> (w1080:u16[])
                }
                frame True {
                  n734 = Not(x=w1090) -> (.not. x?=w1089:bool)
                  n735 = Index Array(array=w1094, index #1=w1100, index #2=w1099, index #3=w1084) -> (element #1=w1098:u16, element #2=w1097:u16, element #3=w1083:u16)
                  n736 = Equal To 0?(x=w1098) -> (x = 0?=w1096:bool)
                  n737 = Equal To 0?(x=w1097) -> (x = 0?=w1095:bool)
                  n738 = Equal To 0?(x=w1083) -> (x = 0?=w1082:bool)
                  n739 = Compound Arithmetic op=AND(w1096, w1095, w1082) -> (w1088:bool)
                  n740 = And(x=w1088, y=w1089) -> (x .and. y?=w1087:bool)
                  n741 = case shown="True" w1087 {
                    tunnel: w1086 -> [_ w1108]
                    tunnel: w1085 -> [_ w1103]
                    frame False {
                    }
                    frame True {
                      n742 = local read "count_warmup_R"() -> (w1101:u16)
                      n743 = local read "count_warmup_L"() -> (w1106:u16)
                      n744 = Increment(x=w1101) -> (x+1=w1104:u16)
                      n745 = Increment(x=w1106) -> (x+1=w1107:u16)
                      n746 = Select(t=w1104, s=w1103, f=w1101) -> (s? t:f=w1102:u16)
                      n747 = Select(t=w1107, s=w1108, f=w1106) -> (s? t:f=w1105:u16)
                      n748 = local write "count_warmup_R"(w1102) -> ()
                      n749 = local write "count_warmup_L"(w1105) -> ()
                    }
                  }
                  n750 = Select(t=myRIO_BRig_RT__Case_NonExp_stateList."DispenseWater_pre", s=w1088, f=w1092) -> (s? t:f=w1091:T1)
                }
              }
            }
            frame "Cue_LED" {
              # "LED Cue"
              # "lick did not occur or warmupType==1"
              # "lick occurred?"
              n751 = local read "warmupType"() -> (w1121:u8)
              n752 = Greater?(x=w1127, y=w1126) -> (0:w1130:bool)
              n753 = Greater?(x=w1129, y=w1128) -> (0:w1125:bool)
              n754 = Or(x=w1125, y=w1130) -> (x .or. y?=w1119:bool)
              n755 = Equal?(x=w1121, y=u8 1) -> (x = y?=w1115:bool)
              n756 = Not(x=w1119) -> (.not. x?=w1118:bool)
              n757 = Or(x=w1118, y=w1115) -> (x .or. y?=w1116:bool)
              n758 = case shown="True" w1116 {
                tunnel: w1124 -> [w1137 w1157]
                tunnel: [w1136 w1157] -> w1123
                tunnel: w1122 -> [_ w1143]
                tunnel: [myRIO_BRig_RT__Case_NonExp_stateList."Idle" ("t") w1156] -> w1117
                tunnel: w1115 -> [_ w1142]
                tunnel: w1114 -> [_ w1154]
                tunnel: w1113 -> [_ w1153]
                tunnel: w1112 -> [w1131 w1152]
                tunnel: [w1131 w1145] -> w1111
                tunnel: w1110 -> [_ w1140]
                tunnel: w1109 -> [_ w1139]
                frame False {
                  w1132 = u16 0 ("new element/subarray")
                  # "lick occurred and warmupType==2"
                  n759 = call "myRIO_BRig_RT_dataMTrig_Solenoid_N__R.vi"() -> ("output_Solenoid_N__R"=w1133:i32)  [unwired: 11 in]
                  n760 = call "myRIO_BRig_RT_dataMTrig_Solenoid_N__L.vi"() -> ("output_Solenoid_N__L"=w1134:i32)  [unwired: 11 in]
                  n761 = Replace Array Subset(array=w1137, new element #1=w1132, new element #2=w1132, index #2=w1134, new element #3=w1132, index #3=w1133) -> (w1136:u16[])  [unwired: 1 in]
                }
                frame True {
                  w1150 = 0 ("index")
                  n762 = local read "Tcycle_Cue_LED_min"() -> (w1146:u16)
                  n763 = Index Array(array=w1152, index=w1150) -> (element=w1151:u16)
                  n764 = Increment(x=w1151) -> (x+1=w1149:u16)
                  n765 = Multiply(x=w1149, y=u16 5) -> (x*y=w1147:u16)
                  n766 = Replace Array Subset(array=w1152, new element=w1149, index=w1150) -> (w1145:u16[])
                  n767 = Less?(x=w1147, y=w1146) -> (x < y?=w1141:bool)
                  n768 = Not Or(1:w1142, 2:w1141) -> (0:w1155:bool)
                  n769 = case shown="True" w1155 {
                    tunnel: w1154 -> [_ w1165]
                    tunnel: w1153 -> [_ w1160]
                    frame False {
                    }
                    frame True {
                      n770 = local read "count_warmup_R"() -> (w1158:u16)
                      n771 = local read "count_warmup_L"() -> (w1163:u16)
                      n772 = Increment(x=w1158) -> (x+1=w1161:u16)
                      n773 = Increment(x=w1163) -> (x+1=w1164:u16)
                      n774 = Select(t=w1161, s=w1160, f=w1158) -> (s? t:f=w1159:u16)
                      n775 = Select(t=w1164, s=w1165, f=w1163) -> (s? t:f=w1162:u16)
                      n776 = local write "count_warmup_R"(w1159) -> ()
                      n777 = local write "count_warmup_L"(w1162) -> ()
                    }
                  }
                  n778 = Select(t=w1143, s=w1141, f=myRIO_BRig_RT__Case_NonExp_stateList."DispenseWater_pre" ("t")) -> (s? t:f=w1156:T1)
                  n779 = xnode "Read/Write Control"("FPGA VI Reference In"=w1140, "error in"=w1139, "CueLed_Event"=w1141) -> ("error out"=w1138:errorcluster)  [unwired: 1 out]
                  n780 = local write "error out"(w1138) -> ()
                }
              }
            }
            frame "RewardCalibration_pre" {
              (unwired) FALSE
              w1166 = FALSE
              w1177 = u8 0
              w1193 = u8 0
              # "Are we starting a RewardCalibration?\nOr are we stopping a RewardCalibration?\nOr is a RewardCalibration over?"
              # "RewCalib\nOnOff"
              # "N"
              # "Solenoid R"
              # "RewCalib\nOnOff"
              # "N"
              # "Solenoid L"
              n781 = local read "RewCalib_Trig_L"() -> (w1200:bool)
              n782 = local read "RewCalib_Trig_R"() -> (w1169:bool)
              n783 = call "myRIO_BRig_RT_dataMTrig_Solenoid_N__R.vi"() -> ("output_Solenoid_N__R"=w1171:i32)  [unwired: 11 in]
              n784 = call "myRIO_BRig_RT_dataMTrig_Solenoid_RewCalib_OnOff__R.vi"() -> ("output_Solenoid_RewCalib_OnOff__R"=w1168:i32)  [unwired: 11 in]
              n785 = call "myRIO_BRig_RT_dataMTrig_Solenoid_N__L.vi"() -> ("output_Solenoid_N__L"=w1186:i32)  [unwired: 11 in]
              n786 = call "myRIO_BRig_RT_dataMTrig_Solenoid_RewCalib_OnOff__L.vi"() -> ("output_Solenoid_RewCalib_OnOff__L"=w1187:i32)  [unwired: 11 in]
              n787 = Index Array(array=w1170, index #1=w1171, index #2=w1168) -> (element #1=w1181:u16, element #2=w1176:u16)
              n788 = Index Array(array=w1170, index #1=w1186, index #2=w1187) -> (element #1=w1197:u16, element #2=w1192:u16)
              n789 = Equal To 0?(x=w1181) -> (x = 0?=w1182:bool)
              n790 = Not Equal To 0?(x=w1176) -> (x != 0?=w1179:bool)
              n791 = Equal To 0?(x=w1197) -> (x = 0?=w1198:bool)
              n792 = Not Equal To 0?(x=w1192) -> (x != 0?=w1195:bool)
              n793 = local write "MTrig_Solenoid_trig__L"(w1166) -> ()
              n794 = local write "MTrig_Solenoid_trig__R"(w1166) -> ()
              n795 = Select(t=u8 1, s=w1169, f=w1177) -> (s? t:f=w1173:u8)
              n796 = Select(t=u8 1, s=w1200, f=w1193) -> (s? t:f=w1189:u8)
              n797 = Select(t=u8 2, s=w1182, f=w1177) -> (s? t:f=w1174:u8)
              n798 = Select(t=u8 4, s=w1179, f=w1177) -> (s? t:f=w1175:u8)
              n799 = Select(t=u8 2, s=w1198, f=w1193) -> (s? t:f=w1190:u8)
              n800 = Select(t=u8 4, s=w1195, f=w1193) -> (s? t:f=w1191:u8)
              n801 = Compound Arithmetic op=ADD(w1173, w1174, w1175) -> (w1172:u8)
              n802 = Compound Arithmetic op=ADD(w1189, w1190, w1191) -> (w1188:u8)
              n803 = case shown="7" w1188 {
                tunnel: w1170 -> [w1230 w1235 w1237 w1242 w1247 w1249 w1252 w1257]
                tunnel: [w1230 w1236 w1237 w1243 w1248 w1249 w1253 w1258] -> w1185
                tunnel: w1187 -> [_ w1233 _ w1240 w1245 _ w1251 w1256]
                tunnel: w1186 -> [_ w1234 _ w1241 w1246 _ _ _]
                frame 0, Default {
                }
                frame 1 {
                  n804 = Replace Array Subset(array=w1235, new element #1=u16 100 ("new element/subarray"), index #1=w1234, new element #2=u16 1 ("new element/subarray"), index #2=w1233) -> (w1236:u16[])
                }
                frame 2 {
                }
                frame 3 {
                  n805 = Replace Array Subset(array=w1242, new element #1=u16 100 ("new element/subarray"), index #1=w1241, new element #2=u16 1 ("new element/subarray"), index #2=w1240) -> (w1243:u16[])
                }
                frame 4 {
                  w1244 = u16 0 ("new element/subarray")
                  n806 = Replace Array Subset(array=w1247, new element #1=w1244, index #1=w1246, new element #2=w1244, index #2=w1245) -> (w1248:u16[])
                }
                frame 5 {
                }
                frame 6 {
                  n807 = Replace Array Subset(array=w1252, new element=u16 0 ("new element/subarray"), index=w1251) -> (w1253:u16[])
                }
                frame 7 {
                  n808 = local write "RewCalib_Trig_L"(FALSE ("RewCalib_Trig_L")) -> ()
                  n809 = Replace Array Subset(array=w1257, new element=u16 0 ("new element/subarray"), index=w1256) -> (w1258:u16[])
                }
              }
              n810 = case shown="7" w1172 {
                tunnel: w1185 -> [w1201 w1206 w1208 w1213 w1218 w1220 w1223 w1228]
                tunnel: [w1201 w1207 w1208 w1214 w1219 w1220 w1224 w1229] -> w1184
                tunnel: w1168 -> [_ w1204 _ w1211 w1216 _ w1222 w1227]
                tunnel: w1171 -> [_ w1205 _ w1212 w1217 _ _ _]
                frame 0, Default {
                }
                frame 1 {
                  n811 = Replace Array Subset(array=w1206, new element #1=u16 100 ("new element/subarray"), index #1=w1205, new element #2=u16 1 ("new element/subarray"), index #2=w1204) -> (w1207:u16[])
                }
                frame 2 {
                }
                frame 3 {
                  n812 = Replace Array Subset(array=w1213, new element #1=u16 100 ("new element/subarray"), index #1=w1212, new element #2=u16 1 ("new element/subarray"), index #2=w1211) -> (w1214:u16[])
                }
                frame 4 {
                  w1215 = u16 0 ("new element/subarray")
                  n813 = Replace Array Subset(array=w1218, new element #1=w1215, index #1=w1217, new element #2=w1215, index #2=w1216) -> (w1219:u16[])
                }
                frame 5 {
                }
                frame 6 {
                  n814 = Replace Array Subset(array=w1223, new element=u16 0 ("new element/subarray"), index=w1222) -> (w1224:u16[])
                }
                frame 7 {
                  n815 = local write "RewCalib_Trig_R"(FALSE ("RewCalib_Trig_L")) -> ()
                  n816 = Replace Array Subset(array=w1228, new element=u16 0 ("new element/subarray"), index=w1227) -> (w1229:u16[])
                }
              }
            }
            frame "DispenseWater_pre" {
              w1264 = u16 0 ("t")
              w1307 = u16 0 ("new element/subarray")
              # "just trust me on this one"
              # "RewCalib\nOnOff"
              # "RewCalib\nOnOff"
              # "nCycle"
              # "Solenoid__R"
              # "Tdelay"
              # "delay"
              # "nCycle"
              # "Solenoid__L"
              # "Tdelay"
              # "delay"
              # "Solenoid__R"
              # "count"
              # "Solenoid_Tcycle_R"
              # "Solenoid_Tcycle_L"
              # "Solenoid__L"
              # "count"
              n817 = call "myRIO_BRig_RT_dataMTrig_Solenoid_RewCalib_OnOff__L.vi"() -> ("output_Solenoid_RewCalib_OnOff__L"=w1271:i32)  [unwired: 11 in]
              n818 = call "myRIO_BRig_RT_dataMTrig_Solenoid_N__L.vi"() -> ("output_Solenoid_N__L"=w1262:i32)  [unwired: 11 in]
              n819 = call "myRIO_BRig_RT_dataMTrig_Solenoid_delay__L.vi"() -> ("output_Solenoid_delay__L"=w1305:i32)  [unwired: 11 in]
              n820 = call "myRIO_BRig_RT_dataMTrig_Solenoid_Tdelay__L.vi"() -> ("output_Solenoid_Tdelay__L"=w1304:i32)  [unwired: 11 in]
              n821 = call "myRIO_BRig_RT_dataMTrig_Solenoid_N__R.vi"() -> ("output_Solenoid_N__R"=w1260:i32)  [unwired: 11 in]
              n822 = call "myRIO_BRig_RT_dataMTrig_Solenoid_delay__R.vi"() -> ("output_Solenoid_delay__R"=w1294:i32)  [unwired: 11 in]
              n823 = call "myRIO_BRig_RT_dataMTrig_Solenoid_Tdelay__R.vi"() -> ("output_Solenoid_Tdelay__R"=w1293:i32)  [unwired: 11 in]
              n824 = call "myRIO_BRig_RT_dataMTrig_Solenoid_RewCalib_OnOff__R.vi"() -> ("output_Solenoid_RewCalib_OnOff__R"=w1267:i32)  [unwired: 11 in]
              n825 = Index Array(array=w1306, index #1=w1262, index #2=w1305, index #3=w1304, index #4=w1260, index #5=w1294, index #6=w1293, index #7=w1271, index #8=w1267) -> (element #1=w1263:u16, element #2=w1303:u16, element #3=w1298:u16, element #4=w1266:u16, element #5=w1288:u16, element #6=w1287:u16, element #7=w1272:u16, element #8=w1269:u16)
              n826 = Equal To 0?(x=w1303) -> (x = 0?=w1302:bool)
              n827 = Equal To 0?(x=w1288) -> (x = 0?=w1292:bool)
              n828 = local read "RewCalib_Trig_L"() -> (w1283:bool)
              n829 = local read "RewCalib_Trig_R"() -> (w1278:bool)
              n830 = Not Equal To 0?(x=w1263) -> (x != 0?=w1301:bool)
              n831 = Not Equal To 0?(x=w1266) -> (x != 0?=w1291:bool)
              n832 = local read "MTrig_Solenoid_Tcycle__L"() -> (w1300:u16)
              n833 = local read "MTrig_Solenoid_Tcycle__R"() -> (w1286:u16)
              n834 = Not Equal To 0?(x=w1272) -> (x != 0?=w1282:bool)
              n835 = Not Equal To 0?(x=w1269) -> (x != 0?=w1280:bool)
              n836 = Not(x=w1283) -> (.not. x?=w1281:bool)
              n837 = Not(x=w1278) -> (.not. x?=w1279:bool)
              n838 = And(x=w1282, y=w1281) -> (x .and. y?=w1277:bool)
              n839 = And(x=w1280, y=w1279) -> (x .and. y?=w1276:bool)
              n840 = call "myRIO_BRig_RT_dataMTrig_Solenoid_c__L.vi"() -> ("output_Solenoid_c__L"=w1309:i32)  [unwired: 11 in]
              n841 = call "myRIO_BRig_RT_dataMTrig_Solenoid_c__R.vi"() -> ("output_Solenoid_c__R"=w1308:i32)  [unwired: 11 in]
              n842 = Select(t=w1300, s=w1301, f=u16 0) -> (s? t:f=w1297:u16)
              n843 = Or(x=w1277, y=w1276) -> (x .or. y?=w1265:bool)
              n844 = Select(t=w1286, s=w1291, f=u16 0) -> (s? t:f=w1289:u16)
              n845 = Select(t=w1297, s=w1302, f=w1298) -> (s? t:f=w1295:u16)
              n846 = Select(t=w1289, s=w1292, f=w1287) -> (s? t:f=w1284:u16)
              n847 = call "myRIO_BRig_RT_dataMTrig_Solenoid_Tcycle__L.vi"() -> ("output_Solenoid_Tcycle__L"=w1296:i32)  [unwired: 11 in]
              n848 = call "myRIO_BRig_RT_dataMTrig_Solenoid_Tcycle__R.vi"() -> ("output_Solenoid_Tcycle__R"=w1285:i32)  [unwired: 11 in]
              n849 = Select(t=w1264, s=w1265, f=w1263) -> (s? t:f=w1261:u16)
              n850 = Select(t=w1264, s=w1265, f=w1266) -> (s? t:f=w1259:u16)
              n851 = Select(t=myRIO_BRig_RT__Case_NonExp_stateList."Idle" ("Enum"), s=w1265, f=myRIO_BRig_RT__Case_NonExp_stateList."DispenseWater" ("Enum")) -> (s? t:f=w1273:T1)
              n852 = Select(t=w1264, s=w1265, f=w1272) -> (s? t:f=w1270:u16)
              n853 = Select(t=w1264, s=w1265, f=w1269) -> (s? t:f=w1268:u16)
              n854 = Replace Array Subset(array=w1306, new element #1=w1307, index #1=w1309, new element #2=w1307, index #2=w1308, new element #3=w1295, index #3=w1296, new element #4=w1284, index #4=w1285, new element #5=w1270, index #5=w1271, new element #6=w1268, index #6=w1267, new element #7=w1261, index #7=w1262, new element #8=w1259, index #8=w1260) -> (w1310:u16[])
            }
            frame "DispenseWater" {
              # "D"
              # "C"
              # "B"
              # "A"
              # "(A) Add COUNT and INCREMENT\n(B) Is (A) smaller than Tcycle?\n(C) Are we dispensing water or in the delay phase?\n(D) If (A) is smaller than Tcycle   AND   if we are dispensing water\n      then send TRUE to solenoid"
              # "delay"
              # "Tcycle"
              # "Solenoid__R"
              # "count"
              # "delay"
              # "Tcycle"
              # "Solenoid__L"
              # "count"
              n855 = To Unsigned Word Integer(number=w1337) -> (unsigned 16bit integer=w1319:u16)
              n856 = call "myRIO_BRig_RT_dataMTrig_Solenoid_delay__R.vi"() -> ("output_Solenoid_delay__R"=w1323:i32)  [unwired: 11 in]
              n857 = call "myRIO_BRig_RT_dataMTrig_Solenoid_c__R.vi"() -> ("output_Solenoid_c__R"=w1322:i32)  [unwired: 11 in]
              n858 = call "myRIO_BRig_RT_dataMTrig_Solenoid_Tcycle__R.vi"() -> ("output_Solenoid_Tcycle__R"=w1324:i32)  [unwired: 11 in]
              n859 = call "myRIO_BRig_RT_dataMTrig_Solenoid_delay__L.vi"() -> ("output_Solenoid_delay__L"=w1339:i32)  [unwired: 11 in]
              n860 = call "myRIO_BRig_RT_dataMTrig_Solenoid_c__L.vi"() -> ("output_Solenoid_c__L"=w1331:i32)  [unwired: 11 in]
              n861 = call "myRIO_BRig_RT_dataMTrig_Solenoid_Tcycle__L.vi"() -> ("output_Solenoid_Tcycle__L"=w1340:i32)  [unwired: 11 in]
              n862 = Index Array(array=w1333, index #1=w1331, index #2=w1340, index #3=w1339, index #4=w1322, index #5=w1324, index #6=w1323) -> (element #1=w1338:u16, element #2=w1328:u16, element #3=w1336:u16, element #4=w1318:u16, element #5=w1315:u16, element #6=w1314:u16)
              n863 = Add(x=w1338, y=w1319) -> (x+y=w1329:u16)
              n864 = Add(x=w1318, y=w1319) -> (x+y=w1320:u16)
              n865 = Less?(x=w1329, y=w1328) -> (x < y?=w1312:bool)
              n866 = Equal To 0?(x=w1336) -> (x = 0?=w1335:bool)
              n867 = Less?(x=w1320, y=w1315) -> (x < y?=w1313:bool)
              n868 = Equal To 0?(x=w1314) -> (x = 0?=w1321:bool)
              n869 = And(x=w1312, y=w1335) -> (x .and. y?=w1334:bool)
              n870 = Or(x=w1312, y=w1313) -> (x .or. y?=w1311:bool)
              n871 = And(x=w1313, y=w1321) -> (x .and. y?=w1316:bool)
              n872 = Select(t=w1329, s=w1312, f=w1328) -> (s? t:f=w1330:u16)
              n873 = Select(t=w1320, s=w1313, f=w1315) -> (s? t:f=w1317:u16)
              n874 = Replace Array Subset(array=w1333, new element #1=w1330, index #1=w1331, new element #2=w1317, index #2=w1322) -> (w1332:u16[])
              n875 = Select(t=w1327, s=w1311, f=myRIO_BRig_RT__Case_NonExp_stateList."DispenseWater_post" ("Enum")) -> (s? t:f=w1325:T1)
            }
            frame "DispenseWater_post" {
              # "nCycle"
              # "delay"
              # "Solenoid__R"
              # "nCycle"
              # "delay"
              # "Solenoid__L"
              n876 = call "myRIO_BRig_RT_dataMTrig_Solenoid_N__L.vi"() -> ("output_Solenoid_N__L"=w1357:i32)  [unwired: 11 in]
              n877 = call "myRIO_BRig_RT_dataMTrig_Solenoid_delay__L.vi"() -> ("output_Solenoid_delay__L"=w1356:i32)  [unwired: 11 in]
              n878 = call "myRIO_BRig_RT_dataMTrig_Solenoid_N__R.vi"() -> ("output_Solenoid_N__R"=w1353:i32)  [unwired: 11 in]
              n879 = call "myRIO_BRig_RT_dataMTrig_Solenoid_delay__R.vi"() -> ("output_Solenoid_delay__R"=w1352:i32)  [unwired: 11 in]
              n880 = Index Array(array=w1359, index #1=w1357, index #2=w1356, index #3=w1353, index #4=w1352) -> (element #1=w1361:u16, element #2=w1360:u16, element #3=w1344:u16, element #4=w1346:u16)
              n881 = Not Equal To 0?(x=w1361) -> (x != 0?=w1362:bool)
              n882 = Not Equal To 0?(x=w1344) -> (x != 0?=w1345:bool)
              n883 = case shown="True" w1345 {
                selector: w1345 -> [_ w1366]
                tunnel: w1344 -> [w1364 w1372]
                tunnel: w1346 -> [_ w1373]
                tunnel: [w1364 w1370] -> w1343
                tunnel: [u16 0 w1369] -> w1342
                tunnel: [_ w1366] -> w1341
                frame False {
                }
                frame True {
                  n884 = Equal To 0?(x=w1373) -> (x = 0?=w1365:bool)
                  n885 = Decrement(x=w1372) -> (x-1=w1371:u16)
                  n886 = Select(t=w1371, s=w1365, f=w1372) -> (s? t:f=w1370:u16)
                  n887 = Select(t=u16 1, s=w1365, f=u16 0) -> (s? t:f=w1369:u16)
                }
              }
              n888 = case shown="True" w1362 {
                selector: w1362 -> [_ w1377]
                tunnel: w1361 -> [w1375 w1383]
                tunnel: w1360 -> [_ w1384]
                tunnel: [w1375 w1381] -> w1355
                tunnel: [u16 0 w1380] -> w1354
                tunnel: [_ w1377] -> w1351
                frame False {
                }
                frame True {
                  n889 = Equal To 0?(x=w1384) -> (x = 0?=w1376:bool)
                  n890 = Decrement(x=w1383) -> (x-1=w1382:u16)
                  n891 = Select(t=w1382, s=w1376, f=w1383) -> (s? t:f=w1381:u16)
                  n892 = Select(t=u16 1, s=w1376, f=u16 0) -> (s? t:f=w1380:u16)
                }
              }
              n893 = Or(x=w1351, y=w1341) -> (x .or. y?=w1350:bool)
              n894 = Replace Array Subset(array=w1359, new element #1=w1355, index #1=w1357, new element #2=w1354, index #2=w1356, new element #3=w1343, index #3=w1353, new element #4=w1342, index #4=w1352) -> (w1358:u16[])
              n895 = Select(t=myRIO_BRig_RT__Case_NonExp_stateList."DispenseWater_pre" ("Enum"), s=w1350, f=myRIO_BRig_RT__Case_NonExp_stateList."Idle" ("Enum")) -> (s? t:f=w1347:T1)
            }
            frame "TestConnection" {
              n896 = local read "Host Password"() -> (w1390:string)
              n897 = local read "Host UserName"() -> (w1391:string)
              n898 = call "myRIO_BRig_RT_comm_webdav_testConnect.vi"("input_password"=w1390, "input_username"=w1391) -> ("output_Iconnected"=w1388:bool)  [unwired: 9 in]
              n899 = Select(t="Connection accepted!" ("message"), s=w1388, f="Error!") -> (s? t:f=w1386:string)
              n900 = One Button Dialog(message=w1386) -> ()  [unwired: 1 in, 1 out]
            }
            frame "SendData" {
              n901 = local read "Data Set Prefix"() -> (w1393:string)
              n902 = local read "Host Password"() -> (w1394:string)
              n903 = local read "Host UserName"() -> (w1395:string)
              n904 = call "myRIO_BRig_RT_comm_webdav_sendData_all.vi"("Host Filename Prefix"=w1393, "Host Password"=w1394, "Host UserName"=w1395) -> ()  [unwired: 9 in]
            }
            frame "Get_FPGA_count_per_ms" {
              # "Used to automatically determine how many FPGA cycles in 1 ms"
              n905 = case shown="False" w1408 {
                selector: w1408 -> [w1410 _]
                tunnel: w1406 -> [_ w1423]
                tunnel: [w1414 w1423] -> w1405
                tunnel: w1404 -> [w1413 w1421]
                tunnel: w1403 -> [w1412 w1420]
                tunnel: [w1411 w1418] -> w1398
                tunnel: [w1410 w1417] -> w1402
                frame False {
                  n906 = Get Date/Time In Seconds() -> (seconds since 1Jan1904=w1415:timestamp)
                  n907 = xnode "Read/Write Control"("FPGA VI Reference In"=w1413, "error in"=w1412, "timeTrial_trig"=TRUE ("timeTrial")) -> ("error out"=w1411:errorcluster)  [unwired: 1 out]
                  n908 = To Double Precision Float(number=w1415) -> (double precision float=w1414:dbl)
                  n909 = local write "get_countPerMS"(w1410) -> ()
                }
                frame True {
                  w1419 = 1.0
                  n910 = Get Date/Time In Seconds() -> (seconds since 1Jan1904=w1424:timestamp)
                  n911 = To Double Precision Float(number=w1424) -> (double precision float=w1425:dbl)
                  n912 = Subtract(x=w1425, y=w1423) -> (x-y=w1422:dbl)
                  n913 = Less Or Equal?(x=w1419, y=w1422) -> (x <= y?=w1417:bool)
                  n914 = case shown="True" w1417 {
                    tunnel: w1421 -> [_ w1438]
                    tunnel: w1420 -> [w1426 w1437]
                    tunnel: w1419 -> [_ w1428]
                    tunnel: [w1426 w1427] -> w1418
                    frame False {
                    }
                    frame True {
                      n915 = xnode "Read/Write Control"("FPGA VI Reference In"=w1438, "error in"=w1437) -> ("FPGA VI Reference Out"=w1435:refnum<k20>, "error out"=w1434:errorcluster, "timeTrial_count"=w1429:u32)
                      n916 = Multiply(x=w1428, y=1000.0) -> (x*y=w1432:dbl)
                      n917 = To Double Precision Float(number=w1429) -> (double precision float=w1431:dbl)
                      n918 = Divide(x=w1431, y=w1432) -> (x/y=w1433:dbl)
                      n919 = local write "FPGA_count2ms"(w1433) -> ()
                      n920 = xnode "Read/Write Control"("FPGA VI Reference In"=w1435, "error in"=w1434, "timeTrial_trig"=FALSE ("timeTrial")) -> ("error out"=w1427:errorcluster)  [unwired: 1 out]
                    }
                  }
                }
              }
              n921 = Select(t=myRIO_BRig_RT__Case_NonExp_stateList."Idle" ("Enum"), s=w1402, f=w1400) -> (s? t:f=w1399:T1)
              n922 = local write "error out"(w1398) -> ()
            }
            frame "End" {
            }
          }
          n923 = local read "MTrig_Audio_trig__R"() -> (w91:bool)
          n924 = local read "MTrig_Audio_trig__L"() -> (w92:bool)
          n925 = local read "MTrig_Laser_trig"() -> (w90:bool)
          n926 = local read "MTrig_CueLed"() -> (w83:bool)
          n927 = Compound Arithmetic op=OR(w92, w91, w90, w83) -> (w89:bool)
          n928 = local read "START"() -> (w115:bool)
          n929 = local read "STOP_abort"() -> (w114:bool)
          n930 = case shown="True" w89 {
            frame False {
            }
            frame True {
              w131 = FALSE
              n931 = local write "MTrig_Audio_trig__R"(w131) -> ()
              n932 = local write "MTrig_Audio_trig__L"(w131) -> ()
              n933 = local write "MTrig_Laser_trig"(w131) -> ()
              n934 = local write "MTrig_CueLed"(w131) -> ()
            }
          }
          n935 = call "myRIO_BRig_RT_dataMTrig_main__NoExp.vi"("input_dataMTrig"=w118, "input_Audio_trig_L"=w92, "input_Audio_trig_R"=w91, "input_Laser_trig"=w90, "input_CueLed"=w83) -> ("output_dataMTrig"=w117:u16[], "output_Audio_L"=w109:bool, "output_Audio_R"=w110:bool, "output_Laser"=w88:bool, "output_CueLed"=w82:bool)  [unwired: 10 in]
          n936 = Or(x=w115, y=w114) -> (x .or. y?=w113:bool)
          n937 = Select(t=myRIO_BRig_RT__Case_NonExp_stateList."End" ("Enum"), s=w113, f=w112) -> (s? t:f=w111:T1)
          n938 = Not(x="MTrig_Laser_Switch") -> (.not. x?=w85:bool)
          n939 = And(x=w88, y=w85) -> (x .and. y?=w86:bool)
          n940 = And(x=w88, y="MTrig_Laser_Switch") -> (x .and. y?=w87:bool)
          n941 = xnode "Read/Write Control"("FPGA VI Reference In"=w98, "error in"=w97, "A1_SR"=w119, "A3_SL"=w120, "audioTrigger_L"=w109, "audioTrigger_R"=w110, "LC_Laser_l1"=w86, "LC_Laser_l2"=w87, "CueLed_Event"=w82) -> ("FPGA VI Reference Out"=w125:refnum<k20>, "error out"=w124:errorcluster)
          n942 = node-c288() -> ()  [unwired: 1 in, 1 out]
          "cState_NonExp" <- w123
        }
        n943 = node-c288(w70) -> ()  [unwired: 1 out]
        n944 = flat-sequence {
          tunnel: w63 -> [w81]
          tunnel: [w81] -> w62
          tunnel: w61 -> [w80]
          tunnel: [w80] -> w60
          frame #0 {
            w79 = FALSE
            n945 = local write "STOP_endBlock"(w79) -> ()
            n946 = local write "STOP_endTrial"(w79) -> ()
          }
        }
      }
      frame True {
        w1451 = u16 0
        w1469 = u8 0
        w1470 = u16 0 ("idxDataBlock")
        w1472 = u16 100 ("new element/subarray")
        w1473 = u16 100 ("new element/subarray")
        w1493 = T6 refnum items=["Session NI_WebDAV"] ("output_hSession")
        w1502 = FALSE
        w1503 = u16 0
        # "dummyState counter"
        # "audio__L\naudio__R"
        # "Audio params"
        # "nRewards"
        # "idxDataBlock"
        # "Solenoid_Tdelay_R"
        # "Solenoid_Tdelay_L"
        # "RewCalib_N__R"
        # "RewCalib_N__L"
        # "Save dataLick to file\nSend file to Host\nSave dataMTrig\nSend file to Host\nDisconnect"
        # "dataTrial"
        # "dataTrial"
        # "Solenoid_Tcycle_R"
        # "Solenoid_Tcycle_L"
        # "Laser_Tcycle"
        # "Audio_Tcycle_R"
        # "Audio_Tcycle_L"
        # "dataLick"
        # "dataLC"
        # "dataLC"
        # "dataBlock"
        # "dataBlock"
        # "dataMTrig"
        # "dataMTrig"
        # "dataExp"
        # "dataCurrent"
        # "dataExp"
        # "dataCurrent"
        # "spout"
        # "state"
        n947 = call "myRIO_BRig_RT_dataMTrig_Solenoid_Tcycle__L.vi"() -> ("output_Solenoid_Tcycle__L"=w1499:i32)  [unwired: 11 in]
        n948 = call "myRIO_BRig_RT_dataMTrig_Solenoid_Tcycle__R.vi"() -> ("output_Solenoid_Tcycle__R"=w1498:i32)  [unwired: 11 in]
        n949 = call "myRIO_BRig_RT_dataMTrig_Audio_Tcycle__L.vi"() -> ("output_Audio_Tcycle__L"=w1497:i32)  [unwired: 11 in]
        n950 = call "myRIO_BRig_RT_dataMTrig_Audio_Tcycle__R.vi"() -> ("output_Audio_Tcycle__R"=w1496:i32)  [unwired: 11 in]
        n951 = call "myRIO_BRig_RT_dataMTrig_Laser_Tcycle.vi"() -> ("output_Laser_Tcycle"=w1495:i32)  [unwired: 11 in]
        n952 = local read "MTrig_Solenoid_Tcycle__L"() -> (w1478:u16)
        n953 = local read "MTrig_Solenoid_Tcycle__R"() -> (w1477:u16)
        n954 = local read "Tcycle_Reward_L"() -> (w1474:u16)
        n955 = local read "Tcycle_Reward_R"() -> (w1475:u16)
        n956 = local read "MTrig_Laser_Tcycle"() -> (w1476:u16)
        n957 = call "myRIO_BRig_RT_dataMTrig_Solenoid_RewCalib_nCycle__L.vi"() -> ("output_Solenoid_RewCalib_nCycle__L"=w1481:i32)  [unwired: 11 in]
        n958 = call "myRIO_BRig_RT_dataMTrig_Solenoid_Tdelay__L.vi"() -> ("output_Solenoid_Tdelay__L"=w1483:i32)  [unwired: 11 in]
        n959 = call "myRIO_BRig_RT_dataMTrig_Solenoid_RewCalib_nCycle__R.vi"() -> ("output_Solenoid_RewCalib_nCycle__R"=w1482:i32)  [unwired: 11 in]
        n960 = call "myRIO_BRig_RT_dataMTrig_Solenoid_Tdelay__R.vi"() -> ("output_Solenoid_Tdelay__R"=w1484:i32)  [unwired: 11 in]
        n961 = case shown="False" w1461 {
          selector: w1461 -> [_ w1525]
          tunnel: w1460 -> [w1522 w1527]
          tunnel: [w1523 w1527] -> w1456
          tunnel: w1459 -> [_ w1526]
          tunnel: [w1524 w1526] -> w1457
          tunnel: [w1521 w1525] -> w1455
          frame False {
            n962 = call "myRIO__TCP_connect_forWriting.vi"("input_error"=w1522) -> ("output_error"=w1523:errorcluster, "output_connected"=w1521:bool, "output_hTCP"=w1524:refnum<k5>)  [unwired: 8 in]
          }
          frame True {
          }
        }
        n963 = call "myRIO_BRig_RT_dataLick_init.vi"() -> ("output_dataLick"=w1505:u16[][])  [unwired: 11 in]
        n964 = call "myRIO_BRig_RT_dataCurrent_init.vi"() -> ("output_dataCurrent"=w1512:u16[])  [unwired: 11 in]
        n965 = call "myRIO_BRig_RT_dataExp_init.vi"() -> ("output_dataExp"=w1511:u16[])  [unwired: 11 in]
        n966 = call "myRIO_BRig_RT_dataMTrig_init.vi"() -> ("output_dataMTrig"=w1501:u16[])  [unwired: 5 in]
        n967 = call "myRIO_BRig_RT_dataLC_init.vi"() -> ("output_dataLC"=w1509:u16[])  [unwired: 11 in]
        n968 = call "myRIO_BRig_RT_dataBlock_init.vi"() -> ("output_dataBlock"=w1510:u16[][])  [unwired: 11 in]
        n969 = call "myRIO_BRig_RT_dataTrial_init.vi"() -> ("output_dataTrial"=w1494:u16[][])  [unwired: 11 in]
        n970 = local write "I_connect_TCP"(w1455) -> ()
        n971 = Replace Array Subset(array=w1501, new element #1=w1473, index #1=w1481, new element #2=w1473, index #2=w1482, new element #3=w1472, index #3=w1483, new element #4=w1472, index #4=w1484, new element #5=w1478, index #5=w1499, new element #6=w1477, index #6=w1498, new element #7=w1474, index #7=w1497, new element #8=w1475, index #8=w1496, new element #9=w1476, index #9=w1495) -> (w1500:u16[])
        n972 = call "myRIO_BRig_RT_dataAnalog_init.vi"() -> ("output_dataAnalog"=w1466:u16[][])  [unwired: 11 in]
        n973 = call "myRIO_BRig_RT_TCP__start_exp.vi"("input_hTCP"=w1457, "input_I_connected_TCP"=w1455, "input_error"=w1456) -> ("output_hTCP"=w1454:refnum<k5>, "output_error"=w1453:errorcluster)  [unwired: 11 in]
        n974 = Get Date/Time In Seconds() -> (seconds since 1Jan1904=w1480:timestamp)
        n975 = call "myRIO_BRig_RT_arrTrig_init.vi"() -> ("output_arrTrig"=w1450:bool[])  [unwired: 11 in]
        n976 = To Double Precision Float(number=w1480) -> (double precision float=w1479:dbl)
        n977 = node-c288() -> (w1520:T3)  [unwired: 4 in]
        n978 = timed-loop {
          timing: w1520 -> [_]
          timing-out: [_] -> w1519
          shift-right: [w1653] -> _
          shift-left: myRIO_BRig_RT__Case_Exp_stateList."Start1" ("Enum") -> [w1571]
          shift-right: [w1605] -> _
          shift-left: enum16{"Left", "Right"}."Left" -> [w1700]
          tunnel: w1449 -> [w1698]
          tunnel: w1448 -> [w1577]
          shift-right: [w1693] -> _
          shift-left: w1517 -> [w1697]
          shift-right: [w1692] -> _
          shift-left: w1516 -> [w1696]
          tunnel: [w1676] -> w1514
          tunnel: [w1677] -> w1515
          shift-right: [w1678] -> w1485
          shift-left: w1512 -> [w1645]
          shift-right: [w1691] -> _
          shift-left: w1511 -> [w1643]
          shift-right: [w1665] -> w1489
          shift-left: w1500 -> [w1666]
          shift-right: [w1689] -> _
          shift-left: w1510 -> [w1690]
          shift-right: [w1687] -> _
          shift-left: w1509 -> [w1688]
          shift-right: [w1679] -> w1491
          shift-left: w1505 -> [w1680]
          shift-right: [w1667] -> _
          shift-left: w1503 -> [w1675]
          shift-right: [w1640] -> _
          shift-left: w1469 -> [w1674]
          shift-right: [w1668] -> _
          shift-left: w1503 -> [w1673]
          shift-right: [w1669] -> _
          shift-left: w1469 -> [w1672]
          shift-right: [w1641] -> _
          shift-left: w1502 -> [w1670]
          shift-right: [w1642] -> _
          shift-left: w1502 -> [w1671]
          shift-right: [w1651] -> _
          shift-left: w1494 -> [w1652]
          shift-right: [w1650] -> w1487
          shift-left: w1493 -> [w1648]
          shift-right: [w1649] -> w1488
          shift-left: FALSE ("output_Iconnected") -> [w1647]
          tunnel: "Data Set Prefix" -> [w1646]
          tunnel: [w1646] -> w1486
          tunnel: w1479 -> [w1644]
          shift-right: [w1638] -> _
          shift-left: 0 ("idxDataBlock") -> [w1639]
          shift-right: [w1635] -> _
          shift-left: w1470 -> [w1637]
          shift-right: [w1634] -> _
          shift-left: w1470 -> [w1636]
          shift-right: [w1624] -> w1464
          shift-left: 0 -> [w1610]
          shift-right: [w1606] -> _
          shift-left: w1451 -> [w1619]
          shift-right: [w1607] -> _
          shift-left: w1451 -> [w1616]
          shift-right: [w1628] -> _
          shift-left: FALSE -> [w1628]
          shift-right: [w1615] -> _
          shift-left: w1451 -> [w1622]
          shift-right: [w1625] -> w1465
          shift-left: w1466 -> [w1626]
          tunnel: w1454 -> [w1614]
          tunnel: [w1613] -> w1463
          tunnel: w1455 -> [w1611]
          tunnel: [w1611] -> w1462
          tunnel: w1453 -> [w1612]
          tunnel: [w1574] -> w1458
          shift-right: [w1603] -> _
          shift-left: u16 0 -> [w1604]
          shift-right: [w1601] -> _
          shift-left: w1451 -> [w1602]
          shift-right: [w1598] -> _
          shift-left: w1450 -> [w1599]
          shift-right: [w1569] -> _
          shift-left: FALSE -> [w1572]
          stop <- w1686 stop-if-true
          # "arrTrig"
          # "arrTrig"
          # "LC_Laser_l2"
          # "LC_Event_l2"
          # "LC_Laser_l1"
          # "LC_Event_l1"
          # "CueLed"
          # "LC_Laser_l2"
          # "LC_Event_l2"
          # "LC_Laser_l1"
          # "LC_Event_l1"
          # "solenoid__R"
          # "solenoid__L"
          # "spout"
          # "iState"
          # "dataAnalog"
          # "index"
          # "iEvent"
          # "iBlock"
          # "iTrial"
          # "Laser"
          # "Audio R"
          # "Audio L"
          # "Solenoid R"
          # "Solenoid L"
          # "manual triggering"
          # "dataTrial"
          # "dataBlock"
          # "nRewards"
          # "dataExp"
          # "dataCurrent"
          # "audio__L\naudio__R"
          # "time stamp"
          # "Audio params"
          # "nRewards"
          # "idxDataBlock"
          # "idxDataBlock"
          # "activate"
          # "audio__L\naudio__R"
          # "amp__R\nfreq__R"
          # "amp__L\nfreq__L"
          # "dataLC"
          # "solenoid__R"
          # "solenoid__L"
          # "Did a lick occur?"
          # "Update lick counter"
          # "spout"
          # "spout"
          # "state"
          # "state"
          n979 = node-c288() -> ()  [unwired: 1 in, 1 out]
          n980 = flat-sequence {
            tunnel: w1577 -> [w1701]
            tunnel: [w1701] -> _
            tunnel: [w1702] -> w1573
            tunnel: [w1701] -> w1576
            frame #0 {
              n981 = Get Date/Time In Seconds() -> (seconds since 1Jan1904=w1702:timestamp)
            }
          }
          n982 = xnode "Read/Write Control"("FPGA VI Reference In"=w1698, "error in"=w1576) -> ("FPGA VI Reference Out"=w1633:refnum<k20>, "error out"=w1632:errorcluster, "A2_LickL"=w1693:u32, "A4_LickR"=w1692:u32)
          "A2" <- w1693
          "A4" <- w1692
          n983 = Greater?(x=w1693, y=w1697) -> (0:w1695:bool)
          n984 = Greater?(x=w1692, y=w1696) -> (0:w1694:bool)
          n985 = Or(x=w1695, y=w1694) -> (x .or. y?=w1699:bool)
          n986 = local read "MTrig_Solenoid_trig__L"() -> (w1663:bool)
          n987 = local read "MTrig_Solenoid_trig__R"() -> (w1662:bool)
          n988 = local read "MTrig_Audio_trig__L"() -> (w1661:bool)
          n989 = local read "MTrig_Audio_trig__R"() -> (w1660:bool)
          n990 = local read "MTrig_Laser_trig"() -> (w1659:bool)
          n991 = case shown="\"initTrial_LC_Sel\"" w1571 {
            selector: w1571 -> [_ _ _ _ _ _ _ _ _ _ _ _ _ _ _ _ _ _ _ _ _ _ _ _ _ _ w2768 _ w2823 _ _ _ _ _ w2940 _ w3013 _ _ _ _ _ w3133 _ w3203 _ w3267 _ w3311 _ _ w3381 _ _ _ _ _ w3552 _ _ _ _ _ _ _ _ _ _ _ _ w3833 w3866]
            tunnel: [myRIO_BRig_RT__Case_Exp_stateList."Start2" ("Enum") myRIO_BRig_RT__Case_Exp_stateList."Start3" ("Enum") myRIO_BRig_RT__Case_Exp_stateList."saveSettings1" ("Enum") myRIO_BRig_RT__Case_Exp_stateList."saveSettings2" ("Enum") myRIO_BRig_RT__Case_Exp_stateList."saveSettings3" ("Enum") myRIO_BRig_RT__Case_Exp_stateList."saveSettings4" ("Enum") myRIO_BRig_RT__Case_Exp_stateList."saveSettings_LC_ENL_l1" ("Enum") myRIO_BRig_RT__Case_Exp_stateList."saveSettings_LC_ENL_l2" ("Enum") myRIO_BRig_RT__Case_Exp_stateList."saveSettings_LC_Cue_l1" ("Enum") myRIO_BRig_RT__Case_Exp_stateList."saveSettings_LC_Cue_l2" ("Enum") myRIO_BRig_RT__Case_Exp_stateList."saveSettings6_LC_l1_Other" ("Enum") myRIO_BRig_RT__Case_Exp_stateList."SaveSettings6_LC_l2_Other" ("Enum") myRIO_BRig_RT__Case_Exp_stateList."setSettings_Audio" ("Enum") myRIO_BRig_RT__Case_Exp_stateList."setSettings_Laser" ("Enum") myRIO_BRig_RT__Case_Exp_stateList."commConnect" ("Enum") w2463 myRIO_BRig_RT__Case_Exp_stateList."initTrial" ("Enum") w2529 myRIO_BRig_RT__Case_Exp_stateList."initTrial3" ("Enum") myRIO_BRig_RT__Case_Exp_stateList."initTrial_LC_ENL1" ("Enum") myRIO_BRig_RT__Case_Exp_stateList."ENL1_pre" ("Enum") myRIO_BRig_RT__Case_Exp_stateList."initTrial_LC_Cue1" ("Enum") myRIO_BRig_RT__Case_Exp_stateList."initTrial_LC_Sel" ("Enum") myRIO_BRig_RT__Case_Exp_stateList."initTrial_LC_Sel" ("Enum") myRIO_BRig_RT__Case_Exp_stateList."initTrial4" ("Enum") w2739 w2765 myRIO_BRig_RT__Case_Exp_stateList."ENL1Penalty" ("Enum") w2824 myRIO_BRig_RT__Case_Exp_stateList."endExp" ("Enum") myRIO_BRig_RT__Case_Exp_stateList."endExp" ("Enum") myRIO_BRig_RT__Case_Exp_stateList."endExp" ("Enum") myRIO_BRig_RT__Case_Exp_stateList."endExp" ("Enum") w2913 w2939 myRIO_BRig_RT__Case_Exp_stateList."Cue1Penalty" ("Enum") w3011 myRIO_BRig_RT__Case_Exp_stateList."endExp" ("Enum") myRIO_BRig_RT__Case_Exp_stateList."endExp" ("Enum") myRIO_BRig_RT__Case_Exp_stateList."endExp" ("Enum") myRIO_BRig_RT__Case_Exp_stateList."endExp" ("Enum") w3103 w3132 myRIO_BRig_RT__Case_Exp_stateList."SelectReward" ("Enum") w3204 myRIO_BRig_RT__Case_Exp_stateList."SelectRewardPost" ("Enum") w3268 myRIO_BRig_RT__Case_Exp_stateList."SelectWrong" ("Enum") w3307 myRIO_BRig_RT__Case_Exp_stateList."endTrial1" ("Enum") myRIO_BRig_RT__Case_Exp_stateList."SelectTimeout" ("Enum") w3383 myRIO_BRig_RT__Case_Exp_stateList."endTrial1" ("Enum") myRIO_BRig_RT__Case_Exp_stateList."endTrial2" ("Enum") myRIO_BRig_RT__Case_Exp_stateList."endTrial3" ("Enum") w3469 w3535 w3552 myRIO_BRig_RT__Case_Exp_stateList."initBlock" ("Enum") w3579 myRIO_BRig_RT__Case_Exp_stateList."commUpload_dataExp" ("Enum") myRIO_BRig_RT__Case_Exp_stateList."endBlock" ("Enum") myRIO_BRig_RT__Case_Exp_stateList."commUpload_dataLC" ("Enum") myRIO_BRig_RT__Case_Exp_stateList."commUpload_dataTrial" ("Enum") myRIO_BRig_RT__Case_Exp_stateList."commUpload_dataCurrent" ("Enum") myRIO_BRig_RT__Case_Exp_stateList."saveData_dataCurrent" ("Enum") myRIO_BRig_RT__Case_Exp_stateList."saveData_dataExp" ("Enum") myRIO_BRig_RT__Case_Exp_stateList."saveData_dataLC" ("Enum") myRIO_BRig_RT__Case_Exp_stateList."saveData_dataTrial" ("Enum") myRIO_BRig_RT__Case_Exp_stateList."commUpload_pre" ("Enum") w3832 w3865] -> w1653
            tunnel: [w1732 w1751 w1773 w1834 w1894 w1960 w2023 w2087 w2151 w2215 w2279 w2322 w2366 w2392 w2454 w2462 w2491 w2512 w2544 w2591 w2620 w2645 w2667 w2684 w2721 w2753 w2781 w2806 w2828 w2844 w2866 w2885 w2904 w2912 w2961 w2989 w3010 w3031 w3052 w3071 w3090 w3113 w3153 w3178 w3201 w3215 w3265 w3289 w3321 w3342 w3362 w3393 w3416 w3428 w3448 w3489 w3508 w3551 w3568 w3582 w3616 w3637 w3658 w3679 w3700 w3728 w3748 w3775 w3795 w3819 w3853 w3886] -> w1605
            tunnel: w1700 -> [w1732 w1751 w1773 w1834 w1894 w1960 w2023 w2087 w2151 w2215 w2279 w2322 w2366 w2392 w2454 w2464 w2491 w2512 w2544 w2591 w2620 w2645 w2667 w2684 w2721 w2753 w2781 w2806 w2828 w2844 w2866 w2885 w2904 w2912 w2961 w2989 w3010 w3031 w3052 w3071 w3090 w3113 w3153 w3178 w3201 w3215 w3265 w3289 w3321 w3342 w3362 w3393 w3416 w3428 w3448 w3489 w3508 w3551 w3568 w3582 w3616 w3637 w3658 w3679 w3700 w3728 w3748 w3775 w3795 w3819 w3853 w3886]
            tunnel: w1699 -> [w1735 w1754 w1770 w1837 w1897 w1963 w2026 w2090 w2154 w2218 w2282 w2325 w2369 w2395 w2457 w2483 w2502 w2530 w2568 w2606 w2634 w2657 w2680 w2709 w2734 w2740 w2764 w2809 w2831 w2850 w2869 w2888 w2907 w2916 w2938 w2995 w3017 w3036 w3055 w3074 w3093 w3111 w3151 w3188 w3211 w3246 w3273 w3300 w3324 w3341 w3374 w3398 w3413 w3436 w3447 w3500 w3534 w3555 w3565 w3591 w3619 w3640 w3661 w3682 w3703 w3731 w3751 w3778 w3798 w3822 w3856 w3889]
            tunnel: w1695 -> [w1734 w1753 w1771 w1836 w1896 w1962 w2025 w2089 w2153 w2217 w2281 w2324 w2368 w2394 w2456 w2482 w2501 w2531 w2567 w2607 w2635 w2658 w2681 w2710 w2735 w2757 w2783 w2808 w2830 w2849 w2868 w2887 w2906 w2930 w2962 w2994 w3016 w3035 w3054 w3073 w3092 w3112 w3150 w3187 w3210 w3245 w3272 w3299 w3323 w3340 w3373 w3397 w3414 w3437 w3446 w3499 w3533 w3554 w3566 w3592 w3618 w3639 w3660 w3681 w3702 w3730 w3750 w3777 w3797 w3821 w3855 w3888]
            tunnel: w1694 -> [w1733 w1752 w1772 w1835 w1895 w1961 w2024 w2088 w2152 w2216 w2280 w2323 w2367 w2393 w2455 w2481 w2500 w2532 w2566 w2608 w2636 w2659 w2682 w2711 w2736 w2756 w2782 w2807 w2829 w2848 w2867 w2886 w2905 w2929 w2963 w2993 w3015 w3034 w3053 w3072 w3091 w3123 w3154 w3186 w3209 w3244 w3271 w3298 w3322 w3339 w3372 w3396 w3415 w3438 w3445 w3498 w3532 w3553 w3567 w3593 w3617 w3638 w3659 w3680 w3701 w3729 w3749 w3776 w3796 w3820 w3854 w3887]
            tunnel: [w1735 w1754 w1770 w1837 w1897 w1963 w2026 w2090 w2154 w2218 w2282 w2325 w2369 w2395 w2457 w2483 w2502 w2530 w2568 w2606 w2634 w2657 w2680 w2709 w2734 w2740 w2764 w2809 w2831 w2850 w2869 w2888 w2907 w2916 w2938 w2995 w3017 w3036 w3055 w3074 w3093 w3111 w3151 w3188 w3211 w3246 w3273 w3300 w3324 w3341 w3374 w3398 w3413 w3436 w3447 w3500 w3534 w3555 w3565 w3591 w3619 w3640 w3661 w3682 w3703 w3731 w3751 w3778 w3798 w3822 w3856 w3889] -> w1683
            tunnel: [w1734 w1753 w1771 w1836 w1896 w1962 w2025 w2089 w2153 w2217 w2281 w2324 w2368 w2394 w2456 w2482 w2501 w2531 w2567 w2607 w2635 w2658 w2681 w2710 w2735 w2757 w2783 w2808 w2830 w2849 w2868 w2887 w2906 w2930 w2962 w2994 w3016 w3035 w3054 w3073 w3092 w3112 w3150 w3187 w3210 w3245 w3272 w3299 w3323 w3340 w3373 w3397 w3414 w3437 w3446 w3499 w3533 w3554 w3566 w3592 w3618 w3639 w3660 w3681 w3702 w3730 w3750 w3777 w3797 w3821 w3855 w3888] -> w1682
            tunnel: [w1733 w1752 w1772 w1835 w1895 w1961 w2024 w2088 w2152 w2216 w2280 w2323 w2367 w2393 w2455 w2481 w2500 w2532 w2566 w2608 w2636 w2659 w2682 w2711 w2736 w2756 w2782 w2807 w2829 w2848 w2867 w2886 w2905 w2929 w2963 w2993 w3015 w3034 w3053 w3072 w3091 w3123 w3154 w3186 w3209 w3244 w3271 w3298 w3322 w3339 w3372 w3396 w3415 w3438 w3445 w3498 w3532 w3553 w3567 w3593 w3617 w3638 w3659 w3680 w3701 w3729 w3749 w3776 w3796 w3820 w3854 w3887] -> w1681
            tunnel: w1645 -> [w1731 w1750 w1769 w1801 w1870 w1898 w1964 w2086 w2150 w2214 w2278 w2321 w2365 w2390 w2404 w2470 w2490 w2528 w2543 w2578 w2619 w2644 w2666 w2694 w2720 w2741 w2767 w2800 w2827 w2845 w2865 w2884 w2903 w2915 w2958 w2988 w3014 w3032 w3051 w3070 w3089 w3105 w3135 w3170 w3206 w3217 w3270 w3290 w3320 w3338 w3363 w3395 w3412 w3425 w3450 w3471 w3506 w3550 w3569 w3594 w3613 w3634 w3655 w3676 w3687 w3717 w3736 w3760 w3792 w3808 w3831 w3864]
            tunnel: w1643 -> [w1730 w1749 w1768 w1832 w1892 w1957 w2020 w2084 w2148 w2212 w2276 w2319 w2363 w2383 w2396 w2467 w2499 w2527 w2551 w2573 w2622 w2637 w2670 w2699 w2724 w2755 w2780 w2799 w2825 w2847 w2864 w2883 w2902 w2911 w2960 w2986 w3009 w3033 w3050 w3069 w3088 w3095 w3152 w3184 w3208 w3238 w3266 w3291 w3318 w3337 w3365 w3392 w3411 w3435 w3439 w3470 w3525 w3549 w3570 w3595 w3612 w3633 w3654 w3675 w3688 w3725 w3745 w3756 w3791 w3816 w3850 w3883]
            tunnel: [w1731 w1750 w1769 w1801 w1870 w1898 w1964 w2086 w2150 w2214 w2278 w2321 w2365 w2390 w2403 w2469 w2490 w2517 w2543 w2577 w2619 w2643 w2665 w2693 w2719 w2738 w2766 w2801 w2826 w2845 w2865 w2884 w2903 w2914 w2957 w2987 w3012 w3032 w3051 w3070 w3089 w3104 w3134 w3185 w3205 w3239 w3269 w3292 w3319 w3338 w3366 w3394 w3412 w3424 w3449 w3471 w3504 w3550 w3569 w3594 w3613 w3634 w3655 w3676 w3687 w3717 w3736 w3760 w3792 w3808 w3831 w3864] -> w1579
            tunnel: [w1730 w1749 w1768 w1831 w1891 w1952 w2019 w2084 w2148 w2212 w2276 w2319 w2363 w2383 w2396 w2468 w2499 w2526 w2551 w2573 w2622 w2637 w2670 w2699 w2724 w2755 w2780 w2799 w2825 w2847 w2864 w2883 w2902 w2911 w2960 w2986 w3009 w3033 w3050 w3069 w3088 w3095 w3152 w3184 w3208 w3238 w3266 w3291 w3318 w3337 w3365 w3392 w3411 w3435 w3439 w3470 w3525 w3549 w3570 w3595 w3612 w3633 w3654 w3675 w3688 w3725 w3745 w3759 w3791 w3816 w3850 w3883] -> w1691
            tunnel: [_ _ _ _ _ _ _ _ _ _ _ _ _ _ _ _ _ _ _ _ _ _ _ _ _ _ _ _ _ _ _ _ _ _ _ _ _ _ _ _ _ _ _ _ w3199 _ _ _ _ _ _ _ _ _ _ _ _ _ _ _ _ _ _ _ _ _ _ _ _ _ _ _] -> w1596
            tunnel: [_ _ _ _ _ _ _ _ _ _ _ _ _ _ _ _ _ _ _ _ _ _ _ _ _ _ _ _ _ _ _ _ _ _ _ _ _ _ _ _ _ _ _ _ w3200 _ _ _ _ _ _ _ _ _ _ _ _ _ _ _ _ _ _ _ _ _ _ _ _ _ _ _] -> w1656
            tunnel: w1690 -> [w1728 w1747 w1766 w1803 w1872 w1958 w2021 w2085 w2149 w2213 w2277 w2320 w2364 w2388 w2451 w2459 w2492 w2507 w2559 w2604 w2632 w2640 w2662 w2683 w2716 w2754 w2779 w2796 w2821 w2846 w2862 w2881 w2900 w2928 w2959 w2985 w3007 w3029 w3048 w3067 w3086 w3122 w3148 w3176 w3207 w3219 w3263 w3288 w3316 w3335 w3364 w3391 w3409 w3427 w3454 w3496 w3517 w3547 w3572 w3597 w3610 w3631 w3652 w3673 w3697 w3711 w3738 w3766 w3785 w3810 w3844 w3877]
            tunnel: [w1728 w1747 w1766 w1803 w1872 w1958 w2021 w2085 w2149 w2213 w2277 w2320 w2364 w2388 w2451 w2458 w2489 w2507 w2559 w2604 w2632 w2640 w2662 w2683 w2716 w2754 w2779 w2796 w2821 w2846 w2862 w2881 w2900 w2928 w2959 w2985 w3007 w3029 w3048 w3067 w3086 w3122 w3148 w3176 w3207 w3218 w3263 w3288 w3316 w3335 w3364 w3391 w3409 w3426 w3454 w3496 w3517 w3547 w3572 w3597 w3610 w3631 w3652 w3673 w3697 w3711 w3738 w3766 w3785 w3810 w3844 w3877] -> w1689
            tunnel: w1688 -> [w1729 w1748 w1767 w1802 w1871 w1959 w2022 w2082 w2146 w2210 w2274 w2317 w2361 w2389 w2452 w2484 w2498 w2525 w2542 w2605 w2633 w2646 w2668 w2697 w2722 w2752 w2763 w2797 w2822 w2843 w2863 w2882 w2901 w2927 w2937 w2984 w3008 w3030 w3049 w3068 w3087 w3121 w3149 w3177 w3202 w3236 w3264 w3287 w3317 w3336 w3361 w3390 w3410 w3434 w3453 w3497 w3524 w3548 w3571 w3596 w3611 w3632 w3653 w3674 w3698 w3724 w3744 w3772 w3783 w3815 w3849 w3882]
            tunnel: [w1729 w1748 w1767 w1802 w1871 w1959 w2022 w2083 w2147 w2211 w2275 w2318 w2362 w2389 w2452 w2484 w2498 w2525 w2542 w2605 w2633 w2646 w2668 w2697 w2722 w2752 w2763 w2797 w2822 w2843 w2863 w2882 w2901 w2927 w2937 w2984 w3008 w3030 w3049 w3068 w3087 w3121 w3149 w3177 w3202 w3236 w3264 w3287 w3317 w3336 w3361 w3390 w3410 w3434 w3453 w3497 w3524 w3548 w3571 w3596 w3611 w3632 w3653 w3674 w3698 w3724 w3744 w3772 w3783 w3815 w3849 w3882] -> w1687
            tunnel: [_ _ _ _ _ _ _ _ _ _ _ _ _ _ _ _ _ _ _ _ _ _ _ _ _ _ _ _ _ _ _ _ _ _ _ _ _ _ _ _ _ _ _ _ _ _ _ _ _ _ _ _ _ _ _ _ _ TRUE _ _ _ _ _ _ _ _ _ _ _ _ _ _] -> w1684
            tunnel: w1675 -> [w1726 w1745 w1764 w1793 w1865 w1947 w2018 w2069 w2138 w2197 w2261 w2289 w2343 _ w2443 w2480 w2497 w2524 w2558 w2603 w2631 w2656 w2679 w2708 w2733 w2751 w2778 w2794 w2820 w2841 w2860 w2879 w2898 w2926 w2954 w2982 w3006 w3027 w3046 w3065 w3084 w3120 w3147 w3166 w3198 w3234 w3262 w3285 w3315 w3334 w3359 w3389 w3408 w3432 w3458 w3495 w3521 w3545 w3563 w3590 w3608 w3629 w3650 w3671 w3695 w3722 w3742 w3770 w3789 w3814 w3848 w3881]
            tunnel: w1674 -> [w1725 w1744 w1763 w1792 w1864 w1946 w2017 w2068 w2137 w2196 w2260 w2290 w2344 _ w2442 w2479 w2496 w2523 w2557 w2602 w2630 w2655 w2678 w2707 w2732 w2750 w2777 w2793 w2819 w2840 w2859 w2878 w2897 w2925 w2953 w2981 w3005 w3026 w3045 w3064 w3083 w3119 w3146 w3165 w3197 w3233 w3261 w3284 w3314 w3333 w3358 w3388 w3407 w3431 w3457 w3494 w3520 w3544 w3562 w3589 w3607 w3628 w3649 w3670 w3694 w3721 w3741 w3769 w3788 w3813 w3847 w3880]
            tunnel: w1673 -> [w1724 w1743 w1762 w1791 w1863 w1945 w2016 w2067 w2136 w2195 w2259 w2291 w2345 _ w2441 w2478 w2495 w2522 w2556 w2601 w2629 w2654 w2677 w2706 w2731 w2749 w2776 w2792 w2818 w2839 w2858 w2877 w2896 w2924 w2952 w2980 w3004 w3025 w3044 w3063 w3082 w3118 w3145 w3164 w3196 w3232 w3260 w3283 w3313 w3332 w3357 w3387 w3406 w3430 w3456 w3493 w3519 w3543 w3561 w3588 w3606 w3627 w3648 w3669 w3693 w3720 w3740 w3768 w3787 w3812 w3846 w3879]
            tunnel: w1672 -> [w1723 w1742 w1761 w1790 w1862 w1944 w2015 w2066 w2135 w2194 w2258 w2292 w2346 _ w2440 w2477 w2494 w2521 w2555 w2600 w2628 w2653 w2676 w2705 w2730 w2748 w2775 w2791 w2817 w2838 w2857 w2876 w2895 w2923 w2951 w2979 w3003 w3024 w3043 w3062 w3081 w3117 w3144 w3163 w3195 w3231 w3259 w3282 w3312 w3331 w3356 w3386 w3405 w3429 w3455 w3492 w3518 w3542 w3560 w3587 w3605 w3626 w3647 w3668 w3692 w3719 w3739 w3767 w3786 w3811 w3845 w3878]
            tunnel: w1671 -> [_ _ _ _ _ _ _ _ _ _ _ _ _ _ _ _ _ _ _ _ _ _ _ _ _ _ _ _ _ _ _ _ _ _ w2956 _ _ _ _ _ _ _ _ _ _ _ _ _ _ _ _ _ _ _ _ _ _ _ _ _ _ _ _ _ _ _ _ _ _ _ _ _]
            tunnel: w1670 -> [_ _ _ _ _ _ _ _ _ _ _ _ _ _ _ _ _ _ _ _ _ _ _ _ _ _ _ _ _ _ _ _ _ _ w2955 _ _ _ _ _ _ _ _ _ _ _ _ _ _ _ _ _ _ _ _ _ _ _ _ _ _ _ _ _ _ _ _ _ _ _ _ _]
            tunnel: [w1726 w1745 w1764 w1793 w1865 w1947 w2018 w2069 w2138 w2197 w2261 w2289 w2343 w2382 w2443 w2480 w2497 w2524 w2558 w2603 w2631 w2656 w2679 w2708 w2733 w2751 w2778 w2794 w2820 w2841 w2860 w2879 w2898 w2926 w2954 w2982 w3006 w3027 w3046 w3065 w3084 w3120 w3147 w3166 w3198 w3234 w3262 w3285 w3315 w3334 w3359 w3389 w3408 w3432 w3458 w3495 w3521 w3545 w3563 w3590 w3608 w3629 w3650 w3671 w3695 w3722 w3742 w3770 w3789 w3814 w3848 w3881] -> w1667
            tunnel: [w1725 w1744 w1763 w1792 w1864 w1946 w2017 w2068 w2137 w2196 w2260 w2290 w2344 w2373 w2442 w2479 w2496 w2523 w2557 w2602 w2630 w2655 w2678 w2707 w2732 w2750 w2777 w2793 w2819 w2840 w2859 w2878 w2897 w2925 w2953 w2981 w3005 w3026 w3045 w3064 w3083 w3119 w3146 w3165 w3197 w3233 w3261 w3284 w3314 w3333 w3358 w3388 w3407 w3431 w3457 w3494 w3520 w3544 w3562 w3589 w3607 w3628 w3649 w3670 w3694 w3721 w3741 w3769 w3788 w3813 w3847 w3880] -> w1640
            tunnel: [w1724 w1743 w1762 w1791 w1863 w1945 w2016 w2067 w2136 w2195 w2259 w2291 w2345 w2381 w2441 w2478 w2495 w2522 w2556 w2601 w2629 w2654 w2677 w2706 w2731 w2749 w2776 w2792 w2818 w2839 w2858 w2877 w2896 w2924 w2952 w2980 w3004 w3025 w3044 w3063 w3082 w3118 w3145 w3164 w3196 w3232 w3260 w3283 w3313 w3332 w3357 w3387 w3406 w3430 w3456 w3493 w3519 w3543 w3561 w3588 w3606 w3627 w3648 w3669 w3693 w3720 w3740 w3768 w3787 w3812 w3846 w3879] -> w1668
            tunnel: [w1723 w1742 w1761 w1790 w1862 w1944 w2015 w2066 w2135 w2194 w2258 w2292 w2346 w2371 w2440 w2477 w2494 w2521 w2555 w2600 w2628 w2653 w2676 w2705 w2730 w2748 w2775 w2791 w2817 w2838 w2857 w2876 w2895 w2923 w2951 w2979 w3003 w3024 w3043 w3062 w3081 w3117 w3144 w3163 w3195 w3231 w3259 w3282 w3312 w3331 w3356 w3386 w3405 w3429 w3455 w3492 w3518 w3542 w3560 w3587 w3605 w3626 w3647 w3668 w3692 w3719 w3739 w3767 w3786 w3811 w3845 w3878] -> w1669
            tunnel: [_ _ _ _ _ _ _ _ _ _ _ _ _ _ _ _ _ _ _ _ _ _ _ _ _ _ _ _ _ _ _ _ _ w2910 w2956 _ _ _ _ _ _ _ _ _ _ _ _ _ _ _ _ _ _ _ _ _ _ _ _ _ _ _ _ _ _ _ _ _ _ _ _ _] -> w1642
            tunnel: [_ _ _ _ _ _ _ _ _ _ _ _ _ _ _ _ _ _ _ _ _ _ _ _ _ _ _ _ _ _ _ _ _ w2909 w2955 _ _ _ _ _ _ _ _ _ _ _ _ _ _ _ _ _ _ _ _ _ _ _ _ _ _ _ _ _ _ _ _ _ _ _ _ _] -> w1641
            tunnel: w1652 -> [w1722 w1741 w1760 w1789 w1861 w1943 w2014 w2065 w2134 w2193 w2257 w2288 w2342 w2380 w2450 w2476 w2493 w2520 w2546 w2593 w2618 w2642 w2664 w2695 w2718 w2747 w2774 w2790 w2816 w2837 w2856 w2875 w2894 w2922 w2950 w2978 w3002 w3023 w3042 w3061 w3080 w3116 w3143 w3160 w3194 w3230 w3258 w3279 w3306 w3330 w3353 w3380 w3404 w3423 w3452 w3485 w3516 w3541 w3573 w3598 w3609 w3630 w3651 w3672 w3696 w3723 w3743 w3771 w3790 w3805 w3843 w3876]
            tunnel: [w1722 w1741 w1760 w1789 w1861 w1943 w2014 w2065 w2134 w2193 w2257 w2288 w2342 w2380 w2450 w2476 w2493 w2520 w2545 w2592 w2611 w2641 w2663 w2695 w2717 w2747 w2774 w2790 w2816 w2837 w2856 w2875 w2894 w2922 w2950 w2978 w3002 w3023 w3042 w3061 w3080 w3116 w3143 w3160 w3194 w3230 w3258 w3279 w3306 w3330 w3353 w3380 w3404 w3423 w3451 w3485 w3516 w3541 w3573 w3598 w3609 w3630 w3651 w3672 w3696 w3723 w3743 w3771 w3790 w3805 w3843 w3876] -> w1651
            tunnel: [w1721 w1740 w1759 w1788 w1860 w1942 w2013 w2064 w2133 w2192 w2256 w2287 w2341 w2379 w2449 w2475 w2504 w2519 w2561 w2599 w2627 w2652 w2675 w2704 w2729 w2746 w2773 w2789 w2815 w2836 w2855 w2874 w2893 w2921 w2949 w2977 w3001 w3022 w3041 w3060 w3079 w3115 w3142 w3159 w3193 w3229 w3257 w3278 w3305 w3329 w3352 w3379 w3403 w3422 w3444 w3491 w3515 w3539 w3574 w3584 w3604 w3625 w3646 w3667 w3691 w3727 w3747 w3774 w3794 w3818 w3852 w3885] -> w1650
            tunnel: [w1720 w1739 w1758 w1787 w1859 w1941 w2012 w2063 w2132 w2191 w2255 w2286 w2340 w2378 w2448 w2474 w2503 w2518 w2560 w2598 w2626 w2651 w2674 w2703 w2728 w2745 w2772 w2788 w2814 w2835 w2854 w2873 w2892 w2920 w2948 w2976 w3000 w3021 w3040 w3059 w3078 w3114 w3141 w3158 w3192 w3228 w3256 w3277 w3304 w3328 w3351 w3378 w3402 w3421 w3443 w3490 w3514 w3540 w3556 w3581 w3614 w3635 w3656 w3677 w3699 w3726 w3746 w3773 w3793 w3817 w3851 w3884] -> w1649
            tunnel: w1648 -> [w1721 w1740 w1759 w1788 w1860 w1942 w2013 w2064 w2133 w2192 w2256 w2287 w2341 w2379 w2449 w2475 w2504 w2519 w2561 w2599 w2627 w2652 w2675 w2704 w2729 w2746 w2773 w2789 w2815 w2836 w2855 w2874 w2893 w2921 w2949 w2977 w3001 w3022 w3041 w3060 w3079 w3115 w3142 w3159 w3193 w3229 w3257 w3278 w3305 w3329 w3352 w3379 w3403 w3422 w3444 w3491 w3515 w3539 _ w3584 w3604 w3625 w3646 w3667 w3691 w3727 w3747 w3774 w3794 w3818 w3852 w3885]
            tunnel: w1647 -> [w1720 w1739 w1758 w1787 w1859 w1941 w2012 w2063 w2132 w2191 w2255 w2286 w2340 w2378 w2448 w2474 w2503 w2518 w2560 w2598 w2626 w2651 w2674 w2703 w2728 w2745 w2772 w2788 w2814 w2835 w2854 w2873 w2892 w2920 w2948 w2976 w3000 w3021 w3040 w3059 w3078 w3114 w3141 w3158 w3192 w3228 w3256 w3277 w3304 w3328 w3351 w3378 w3402 w3421 w3443 w3490 w3514 w3540 _ w3581 w3614 w3635 w3656 w3677 w3699 w3726 w3746 w3773 w3793 w3817 w3851 w3884]
            tunnel: w1646 -> [_ _ _ _ _ _ _ _ _ _ _ _ _ _ _ _ _ _ _ _ _ _ _ _ _ _ _ _ _ _ _ _ _ _ _ _ _ _ _ _ _ _ _ _ _ _ _ _ _ _ _ _ _ _ _ _ _ _ _ _ w3602 w3623 w3644 w3665 w3689 _ _ _ _ _ _ _]
            tunnel: w1644 -> [_ _ _ _ _ _ _ _ _ _ _ _ _ _ _ _ _ _ _ _ _ _ _ _ _ _ _ _ _ _ _ _ _ _ _ _ _ _ _ _ _ _ _ _ _ _ _ _ _ _ _ _ _ _ _ _ _ _ _ _ _ _ _ _ _ _ _ w3761 _ _ _ _]
            tunnel: [w1719 w1738 w1757 w1786 w1858 w1940 w2011 w2062 w2131 w2190 w2254 w2285 w2339 w2377 w2447 w2465 w2487 w2516 w2562 w2597 w2625 w2650 w2673 w2702 w2727 w2744 w2771 w2787 w2813 w2834 w2853 w2872 w2891 w2919 w2947 w2975 w2999 w3020 w3039 w3058 w3077 w3110 w3140 w3157 w3191 w3213 w3255 w3276 w3303 w3327 w3350 w3377 w3401 w3420 w3442 w3488 w3501 w3538 w3559 w3583 w3601 w3622 w3643 w3664 w3686 w3706 w3735 w3755 w3782 w3803 w3842 w3875] -> w1638
            tunnel: w1639 -> [w1719 w1738 w1757 w1786 w1858 w1940 w2011 w2062 w2131 w2190 w2254 w2285 w2339 w2377 w2447 _ _ w2516 w2562 w2597 w2625 w2650 w2673 w2702 w2727 w2744 w2771 w2787 w2813 w2834 w2853 w2872 w2891 w2919 w2947 w2975 w2999 w3020 w3039 w3058 w3077 w3110 w3140 w3157 w3191 w3213 w3255 w3276 w3303 w3327 w3350 w3377 w3401 w3420 w3442 w3488 w3502 w3538 w3559 w3583 w3601 w3622 w3643 w3664 w3686 w3706 w3735 w3755 w3782 w3803 w3842 w3875]
            tunnel: w1637 -> [w1718 w1737 w1756 w1785 w1857 w1939 w2010 w2061 w2130 w2189 w2253 w2284 w2338 w2376 w2446 w2473 w2486 w2515 w2554 w2596 w2624 w2649 w2672 w2701 w2726 w2743 w2770 w2786 w2812 w2833 w2852 w2871 w2890 w2918 w2946 w2974 w2998 w3019 w3038 w3057 w3076 w3109 w3139 w3156 w3190 w3227 w3254 w3275 w3302 w3326 w3349 w3376 w3400 w3419 w3441 w3487 w3513 w3537 w3558 w3586 w3600 w3621 w3642 w3663 w3685 w3705 w3734 w3754 w3781 w3802 w3841 w3874]
            tunnel: w1636 -> [w1717 w1736 w1755 w1784 w1856 w1938 w2009 w2060 w2129 w2188 w2252 w2283 w2337 w2375 w2445 w2472 w2485 w2514 w2553 w2595 w2623 w2648 w2671 w2700 w2725 w2742 w2769 w2785 w2811 w2832 w2851 w2870 w2889 w2917 w2945 w2973 w2997 w3018 w3037 w3056 w3075 w3108 w3138 w3155 w3189 w3224 w3253 w3274 w3301 w3325 w3348 w3375 w3399 w3418 w3440 w3486 w3512 w3536 w3557 w3585 w3599 w3620 w3641 w3662 w3684 w3704 w3733 w3753 w3780 w3801 w3840 w3873]
            tunnel: [w1718 w1737 w1756 w1785 w1857 w1939 w2010 w2061 w2130 w2189 w2253 w2284 w2338 w2376 w2446 w2473 w2486 w2515 w2554 w2596 w2624 w2649 w2672 w2701 w2726 w2743 w2770 w2786 w2812 w2833 w2852 w2871 w2890 w2918 w2946 w2974 w2998 w3019 w3038 w3057 w3076 w3109 w3139 w3156 w3190 w3226 w3254 w3275 w3302 w3326 w3349 w3376 w3400 w3419 w3441 w3487 w3513 w3537 w3558 w3586 w3600 w3621 w3642 w3663 w3685 w3705 w3734 w3754 w3781 w3802 w3841 w3874] -> w1635
            tunnel: [w1717 w1736 w1755 w1784 w1856 w1938 w2009 w2060 w2129 w2188 w2252 w2283 w2337 w2375 w2445 w2472 w2485 w2514 w2553 w2595 w2623 w2648 w2671 w2700 w2725 w2742 w2769 w2785 w2811 w2832 w2851 w2870 w2889 w2917 w2945 w2973 w2997 w3018 w3037 w3056 w3075 w3108 w3138 w3155 w3189 w3225 w3253 w3274 w3301 w3325 w3348 w3375 w3399 w3418 w3440 w3486 w3512 w3536 w3557 w3585 w3599 w3620 w3641 w3662 w3684 w3704 w3733 w3753 w3780 w3801 w3840 w3873] -> w1634
            tunnel: w1633 -> [w1716 _ _ _ _ _ _ _ _ _ _ _ _ _ w2438 _ _ w2511 w2565 w2587 _ _ _ _ _ _ _ _ _ _ _ _ _ _ w2942 _ _ _ _ _ _ w3106 w3137 _ _ _ _ _ _ _ w3347 _ _ _ _ w3467 _ _ _ _ _ _ _ _ _ _ _ _ _ _ _ _]
            tunnel: w1632 -> [w1715 _ _ _ _ _ _ _ _ _ _ _ _ _ w2439 _ _ w2510 w2564 w2586 _ _ _ _ _ _ _ _ _ _ _ _ _ _ w2941 _ _ _ _ _ _ w3107 w3136 _ _ _ _ _ _ _ w3346 _ _ _ _ w3466 _ _ _ _ _ _ _ _ _ _ _ _ _ _ _ _]
            tunnel: [_ _ _ _ _ _ _ _ _ _ _ _ _ _ _ _ _ _ _ _ _ _ _ _ _ _ w2761 _ _ _ _ _ _ _ w2935 _ _ _ _ _ _ w3099 w3128 _ _ _ _ _ _ _ _ _ _ _ _ _ _ _ _ _ _ _ _ _ _ _ _ _ _ _ _ _] -> w1587
            tunnel: [_ _ _ _ _ _ _ _ _ _ _ _ _ _ _ _ _ _ _ _ _ _ _ _ _ _ w2760 _ _ _ _ _ _ _ w2934 _ _ _ _ _ _ w3098 w3127 _ _ _ _ _ _ _ _ _ _ _ _ _ _ _ _ _ _ _ _ _ _ _ _ _ _ _ _ _] -> w1586
            tunnel: [_ _ _ _ _ _ _ _ _ _ _ _ _ _ _ _ _ _ _ _ _ _ _ w2696 w2715 _ _ _ _ _ _ _ _ _ _ _ _ _ _ _ _ _ _ _ _ _ _ _ _ _ _ _ _ _ _ _ _ _ _ _ _ _ _ _ _ _ _ _ _ _ _ _] -> w1630
            tunnel: [_ _ _ _ _ _ _ _ _ _ _ _ _ _ _ _ _ _ _ _ _ _ _ _ TRUE ("Recording") _ _ _ _ _ _ _ _ _ _ _ _ _ _ _ _ _ _ _ _ _ _ _ _ _ _ _ _ _ _ _ _ _ _ _ _ _ _ _ _ _ _ _ _ _ _ _] -> w1627
            tunnel: [_ _ _ _ _ _ _ _ _ _ _ _ _ _ _ _ _ _ _ _ _ _ _ w2696 _ _ _ _ _ _ _ _ _ _ _ _ _ _ _ _ _ _ _ _ _ _ _ _ _ _ _ _ _ _ _ _ _ _ _ _ _ _ _ _ _ _ _ _ _ _ _ _] -> w1623
            tunnel: [_ _ _ _ _ _ _ _ _ _ _ _ _ _ _ TRUE _ _ _ _ _ _ _ _ _ _ _ _ _ _ _ _ _ _ _ _ _ _ _ _ _ _ _ _ _ _ _ _ _ _ _ _ _ _ _ _ _ _ _ _ _ _ _ _ _ _ _ _ _ _ _ _] -> w1620
            tunnel: [_ _ _ _ _ _ _ _ _ _ _ _ _ _ _ _ _ TRUE _ _ _ _ _ _ _ _ _ _ _ _ _ _ _ _ _ _ _ _ _ _ _ _ _ _ _ _ _ _ _ _ _ _ _ _ _ _ _ _ _ _ _ _ _ _ _ _ _ _ _ _ _ _] -> w1618
            tunnel: [_ _ _ _ _ _ _ _ _ _ _ _ _ _ _ _ _ w2506 _ _ _ _ _ _ _ _ _ _ _ _ _ _ _ _ _ _ _ _ _ _ _ _ _ _ _ _ _ _ _ _ _ _ _ _ _ _ _ _ _ _ _ _ _ _ _ _ _ _ _ _ _ _] -> w1617
            tunnel: w1604 -> [_ _ _ _ _ _ _ _ _ _ _ _ _ _ _ _ _ _ _ _ _ _ _ _ _ _ _ _ _ _ _ _ _ _ _ _ _ _ _ _ _ _ _ _ _ _ _ _ _ _ _ _ _ _ _ _ _ _ _ _ _ _ _ _ _ _ _ _ _ _ w3838 w3871]
            tunnel: [_ _ _ _ _ _ _ _ _ _ _ _ _ _ _ _ _ _ _ _ _ _ _ _ _ _ _ _ _ _ _ _ _ _ _ _ _ _ _ _ _ _ _ _ _ _ _ _ _ _ _ _ _ _ _ _ _ _ _ _ _ _ _ _ _ _ _ _ _ _ w3836 w3869] -> w1603
            tunnel: w1599 -> [_ _ _ _ _ _ _ _ _ _ _ _ _ _ _ _ _ _ _ _ w2609 w2639 w2661 w2692 w2713 w2737 w2762 w2784 w2810 _ _ _ _ w2908 w2936 w2972 w2996 _ _ _ _ w3100 w3129 _ _ _ _ _ _ _ _ _ _ _ _ _ _ _ _ _ _ _ _ _ _ _ _ _ _ _ _ _]
            tunnel: [_ _ _ _ _ _ _ _ _ _ _ _ _ _ _ _ _ _ _ w2575 w2609 w2638 w2660 w2691 w2712 w2737 w2762 w2784 w2810 _ _ _ _ w2908 w2936 w2972 w2996 _ _ _ _ w3100 w3129 _ _ _ _ _ _ _ _ _ _ _ _ _ _ _ _ _ _ _ _ _ _ _ _ _ _ _ _ _] -> w1598
            tunnel: [_ _ _ _ _ _ _ _ _ _ _ _ _ _ _ _ _ _ _ _ _ _ _ _ _ _ w2759 _ _ _ _ _ _ _ w2933 _ _ _ _ _ _ w3097 w3126 _ _ _ _ _ _ _ _ _ _ _ _ _ _ _ _ _ _ _ _ _ _ _ _ _ _ _ _ _] -> w1591
            tunnel: [_ _ _ _ _ _ _ _ _ _ _ _ _ _ _ _ _ _ _ _ _ _ _ _ _ _ w2758 _ _ _ _ _ _ _ w2932 _ _ _ _ _ _ w3096 w3125 _ _ _ _ _ _ _ _ _ _ _ _ _ _ _ _ _ _ _ _ _ _ _ _ _ _ _ _ _] -> w1589
            tunnel: [_ _ _ _ _ _ _ _ _ _ _ _ _ _ _ _ _ _ _ _ _ _ _ _ _ _ _ _ _ _ _ _ _ _ w2931 _ _ _ _ _ _ _ _ _ _ _ _ _ _ _ _ _ _ _ _ _ _ _ _ _ _ _ _ _ _ _ _ _ _ _ _ _] -> w1595
            tunnel: [_ _ _ _ _ _ _ _ _ _ _ _ _ _ _ w2460 _ _ _ _ _ _ _ _ _ _ _ _ _ _ _ _ _ _ _ _ _ _ _ _ _ _ _ _ _ _ _ _ _ _ _ _ _ _ _ _ _ _ _ _ _ _ _ _ _ _ _ _ _ _ _ _] -> w1578
            frame "Start1", Default {
              w1714 = FALSE ("SelectionState")
              n992 = xnode "Read/Write Control"("FPGA VI Reference In"=w1716, "error in"=w1715, "SelectionState"=w1714, "LR_reward_Laser_l1"=w1714, "LR_wrong_Laser_l1"=w1714, "LR_reward_Event_l1"=w1714, "LR_wrong_Event_l1"=w1714, "Left(F)_or_Right(T)"=w1714, "ignoreWrong"=w1714, "SelectionState"=w1714, "LR_reward_Laser_l2"=w1714, "LR_wrong_laser_l2"=w1714, "LR_reward_Event_l2"=w1714, "LR_wrong_Event_l2"=w1714, "LC_Event_l1"=w1714, "LC_Laser_l1"=w1714, "LC_Laser_l2"=w1714, "LC_Event_l2"=w1714, "CueLed_Event"=w1714) -> ()  [unwired: 2 out]
            }
            frame "Start2" {
            }
            frame "Start3" {
            }
            frame "saveSettings1" {
              n993 = call "myRIO_BRig_RT_dataExp_Audio_freq__L.vi"() -> ("output_Audio_freq__L"=w1809:i32)  [unwired: 11 in]
              n994 = call "myRIO_BRig_RT_dataExp_Audio_freq__R.vi"() -> ("output_Audio_freq__R"=w1808:i32)  [unwired: 11 in]
              n995 = call "myRIO_BRig_RT_dataExp_Audio_amp__L.vi"() -> ("output_Audio_amp__L"=w1807:i32)  [unwired: 11 in]
              n996 = call "myRIO_BRig_RT_dataExp_Audio_amp__R.vi"() -> ("output_Audio_amp__R"=w1805:i32)  [unwired: 11 in]
              n997 = call "myRIO_BRig_RT_dataExp_TPB_min__L.vi"() -> ("output_TPB_min__L"=w1817:i32)  [unwired: 11 in]
              n998 = call "myRIO_BRig_RT_dataExp_TPB_min__R.vi"() -> ("output_TPB_min__R"=w1815:i32)  [unwired: 11 in]
              n999 = call "myRIO_BRig_RT_dataExp_TPB_max__L.vi"() -> ("output_TPB_max__L"=w1813:i32)  [unwired: 11 in]
              n1000 = call "myRIO_BRig_RT_dataExp_TPB_max__R.vi"() -> ("output_TPB_max__R"=w1811:i32)  [unwired: 11 in]
              n1001 = call "myRIO_BRig_RT_dataExp_Cue1Param_AudioLed_Count_Switch.vi"() -> ("output_Cue1Param_AudioLed_Count_Switch"=w1779:i32)  [unwired: 11 in]
              n1002 = call "myRIO_BRig_RT_dataExp_Cue1Param_AudioLed_Probability_Switch.vi"() -> ("output_Cue1Param_AudioLed_Probability_Switch"=w1777:i32)  [unwired: 11 in]
              n1003 = call "myRIO_BRig_RT_dataExp_Cue1Param_CueType_Switch.vi"() -> ("output_Cue1Param_CueType_Switch"=w1775:i32)  [unwired: 11 in]
              n1004 = call "myRIO_BRig_RT_dataExp_ItrialUntilReward.vi"() -> ("output_I_trialUntilReward"=w1830:i32)  [unwired: 11 in]
              n1005 = call "myRIO_BRig_RT_dataExp_IblockUntilReward.vi"() -> ("output_I_blockUntilReward"=w1826:i32)  [unwired: 11 in]
              n1006 = call "myRIO_BRig_RT_dataExp_CueCycles.vi"() -> ("output_CueCycles"=w1825:i32)  [unwired: 11 in]
              n1007 = call "myRIO_BRig_RT_dataExp_ENL_min.vi"() -> ("output_ENL_min"=w1823:i32)  [unwired: 11 in]
              n1008 = call "myRIO_BRig_RT_dataExp_ENL_max.vi"() -> ("output_ENL_max"=w1821:i32)  [unwired: 11 in]
              n1009 = call "myRIO_BRig_RT_dataExp_ENL_penalty.vi"() -> ("output_ENL_penalty"=w1819:i32)  [unwired: 11 in]
              n1010 = local read "Audio_Freq__L"() -> (w1783:u8)
              n1011 = local read "Audio_Freq__R"() -> (w1781:u8)
              n1012 = local read "Audio_Amp__L"() -> (w1806:u16)
              n1013 = local read "TpB_Min_L"() -> (w1816:u16)
              n1014 = local read "TpB_Min_R"() -> (w1814:u16)
              n1015 = local read "TpB_Max_L"() -> (w1812:u16)
              n1016 = local read "TpB_Max_R"() -> (w1810:u16)
              n1017 = local read "Audio_Amp__R"() -> (w1804:u16)
              n1018 = local read "TrialUntilReward"() -> (w1829:bool)
              n1019 = local read "CueCycles"() -> (w1824:u16)
              n1020 = local read "Tcycle_ENL_min"() -> (w1822:u16)
              n1021 = local read "Tcycle_ENL_max"() -> (w1820:u16)
              n1022 = local read "Tcycle_ENLPenalty"() -> (w1818:u16)
              n1023 = local read "Cue1Param_AudioLed_Count_Switch"() -> (w1778:u16)
              n1024 = local read "Cue1Param_AudioLed_Probability_Switch"() -> (w1776:u16)
              n1025 = local read "Cue1Param_CueType_Switch"() -> (w1774:u16)
              n1026 = To Unsigned Word Integer(number=w1781) -> (unsigned 16bit integer=w1780:u16)
              n1027 = To Unsigned Word Integer(number=w1783) -> (unsigned 16bit integer=w1782:u16)
              n1028 = Boolean To (0,1)(Boolean=w1829) -> (0, 1=w1828:i16)
              n1029 = To Unsigned Word Integer(number=w1828) -> (unsigned 16bit integer=w1827:u16)
              n1030 = local read "BUR_min"() -> (w1798:u16)
              n1031 = local read "BUR_max"() -> (w1799:u16)
              n1032 = Not Equal To 0?(x=w1798) -> (x != 0?=w1797:bool)
              n1033 = Not Equal To 0?(x=w1799) -> (x != 0?=w1796:bool)
              n1034 = And(x=w1797, y=w1796) -> (x .and. y?=w1795:bool)
              n1035 = Boolean To (0,1)(Boolean=w1795) -> (0, 1=w1800:i16)
              n1036 = To Unsigned Word Integer(number=w1800) -> (unsigned 16bit integer=w1794:u16)
              n1037 = Replace Array Subset(array=w1832, new element #1=w1827, index #1=w1830, new element #2=w1794, index #2=w1826, new element #3=w1824, index #3=w1825, new element #4=w1822, index #4=w1823, new element #5=w1820, index #5=w1821, new element #6=w1818, index #6=w1819, new element #7=w1816, index #7=w1817, new element #8=w1814, index #8=w1815, new element #9=w1812, index #9=w1813, new element #10=w1810, index #10=w1811, new element #11=w1782, index #11=w1809, new element #12=w1780, index #12=w1808, new element #13=w1806, index #13=w1807, new element #14=w1804, index #14=w1805, new element #15=w1778, index #15=w1779, new element #16=w1776, index #16=w1777, new element #17=w1774, index #17=w1775) -> (w1831:u16[])
            }
            frame "saveSettings2" {
              n1038 = call "myRIO_BRig_RT_dataExp_Tcycle_Cue1_Audio_min.vi"() -> ("output_Tcycle_Cue1_Audio_min"=w1875:i32)  [unwired: 11 in]
              n1039 = call "myRIO_BRig_RT_dataExp_Tcycle_Cue1_Audio_max.vi"() -> ("output_Tcycle_Cue1_Audio_max"=w1874:i32)  [unwired: 11 in]
              n1040 = call "myRIO_BRig_RT_dataExp_Tcycle_Cue1Penalty_Audio.vi"() -> ("output_Tcycle_Cue1Penalty_Audio"=w1873:i32)  [unwired: 11 in]
              n1041 = call "myRIO_BRig_RT_dataExp_Tcycle_RewardPost.vi"() -> ("output_Tcycle_RewardPost"=w1881:i32)  [unwired: 11 in]
              n1042 = call "myRIO_BRig_RT_dataExp_Tcycle_Wrong.vi"() -> ("output_Tcycle_Wrong"=w1879:i32)  [unwired: 11 in]
              n1043 = call "myRIO_BRig_RT_dataExp_Tcycle_Timeout.vi"() -> ("output_Tcycle_Timeout"=w1877:i32)  [unwired: 11 in]
              n1044 = call "myRIO_BRig_RT_dataExp_SolenoidProbability_L.vi"() -> ("output_SolenoidProbability_L"=w1853:i32)  [unwired: 11 in]
              n1045 = call "myRIO_BRig_RT_dataExp_SolenoidProbability_R.vi"() -> ("output_SolenoidProbability_R"=w1852:i32)  [unwired: 11 in]
              n1046 = call "myRIO_BRig_RT_dataExp_Cue1Param_AudioLed_Count_NS.vi"() -> ("output_Cue1Param_AudioLed_Count_NS"=w1849:i32)  [unwired: 11 in]
              n1047 = call "myRIO_BRig_RT_dataExp_Cue1Param_AudioLed_Probability_NS.vi"() -> ("output_Cue1Param_AudioLed_Probability_NS"=w1847:i32)  [unwired: 11 in]
              n1048 = call "myRIO_BRig_RT_dataExp_Cue1Param_CueType_NS.vi"() -> ("output_Cue1Param_CueType_NS"=w1845:i32)  [unwired: 11 in]
              n1049 = call "myRIO_BRig_RT_dataExp_nBlock.vi"() -> ("output_nBlock"=w1890:i32)  [unwired: 11 in]
              n1050 = call "myRIO_BRig_RT_dataExp_nTrial.vi"() -> ("output_nTrial"=w1889:i32)  [unwired: 11 in]
              n1051 = call "myRIO_BRig_RT_dataExp_runTime_seconds.vi"() -> ("output_RunTime_minutes"=w1888:i32)  [unwired: 11 in]
              n1052 = call "myRIO_BRig_RT_dataExp_Tcycle_Selection.vi"() -> ("output_Tcycle_Selection"=w1887:i32)  [unwired: 11 in]
              n1053 = call "myRIO_BRig_RT_dataExp_Tcycle_Reward__L.vi"() -> ("output_Tcycle_Reward__L"=w1885:i32)  [unwired: 11 in]
              n1054 = call "myRIO_BRig_RT_dataExp_Tcycle_Reward__R.vi"() -> ("output_Tcycle_Reward__R"=w1883:i32)  [unwired: 11 in]
              n1055 = local read "Tcycle_CuePenalty_Audio"() -> (w1866:u16)
              n1056 = call "myRIO_BRig_RT_dataExp_Tcycle_Cue1_LED_min.vi"() -> ("output_Tcycle_Cue1_LED_min"=w1843:i32)  [unwired: 11 in]
              n1057 = call "myRIO_BRig_RT_dataExp_Tcycle_Cue1_LED_max.vi"() -> ("output_Tcycle_Cue1_LED_max"=w1842:i32)  [unwired: 11 in]
              n1058 = call "myRIO_BRig_RT_dataExp_Tcycle_Cue1Penalty_LED.vi"() -> ("output_Tcycle_Cue1Penalty_LED"=w1841:i32)  [unwired: 11 in]
              n1059 = local read "Tcycle_Cue_Audio_max"() -> (w1854:u16)
              n1060 = local read "Tcycle_Cue_Audio_min"() -> (w1855:u16)
              n1061 = local read "Tcycle_RewardPost"() -> (w1880:u16)
              n1062 = local read "Tcycle_Wrong"() -> (w1878:u16)
              n1063 = local read "Tcycle_Timeout"() -> (w1876:u16)
              n1064 = local read "Tcycle_Selection"() -> (w1886:u16)
              n1065 = local read "Tcycle_Reward_L"() -> (w1884:u16)
              n1066 = local read "Tcycle_Reward_R"() -> (w1882:u16)
              n1067 = local read "Cue1Param_AudioLed_Count_NS"() -> (w1848:u16)
              n1068 = local read "Cue1Param_AudioLed_Probability_NS"() -> (w1846:u16)
              n1069 = local read "Cue1Param_CueType_NS"() -> (w1844:u16)
              n1070 = local read "SolenoidProbability_R"() -> (w1850:u16)
              n1071 = local read "SolenoidProbability_L"() -> (w1851:u16)
              n1072 = local read "Tcycle_CuePenalty_LED"() -> (w1838:u16)
              n1073 = local read "Tcycle_Cue_LED_min"() -> (w1840:u16)
              n1074 = local read "Tcycle_Cue_LED_max"() -> (w1839:u16)
              n1075 = Replace Array Subset(array=w1892, new element #1=u16 0, index #1=w1890, new element #2=u16 0, index #2=w1889, new element #3=u16 0, index #3=w1888, new element #4=w1886, index #4=w1887, new element #5=w1884, index #5=w1885, new element #6=w1882, index #6=w1883, new element #7=w1880, index #7=w1881, new element #8=w1878, index #8=w1879, new element #9=w1876, index #9=w1877, new element #10=w1855, index #10=w1875, new element #11=w1854, index #11=w1874, new element #12=w1866, index #12=w1873, new element #13=w1851, index #13=w1853, new element #14=w1850, index #14=w1852, new element #15=w1848, index #15=w1849, new element #16=w1846, index #16=w1847, new element #17=w1844, index #17=w1845, new element #18=w1840, index #18=w1843, new element #19=w1839, index #19=w1842, new element #20=w1838, index #20=w1841) -> (w1891:u16[])
            }
            frame "saveSettings3" {
              w1904 = 100.0 ("y")
              n1076 = call "myRIO_BRig_RT_dataExp_laser1_Freq.vi"() -> ("output_laser1_Freq"=w1937:i32)  [unwired: 11 in]
              n1077 = call "myRIO_BRig_RT_dataExp_laser1_Tpeak.vi"() -> ("output_laser1_Tpeak"=w1932:i32)  [unwired: 11 in]
              n1078 = call "myRIO_BRig_RT_dataExp_laser1_Tshutter.vi"() -> ("output_laser1_Tshutter"=w1927:i32)  [unwired: 11 in]
              n1079 = call "myRIO_BRig_RT_dataExp_FPGA_f_count2ms.vi"() -> ("output_FPGA_f_count2ms"=w1922:i32)  [unwired: 11 in]
              n1080 = call "myRIO_BRig_RT_dataExp_laser1_Power_min.vi"() -> ("output_laser1_Power_min"=w1917:i32)  [unwired: 11 in]
              n1081 = call "myRIO_BRig_RT_dataExp_laser1_Power_max.vi"() -> ("output_laser1_Power_max"=w1910:i32)  [unwired: 11 in]
              n1082 = call "myRIO_BRig_RT_dataExp_laser1_Power_step.vi"() -> ("output_laser1_Power_step"=w1909:i32)  [unwired: 11 in]
              n1083 = call "myRIO_BRig_RT_dataExp_laser1_duration.vi"() -> ("output_laser1_duration"=w1912:i32)  [unwired: 11 in]
              n1084 = local read "Laser_Tshutter_l1"() -> (w1924:dbl)
              n1085 = local read "Laser_Tpeak_l1"() -> (w1929:dbl)
              n1086 = local read "Laser_power_max_l1"() -> (w1903:dbl)
              n1087 = local read "Laser_power_step_l1"() -> (w1902:dbl)
              n1088 = local read "Laser_power_min_l1"() -> (w1914:dbl)
              n1089 = local read "Laser_Freq_l1"() -> (w1936:dbl)
              n1090 = call "myRIO_BRig_RT_dataExp_BUR_min.vi"() -> ("output_BUR_min"=w1956:i32)  [unwired: 11 in]
              n1091 = call "myRIO_BRig_RT_dataExp_BUR_max.vi"() -> ("output_BUR_max"=w1954:i32)  [unwired: 11 in]
              n1092 = call "myRIO_BRig_RT_dataExp_Audio_sp__L.vi"() -> ("output_Audio_sp__L"=w1951:i32)  [unwired: 11 in]
              n1093 = call "myRIO_BRig_RT_dataExp_Audio_sp__R.vi"() -> ("output_Audio_sp__R"=w1950:i32)  [unwired: 11 in]
              n1094 = local read "FPGA_count2ms"() -> (w1919:dbl)
              n1095 = local read "sp_LeftSpout"() -> (w1949:u16)
              n1096 = local read "BUR_max"() -> (w1953:u16)
              n1097 = local read "sp_RightSpout"() -> (w1948:u16)
              n1098 = local read "BUR_min"() -> (w1955:u16)
              n1099 = Multiply(x=w1936, y=w1904) -> (x*y=w1935:dbl)
              n1100 = Multiply(x=w1929, y=w1904) -> (x*y=w1931:dbl)
              n1101 = Multiply(x=w1924, y=w1904) -> (x*y=w1926:dbl)
              n1102 = Multiply(x=w1919, y=w1904) -> (x*y=w1921:dbl)
              n1103 = Multiply(x=w1914, y=w1904) -> (x*y=w1916:dbl)
              n1104 = Multiply(x=w1903, y=w1904) -> (x*y=w1908:dbl)
              n1105 = Multiply(x=w1902, y=w1904) -> (x*y=w1906:dbl)
              n1106 = Round To Nearest(number=w1935) -> (nearest integer value=w1934:dbl)
              n1107 = Round To Nearest(number=w1931) -> (nearest integer value=w1930:dbl)
              n1108 = Round To Nearest(number=w1926) -> (nearest integer value=w1925:dbl)
              n1109 = Round To Nearest(number=w1921) -> (nearest integer value=w1920:dbl)
              n1110 = Round To Nearest(number=w1916) -> (nearest integer value=w1915:dbl)
              n1111 = Round To Nearest(number=w1908) -> (nearest integer value=w1907:dbl)
              n1112 = Round To Nearest(number=w1906) -> (nearest integer value=w1905:dbl)
              n1113 = To Unsigned Word Integer(number=w1934) -> (unsigned 16bit integer=w1933:u16)
              n1114 = To Unsigned Word Integer(number=w1930) -> (unsigned 16bit integer=w1928:u16)
              n1115 = To Unsigned Word Integer(number=w1925) -> (unsigned 16bit integer=w1923:u16)
              n1116 = To Unsigned Word Integer(number=w1920) -> (unsigned 16bit integer=w1918:u16)
              n1117 = To Unsigned Word Integer(number=w1915) -> (unsigned 16bit integer=w1913:u16)
              n1118 = To Unsigned Word Integer(number=w1907) -> (unsigned 16bit integer=w1901:u16)
              n1119 = To Unsigned Word Integer(number=w1905) -> (unsigned 16bit integer=w1900:u16)
              n1120 = local read "Laser_duration_l1"() -> (w1911:u16)
              n1121 = Replace Array Subset(array=w1957, new element #1=w1955, index #1=w1956, new element #2=w1953, index #2=w1954, new element #3=w1949, index #3=w1951, new element #4=w1948, index #4=w1950, new element #5=w1933, index #5=w1937, new element #6=w1928, index #6=w1932, new element #7=w1923, index #7=w1927, new element #8=w1918, index #8=w1922, new element #9=w1913, index #9=w1917, new element #10=w1901, index #10=w1910, new element #11=w1900, index #11=w1909, new element #12=w1911, index #12=w1912) -> (w1952:u16[])
            }
            frame "saveSettings4" {
              w1977 = 100.0 ("y")
              n1122 = call "myRIO_BRig_RT_dataExp_laser2_Freq.vi"() -> ("output_laser2_Freq"=w1966:i32)  [unwired: 11 in]
              n1123 = call "myRIO_BRig_RT_dataExp_laser2_Tpeak.vi"() -> ("output_laser2_Tpeak"=w1968:i32)  [unwired: 11 in]
              n1124 = call "myRIO_BRig_RT_dataExp_laser2_Tshutter.vi"() -> ("output_laser2_Tshutter"=w1970:i32)  [unwired: 11 in]
              n1125 = call "myRIO_BRig_RT_dataExp_laser2_Power_min.vi"() -> ("output_laser2_Power_min"=w1985:i32)  [unwired: 11 in]
              n1126 = call "myRIO_BRig_RT_dataExp_laser2_Power_max.vi"() -> ("output_laser2_Power_max"=w1984:i32)  [unwired: 11 in]
              n1127 = call "myRIO_BRig_RT_dataExp_laser2_Power_step.vi"() -> ("output_laser2_Power_step"=w1983:i32)  [unwired: 11 in]
              n1128 = call "myRIO_BRig_RT_dataExp_laser2_duration.vi"() -> ("output_laser2_duration"=w1982:i32)  [unwired: 11 in]
              n1129 = call "myRIO_BRig_RT_dataExp_CueLed_Freq.vi"() -> ("output_CueLed_Freq"=w1974:i32)  [unwired: 11 in]
              n1130 = call "myRIO_BRig_RT_dataExp_CueLed_Tpeak.vi"() -> ("output_CueLed_Tpeak"=w1973:i32)  [unwired: 11 in]
              n1131 = local read "Laser_Tshutter_l2"() -> (w2000:dbl)
              n1132 = local read "Laser_Tpeak_l2"() -> (w2003:dbl)
              n1133 = local read "Laser_power_max_l2"() -> (w1990:dbl)
              n1134 = local read "Laser_power_step_l2"() -> (w1989:dbl)
              n1135 = local read "Laser_power_min_l2"() -> (w1997:dbl)
              n1136 = local read "Laser_Freq_l2"() -> (w2008:dbl)
              n1137 = local read "CueLed_Tpeak"() -> (w1975:dbl)
              n1138 = local read "CueLed_Freq"() -> (w1976:dbl)
              n1139 = Multiply(x=w2008, y=w1977) -> (x*y=w2007:dbl)
              n1140 = Multiply(x=w2003, y=w1977) -> (x*y=w2005:dbl)
              n1141 = Multiply(x=w2000, y=w1977) -> (x*y=w2002:dbl)
              n1142 = Multiply(x=w1997, y=w1977) -> (x*y=w1999:dbl)
              n1143 = Multiply(x=w1990, y=w1977) -> (x*y=w1994:dbl)
              n1144 = Multiply(x=w1989, y=w1977) -> (x*y=w1992:dbl)
              n1145 = Multiply(x=w1976, y=w1977) -> (x*y=w1978:dbl)
              n1146 = Multiply(x=w1975, y=w1977) -> (x*y=w1979:dbl)
              n1147 = Round To Nearest(number=w2007) -> (nearest integer value=w2006:dbl)
              n1148 = Round To Nearest(number=w2005) -> (nearest integer value=w2004:dbl)
              n1149 = Round To Nearest(number=w2002) -> (nearest integer value=w2001:dbl)
              n1150 = Round To Nearest(number=w1999) -> (nearest integer value=w1998:dbl)
              n1151 = Round To Nearest(number=w1994) -> (nearest integer value=w1993:dbl)
              n1152 = Round To Nearest(number=w1992) -> (nearest integer value=w1991:dbl)
              n1153 = Round To Nearest(number=w1978) -> (nearest integer value=w1981:dbl)
              n1154 = Round To Nearest(number=w1979) -> (nearest integer value=w1980:dbl)
              n1155 = To Unsigned Word Integer(number=w2006) -> (unsigned 16bit integer=w1965:u16)
              n1156 = To Unsigned Word Integer(number=w2004) -> (unsigned 16bit integer=w1967:u16)
              n1157 = To Unsigned Word Integer(number=w2001) -> (unsigned 16bit integer=w1969:u16)
              n1158 = To Unsigned Word Integer(number=w1998) -> (unsigned 16bit integer=w1996:u16)
              n1159 = To Unsigned Word Integer(number=w1993) -> (unsigned 16bit integer=w1988:u16)
              n1160 = To Unsigned Word Integer(number=w1991) -> (unsigned 16bit integer=w1987:u16)
              n1161 = To Unsigned Word Integer(number=w1981) -> (unsigned 16bit integer=w1972:u16)
              n1162 = To Unsigned Word Integer(number=w1980) -> (unsigned 16bit integer=w1971:u16)
              n1163 = local read "Laser_duration_l2"() -> (w1995:u16)
              n1164 = Replace Array Subset(array=w2020, new element #1=w1965, index #1=w1966, new element #2=w1967, index #2=w1968, new element #3=w1969, index #3=w1970, new element #4=w1996, index #4=w1985, new element #5=w1988, index #5=w1984, new element #6=w1987, index #6=w1983, new element #7=w1995, index #7=w1982, new element #8=w1972, index #8=w1974, new element #9=w1971, index #9=w1973) -> (w2019:u16[])
            }
            frame "saveSettings_LC_ENL_l1" {
              # "Selection First"
              # "Count"
              # "Tdelay"
              # "Probability"
              # "OnOff"
              # "Block"
              # "delayOpt"
              # "Count"
              # "Tdelay"
              # "Probability"
              # "OnOff"
              # "Block"
              # "ENL1 All"
              # "delayOpt"
              # "Count"
              # "Tdelay"
              # "Probability"
              # "OnOff"
              # "Block"
              # "ENL1 First"
              n1165 = local read "LC_ENL1_delayOpt_Switch_l1"() -> (w2058:bool)
              n1166 = call "myRIO_BRig_RT_dataLC_ENL1_Block_NS_l1.vi"() -> ("output_ENL1_All_Block"=w2055:i32)  [unwired: 11 in]
              n1167 = call "myRIO_BRig_RT_dataLC_ENL1_OnOff_NS_l1.vi"() -> ("output_ENL1_OnOff_NS_l1"=w2045:i32)  [unwired: 11 in]
              n1168 = call "myRIO_BRig_RT_dataLC_ENL1_Probability_NS_l1.vi"() -> ("output_ENL1_Probability_NS_l1"=w2044:i32)  [unwired: 11 in]
              n1169 = call "myRIO_BRig_RT_dataLC_ENL1_Tdelay_NS_l1.vi"() -> ("output_ENL1_Tdelay_NS_l1"=w2043:i32)  [unwired: 11 in]
              n1170 = call "myRIO_BRig_RT_dataLC_ENL1_Count_NS_l1.vi"() -> ("output_ENL1_Count_NS_l1"=w2042:i32)  [unwired: 11 in]
              n1171 = call "myRIO_BRig_RT_dataLC_ENL1_delayOpt_NS_l1.vi"() -> ("output_ENL1_delayOpt_NS_l1"=w2041:i32)  [unwired: 11 in]
              n1172 = call "myRIO_BRig_RT_dataLC_ENL1_Block_Switch_l1.vi"() -> ("output_ENL1_Block_Switch_l1"=w2081:i32)  [unwired: 11 in]
              n1173 = call "myRIO_BRig_RT_dataLC_ENL1_OnOff_Switch_l1.vi"() -> ("output_ENL1_OnOff_Switch_l1"=w2079:i32)  [unwired: 11 in]
              n1174 = call "myRIO_BRig_RT_dataLC_ENL1_Probability_Switch_l1.vi"() -> ("output_ENL1_Probability_Switch_l1"=w2075:i32)  [unwired: 11 in]
              n1175 = call "myRIO_BRig_RT_dataLC_ENL1_Tdelay_Switch_l1.vi"() -> ("output_ENL1_Tdelay_Switch_l1"=w2073:i32)  [unwired: 11 in]
              n1176 = call "myRIO_BRig_RT_dataLC_ENL1_Count_Switch_l1.vi"() -> ("output_ENL1_Count_Switch_l1"=w2071:i32)  [unwired: 11 in]
              n1177 = call "myRIO_BRig_RT_dataLC_ENL1_delayOpt_Switch_l1.vi"() -> ("output_ENL1_delayOpt_Switch_l1"=w2057:i32)  [unwired: 11 in]
              n1178 = local read "LC_ENL1_Count_Switch_l1"() -> (w2070:u16)
              n1179 = local read "LC_ENL1_Probability_Switch_l1"() -> (w2074:u16)
              n1180 = local read "LC_ENL1_Block_Switch_l1"() -> (w2080:u16)
              n1181 = local read "LC_ENL1_Tdelay_Switch_l1"() -> (w2072:u16)
              n1182 = local read "LC_ENL1_OnOff_Switch_l1"() -> (w2078:bool)
              n1183 = call "myRIO_BRig_RT_dataLC_Selection_Block_Switch_l1.vi"() -> ("output_Selection_Block_Switch_l1"=w2039:i32)  [unwired: 11 in]
              n1184 = call "myRIO_BRig_RT_dataLC_Selection_OnOff_Switch_l1.vi"() -> ("output_Selection_OnOff_Switch_l1"=w2038:i32)  [unwired: 11 in]
              n1185 = call "myRIO_BRig_RT_dataLC_Selection_Probability_Switch_l1.vi"() -> ("output_Selection_Probability_Switch_l1"=w2037:i32)  [unwired: 11 in]
              n1186 = call "myRIO_BRig_RT_dataLC_Selection_Tdelay_Switch_l1.vi"() -> ("output_Selection_Tdelay_Switch_l1"=w2036:i32)  [unwired: 11 in]
              n1187 = call "myRIO_BRig_RT_dataLC_Selection_Count_Switch_l1.vi"() -> ("output_Selection_Count_Switch_l1"=w2035:i32)  [unwired: 11 in]
              n1188 = local read "LC_ENL1_OnOff_NS_l1"() -> (w2051:bool)
              n1189 = local read "LC_ENL1_Probability_NS_l1"() -> (w2049:u16)
              n1190 = local read "LC_ENL1_delayOpt_NS_l1"() -> (w2047:bool)
              n1191 = local read "LC_Sel_Probability_Switch_l1"() -> (w2030:u16)
              n1192 = local read "LC_ENL1_Tdelay_NS_l1"() -> (w2040:u16)
              n1193 = local read "LC_ENL1_Block_NS_l1"() -> (w2052:u16)
              n1194 = local read "LC_ENL1_Count_NS_l1"() -> (w2048:u16)
              n1195 = local read "LC_Sel_Tdelay_Switch_l1"() -> (w2029:u16)
              n1196 = local read "LC_Sel_OnOff_Switch_l1"() -> (w2033:bool)
              n1197 = local read "LC_Sel_Count_Switch_l1"() -> (w2028:u16)
              n1198 = local read "LC_Sel_Block_Switch_l1"() -> (w2032:u16)
              n1199 = Boolean To (0,1)(Boolean=w2058) -> (0, 1=w2059:i16)
              n1200 = Boolean To (0,1)(Boolean=w2078) -> (0, 1=w2077:i16)
              n1201 = Boolean To (0,1)(Boolean=w2051) -> (0, 1=w2054:i16)
              n1202 = To Unsigned Word Integer(number=w2059) -> (unsigned 16bit integer=w2056:u16)
              n1203 = To Unsigned Word Integer(number=w2077) -> (unsigned 16bit integer=w2076:u16)
              n1204 = Boolean To (0,1)(Boolean=w2047) -> (0, 1=w2053:i16)
              n1205 = To Unsigned Word Integer(number=w2054) -> (unsigned 16bit integer=w2050:u16)
              n1206 = Boolean To (0,1)(Boolean=w2033) -> (0, 1=w2034:i16)
              n1207 = To Unsigned Word Integer(number=w2053) -> (unsigned 16bit integer=w2046:u16)
              n1208 = To Unsigned Word Integer(number=w2034) -> (unsigned 16bit integer=w2031:u16)
              n1209 = Replace Array Subset(array=w2082, new element #1=w2080, index #1=w2081, new element #2=w2076, index #2=w2079, new element #3=w2074, index #3=w2075, new element #4=w2072, index #4=w2073, new element #5=w2070, index #5=w2071, new element #6=w2056, index #6=w2057, new element #7=w2052, index #7=w2055, new element #8=w2050, index #8=w2045, new element #9=w2049, index #9=w2044, new element #10=w2040, index #10=w2043, new element #11=w2048, index #11=w2042, new element #12=w2046, index #12=w2041, new element #13=w2032, index #13=w2039, new element #14=w2031, index #14=w2038, new element #15=w2030, index #15=w2037, new element #16=w2029, index #16=w2036, new element #17=w2028, index #17=w2035) -> (w2083:u16[])
            }
            frame "saveSettings_LC_ENL_l2" {
              # "Selection First"
              # "Count"
              # "Tdelay"
              # "Probability"
              # "OnOff"
              # "Block"
              # "delayOpt"
              # "Count"
              # "Tdelay"
              # "Probability"
              # "OnOff"
              # "Block"
              # "ENL1 All"
              # "delayOpt"
              # "Count"
              # "Tdelay"
              # "Probability"
              # "OnOff"
              # "Block"
              # "ENL1 First"
              n1210 = call "myRIO_BRig_RT_dataLC_ENL1_Block_Switch_l2.vi"() -> ("output_ENL1_Block_Switch_l2"=w2102:i32)  [unwired: 11 in]
              n1211 = call "myRIO_BRig_RT_dataLC_ENL1_OnOff_Switch_l2.vi"() -> ("output_ENL1_OnOff_Switch_l2"=w2103:i32)  [unwired: 11 in]
              n1212 = call "myRIO_BRig_RT_dataLC_ENL1_Probability_Switch_l2.vi"() -> ("output_ENL1_Probability_Switch_l2"=w2104:i32)  [unwired: 11 in]
              n1213 = call "myRIO_BRig_RT_dataLC_ENL1_Tdelay_Switch_l2.vi"() -> ("output_ENL1_Tdelay_Switch_l2"=w2105:i32)  [unwired: 11 in]
              n1214 = call "myRIO_BRig_RT_dataLC_ENL1_Count_Switch_l2.vi"() -> ("output_ENL1_Count_Switch_l2"=w2106:i32)  [unwired: 11 in]
              n1215 = call "myRIO_BRig_RT_dataLC_ENL1_delayOpt_Switch_l2.vi"() -> ("output_ENL1_delayOpt_Switch_l2"=w2107:i32)  [unwired: 11 in]
              n1216 = local read "LC_ENL1_delayOpt_Switch_l2"() -> (w2127:bool)
              n1217 = call "myRIO_BRig_RT_dataLC_ENL1_Block_NS_l2.vi"() -> ("output_ENL1_Block_NS_l2"=w2096:i32)  [unwired: 11 in]
              n1218 = call "myRIO_BRig_RT_dataLC_ENL1_OnOff_NS_l2.vi"() -> ("output_ENL1_OnOff_NS_l2"=w2097:i32)  [unwired: 11 in]
              n1219 = call "myRIO_BRig_RT_dataLC_ENL1_Probability_NS_l2.vi"() -> ("output_ENL1_Probability_NS_l2"=w2098:i32)  [unwired: 11 in]
              n1220 = call "myRIO_BRig_RT_dataLC_ENL1_Tdelay_NS_l2.vi"() -> ("output_ENL1_Tdelay_NS_l2"=w2099:i32)  [unwired: 11 in]
              n1221 = call "myRIO_BRig_RT_dataLC_ENL1_Count_NS_l2.vi"() -> ("output_ENL1_Count_NS_l2"=w2100:i32)  [unwired: 11 in]
              n1222 = call "myRIO_BRig_RT_dataLC_ENL1_delayOpt_NS_l2.vi"() -> ("output_ENL1_delayOpt_NS_l2"=w2101:i32)  [unwired: 11 in]
              n1223 = local read "LC_ENL1_Count_Switch_l2"() -> (w2139:u16)
              n1224 = local read "LC_ENL1_Probability_Switch_l2"() -> (w2141:u16)
              n1225 = local read "LC_ENL1_Block_Switch_l2"() -> (w2145:u16)
              n1226 = local read "LC_ENL1_Tdelay_Switch_l2"() -> (w2140:u16)
              n1227 = local read "LC_ENL1_OnOff_Switch_l2"() -> (w2144:bool)
              n1228 = call "myRIO_BRig_RT_dataLC_Selection_Block_Switch_l2.vi"() -> ("output_Selection_Block_Switch_l2"=w2095:i32)  [unwired: 11 in]
              n1229 = call "myRIO_BRig_RT_dataLC_Selection_OnOff_Switch_l2.vi"() -> ("output_Selection_OnOff_Switch_l2"=w2094:i32)  [unwired: 11 in]
              n1230 = call "myRIO_BRig_RT_dataLC_Selection_Probability_Switch_l2.vi"() -> ("output_Selection_Probability_Switch_l1"=w2093:i32)  [unwired: 11 in]
              n1231 = call "myRIO_BRig_RT_dataLC_Selection_Tdelay_Switch_l2.vi"() -> ("output_Selection_Tdelay_Switch_l2"=w2092:i32)  [unwired: 11 in]
              n1232 = call "myRIO_BRig_RT_dataLC_Selection_Count_Switch_l2.vi"() -> ("output_Selection_Count_Switch_l2"=w2091:i32)  [unwired: 11 in]
              n1233 = local read "LC_ENL1_OnOff_NS_l2"() -> (w2122:bool)
              n1234 = local read "LC_ENL1_Probability_NS_l2"() -> (w2120:u16)
              n1235 = local read "LC_ENL1_delayOpt_NS_l2"() -> (w2118:bool)
              n1236 = local read "LC_Sel_Probability_Switch_l2"() -> (w2111:u16)
              n1237 = local read "LC_ENL1_Tdelay_NS_l2"() -> (w2116:u16)
              n1238 = local read "LC_ENL1_Block_NS_l2"() -> (w2123:u16)
              n1239 = local read "LC_ENL1_Count_NS_l2"() -> (w2119:u16)
              n1240 = local read "LC_Sel_Tdelay_Switch_l2"() -> (w2110:u16)
              n1241 = local read "LC_Sel_OnOff_Switch_l2"() -> (w2114:bool)
              n1242 = local read "LC_Sel_Count_Switch_l2"() -> (w2109:u16)
              n1243 = local read "LC_Sel_Block_Switch_l2"() -> (w2113:u16)
              n1244 = Boolean To (0,1)(Boolean=w2127) -> (0, 1=w2128:i16)
              n1245 = Boolean To (0,1)(Boolean=w2144) -> (0, 1=w2143:i16)
              n1246 = Boolean To (0,1)(Boolean=w2122) -> (0, 1=w2125:i16)
              n1247 = To Unsigned Word Integer(number=w2128) -> (unsigned 16bit integer=w2126:u16)
              n1248 = To Unsigned Word Integer(number=w2143) -> (unsigned 16bit integer=w2142:u16)
              n1249 = Boolean To (0,1)(Boolean=w2118) -> (0, 1=w2124:i16)
              n1250 = To Unsigned Word Integer(number=w2125) -> (unsigned 16bit integer=w2121:u16)
              n1251 = Boolean To (0,1)(Boolean=w2114) -> (0, 1=w2115:i16)
              n1252 = To Unsigned Word Integer(number=w2124) -> (unsigned 16bit integer=w2117:u16)
              n1253 = To Unsigned Word Integer(number=w2115) -> (unsigned 16bit integer=w2112:u16)
              n1254 = Replace Array Subset(array=w2146, new element #1=w2145, index #1=w2102, new element #2=w2142, index #2=w2103, new element #3=w2141, index #3=w2104, new element #4=w2140, index #4=w2105, new element #5=w2139, index #5=w2106, new element #6=w2126, index #6=w2107, new element #7=w2123, index #7=w2096, new element #8=w2121, index #8=w2097, new element #9=w2120, index #9=w2098, new element #10=w2116, index #10=w2099, new element #11=w2119, index #11=w2100, new element #12=w2117, index #12=w2101, new element #13=w2113, index #13=w2095, new element #14=w2112, index #14=w2094, new element #15=w2111, index #15=w2093, new element #16=w2110, index #16=w2092, new element #17=w2109, index #17=w2091) -> (w2147:u16[])
            }
            frame "saveSettings_LC_Cue_l1" {
              # "Selection All"
              # "Count"
              # "Tdelay"
              # "Probability"
              # "OnOff"
              # "Block"
              # "delayOpt"
              # "Count"
              # "Tdelay"
              # "Probability"
              # "OnOff"
              # "Block"
              # "Cue1 All"
              # "delayOpt"
              # "Count"
              # "Tdelay"
              # "Probability"
              # "OnOff"
              # "Block"
              # "Cue1 First"
              n1255 = call "myRIO_BRig_RT_dataLC_Cue1_delayOpt_Switch_l1.vi"() -> ("output_Cue1_delayOpt_Switch_l1"=w2186:i32)  [unwired: 11 in]
              n1256 = call "myRIO_BRig_RT_dataLC_Cue1_Block_Switch_l1.vi"() -> ("output_Cue1_Block_Switch_l1"=w2209:i32)  [unwired: 11 in]
              n1257 = call "myRIO_BRig_RT_dataLC_Cue1_OnOff_Switch_l1.vi"() -> ("output_Cue1_OnOff_Switch_l1"=w2207:i32)  [unwired: 11 in]
              n1258 = call "myRIO_BRig_RT_dataLC_Cue1_Probability_Switch_l1.vi"() -> ("output_Cue1_Probability_Switch_l1"=w2203:i32)  [unwired: 11 in]
              n1259 = call "myRIO_BRig_RT_dataLC_Cue1_Tdelay_Switch_l1.vi"() -> ("output_Cue1_Tdelay_Switch_l1"=w2201:i32)  [unwired: 11 in]
              n1260 = call "myRIO_BRig_RT_dataLC_Cue1_Count_Switch_l1.vi"() -> ("output_Cue1_Count_Switch_l1"=w2199:i32)  [unwired: 11 in]
              n1261 = local read "LC_Cue1_delayOpt_Switch_l1"() -> (w2185:bool)
              n1262 = call "myRIO_BRig_RT_dataLC_Cue1_Block_NS_l1.vi"() -> ("output_Cue1_Block_NS_l1"=w2183:i32)  [unwired: 11 in]
              n1263 = call "myRIO_BRig_RT_dataLC_Cue1_OnOff_NS_l1.vi"() -> ("output_Cue1_OnOff_NS_l1"=w2182:i32)  [unwired: 11 in]
              n1264 = call "myRIO_BRig_RT_dataLC_Cue1_Probability_NS_l1.vi"() -> ("output_Cue1_l1_All_Probability"=w2181:i32)  [unwired: 11 in]
              n1265 = call "myRIO_BRig_RT_dataLC_Cue1_Tdelay_NS_l1.vi"() -> ("output_Cue1_Tdelay_NS_l1"=w2180:i32)  [unwired: 11 in]
              n1266 = call "myRIO_BRig_RT_dataLC_Cue1_Count_NS_l1.vi"() -> ("output_Cue1_Count_NS_l1"=w2179:i32)  [unwired: 11 in]
              n1267 = call "myRIO_BRig_RT_dataLC_Cue1_delayOpt_NS_l1.vi"() -> ("output_Cue1_delayOpt_NS_l1"=w2178:i32)  [unwired: 11 in]
              n1268 = local read "LC_Cue1_Count_Switch_l1"() -> (w2198:u16)
              n1269 = local read "LC_Cue1_Probability_Switch_l1"() -> (w2202:u16)
              n1270 = local read "LC_Cue1_Block_Switch_l1"() -> (w2208:u16)
              n1271 = local read "LC_Cue1_Tdelay_Switch_l1"() -> (w2200:u16)
              n1272 = local read "LC_Cue1_OnOff_Switch_l1"() -> (w2206:bool)
              n1273 = local read "LC_Cue1_OnOff_NS_l1"() -> (w2174:bool)
              n1274 = call "myRIO_BRig_RT_dataLC_Selection_Block_NS_l1.vi"() -> ("output_Selection_Block_NS_l1"=w2167:i32)  [unwired: 11 in]
              n1275 = call "myRIO_BRig_RT_dataLC_Selection_OnOff_NS_l1.vi"() -> ("output_Selection_OnOff_NS_l1"=w2166:i32)  [unwired: 11 in]
              n1276 = call "myRIO_BRig_RT_dataLC_Selection_Probability_NS_l1.vi"() -> ("output_Selection_Probability_NS_l1"=w2165:i32)  [unwired: 11 in]
              n1277 = call "myRIO_BRig_RT_dataLC_Selection_Tdelay_NS_l1.vi"() -> ("output_Selection_Tdelay_NS_l1"=w2164:i32)  [unwired: 11 in]
              n1278 = call "myRIO_BRig_RT_dataLC_Selection_Count_NS_l1.vi"() -> ("output_Selection_Count_NS_l1"=w2157:i32)  [unwired: 11 in]
              n1279 = local read "LC_Cue1_delayOpt_NS_l1"() -> (w2175:bool)
              n1280 = local read "LC_Cue1_Probability_NS_l1"() -> (w2171:u16)
              n1281 = local read "LC_Cue1_Tdelay_NS_l1"() -> (w2170:u16)
              n1282 = local read "LC_Cue1_Count_NS_l1"() -> (w2169:u16)
              n1283 = local read "LC_Cue1_Block_NS_l1"() -> (w2173:u16)
              n1284 = local read "LC_Sel_Probability_NS_l1"() -> (w2159:u16)
              n1285 = local read "LC_Sel_Tdelay_NS_l1"() -> (w2158:u16)
              n1286 = local read "LC_Sel_OnOff_NS_l1"() -> (w2161:bool)
              n1287 = local read "LC_Sel_Count_NS_l1"() -> (w2156:u16)
              n1288 = local read "LC_Sel_Block_NS_l1"() -> (w2163:u16)
              n1289 = Boolean To (0,1)(Boolean=w2185) -> (0, 1=w2187:i16)
              n1290 = Boolean To (0,1)(Boolean=w2206) -> (0, 1=w2205:i16)
              n1291 = Boolean To (0,1)(Boolean=w2174) -> (0, 1=w2177:i16)
              n1292 = To Unsigned Word Integer(number=w2187) -> (unsigned 16bit integer=w2184:u16)
              n1293 = To Unsigned Word Integer(number=w2205) -> (unsigned 16bit integer=w2204:u16)
              n1294 = To Unsigned Word Integer(number=w2177) -> (unsigned 16bit integer=w2172:u16)
              n1295 = Boolean To (0,1)(Boolean=w2175) -> (0, 1=w2176:i16)
              n1296 = Boolean To (0,1)(Boolean=w2161) -> (0, 1=w2162:i16)
              n1297 = To Unsigned Word Integer(number=w2176) -> (unsigned 16bit integer=w2168:u16)
              n1298 = To Unsigned Word Integer(number=w2162) -> (unsigned 16bit integer=w2160:u16)
              n1299 = Replace Array Subset(array=w2210, new element #1=w2208, index #1=w2209, new element #2=w2204, index #2=w2207, new element #3=w2202, index #3=w2203, new element #4=w2200, index #4=w2201, new element #5=w2198, index #5=w2199, new element #6=w2184, index #6=w2186, new element #7=w2173, index #7=w2183, new element #8=w2172, index #8=w2182, new element #9=w2171, index #9=w2181, new element #10=w2170, index #10=w2180, new element #11=w2169, index #11=w2179, new element #12=w2168, index #12=w2178, new element #13=w2163, index #13=w2167, new element #14=w2160, index #14=w2166, new element #15=w2159, index #15=w2165, new element #16=w2158, index #16=w2164, new element #17=w2156, index #17=w2157) -> (w2211:u16[])
            }
            frame "saveSettings_LC_Cue_l2" {
              # "Selection All"
              # "Count"
              # "Tdelay"
              # "Probability"
              # "OnOff"
              # "Block"
              # "delayOpt"
              # "Count"
              # "Tdelay"
              # "Probability"
              # "OnOff"
              # "Block"
              # "Cue1 All"
              # "delayOpt"
              # "Count"
              # "Tdelay"
              # "Probability"
              # "OnOff"
              # "Block"
              # "Cue1 First"
              n1300 = call "myRIO_BRig_RT_dataLC_Cue1_delayOpt_Switch_l2.vi"() -> ("output_Cue1_delayOpt_Switch_l2"=w2250:i32)  [unwired: 11 in]
              n1301 = call "myRIO_BRig_RT_dataLC_Cue1_Block_Switch_l2.vi"() -> ("output_Cue1_Block_Switch_l2"=w2273:i32)  [unwired: 11 in]
              n1302 = call "myRIO_BRig_RT_dataLC_Cue1_OnOff_Switch_l2.vi"() -> ("output_Cue1_OnOff_Switch_l2"=w2271:i32)  [unwired: 11 in]
              n1303 = call "myRIO_BRig_RT_dataLC_Cue1_Probability_Switch_l2.vi"() -> ("output_Cue1_l2_First_Probability"=w2267:i32)  [unwired: 11 in]
              n1304 = call "myRIO_BRig_RT_dataLC_Cue1_Tdelay_Switch_l2.vi"() -> ("output_Cue1_Tdelay_Switch_l2"=w2265:i32)  [unwired: 11 in]
              n1305 = call "myRIO_BRig_RT_dataLC_Cue1_Count_Switch_l2.vi"() -> ("output_Cue1_Count_Switch_l2"=w2263:i32)  [unwired: 11 in]
              n1306 = local read "LC_Cue1_delayOpt_Switch_l2"() -> (w2249:bool)
              n1307 = call "myRIO_BRig_RT_dataLC_Cue1_Block_NS_l2.vi"() -> ("output_Cue1_Block_NS_l2"=w2247:i32)  [unwired: 11 in]
              n1308 = call "myRIO_BRig_RT_dataLC_Cue1_OnOff_NS_l2.vi"() -> ("output_Cue1_OnOff_NS_l2"=w2246:i32)  [unwired: 11 in]
              n1309 = call "myRIO_BRig_RT_dataLC_Cue1_Probability_NS_l2.vi"() -> ("output_Cue1_l2_All_Probability"=w2245:i32)  [unwired: 11 in]
              n1310 = call "myRIO_BRig_RT_dataLC_Cue1_Tdelay_NS_l2.vi"() -> ("output_Cue1_Tdelay_NS_l2"=w2244:i32)  [unwired: 11 in]
              n1311 = call "myRIO_BRig_RT_dataLC_Cue1_Count_NS_l2.vi"() -> ("output_Cue1_Count_NS_l2"=w2243:i32)  [unwired: 11 in]
              n1312 = call "myRIO_BRig_RT_dataLC_Cue1_delayOpt_NS_l2.vi"() -> ("output_Cue1_delayOpt_NS_l2"=w2242:i32)  [unwired: 11 in]
              n1313 = local read "LC_Cue1_Count_Switch_l2"() -> (w2262:u16)
              n1314 = local read "LC_Cue1_Probability_Switch_l2"() -> (w2266:u16)
              n1315 = local read "LC_Cue1_Block_Switch_l2"() -> (w2272:u16)
              n1316 = local read "LC_Cue1_Tdelay_Switch_l2"() -> (w2264:u16)
              n1317 = local read "LC_Cue1_OnOff_Switch_l2"() -> (w2270:bool)
              n1318 = local read "LC_Cue1_OnOff_NS_l2"() -> (w2238:bool)
              n1319 = call "myRIO_BRig_RT_dataLC_Selection_Block_NS_l2.vi"() -> ("output_Selection_Block_NS_l2"=w2223:i32)  [unwired: 11 in]
              n1320 = call "myRIO_BRig_RT_dataLC_Selection_OnOff_NS_l2.vi"() -> ("output_Selection_OnOff_NS_l2"=w2222:i32)  [unwired: 11 in]
              n1321 = call "myRIO_BRig_RT_dataLC_Selection_Probability_NS_l2.vi"() -> ("output_Selection_Probability_NS_l2"=w2221:i32)  [unwired: 11 in]
              n1322 = call "myRIO_BRig_RT_dataLC_Selection_Tdelay_NS_l2.vi"() -> ("output_Selection_Tdelay_NS_l2"=w2220:i32)  [unwired: 11 in]
              n1323 = call "myRIO_BRig_RT_dataLC_Selection_Count_NS_l2.vi"() -> ("output_Selection_Count_NS_l2"=w2219:i32)  [unwired: 11 in]
              n1324 = local read "LC_Cue1_delayOpt_NS_l2"() -> (w2239:bool)
              n1325 = local read "LC_Cue1_Probability_NS_l2"() -> (w2235:u16)
              n1326 = local read "LC_Cue1_Tdelay_NS_l2"() -> (w2234:u16)
              n1327 = local read "LC_Cue1_Count_NS_l2"() -> (w2233:u16)
              n1328 = local read "LC_Cue1_Block_NS_l2"() -> (w2237:u16)
              n1329 = local read "LC_Sel_Probability_NS_l2"() -> (w2227:u16)
              n1330 = local read "LC_Sel_Tdelay_NS_l2"() -> (w2226:u16)
              n1331 = local read "LC_Sel_OnOff_NS_l2"() -> (w2229:bool)
              n1332 = local read "LC_Sel_Count_NS_l2"() -> (w2225:u16)
              n1333 = local read "LC_Sel_Block_NS_l2"() -> (w2231:u16)
              n1334 = Boolean To (0,1)(Boolean=w2249) -> (0, 1=w2251:i16)
              n1335 = Boolean To (0,1)(Boolean=w2270) -> (0, 1=w2269:i16)
              n1336 = Boolean To (0,1)(Boolean=w2238) -> (0, 1=w2241:i16)
              n1337 = To Unsigned Word Integer(number=w2251) -> (unsigned 16bit integer=w2248:u16)
              n1338 = To Unsigned Word Integer(number=w2269) -> (unsigned 16bit integer=w2268:u16)
              n1339 = To Unsigned Word Integer(number=w2241) -> (unsigned 16bit integer=w2236:u16)
              n1340 = Boolean To (0,1)(Boolean=w2239) -> (0, 1=w2240:i16)
              n1341 = Boolean To (0,1)(Boolean=w2229) -> (0, 1=w2230:i16)
              n1342 = To Unsigned Word Integer(number=w2240) -> (unsigned 16bit integer=w2232:u16)
              n1343 = To Unsigned Word Integer(number=w2230) -> (unsigned 16bit integer=w2228:u16)
              n1344 = Replace Array Subset(array=w2274, new element #1=w2272, index #1=w2273, new element #2=w2268, index #2=w2271, new element #3=w2266, index #3=w2267, new element #4=w2264, index #4=w2265, new element #5=w2262, index #5=w2263, new element #6=w2248, index #6=w2250, new element #7=w2237, index #7=w2247, new element #8=w2236, index #8=w2246, new element #9=w2235, index #9=w2245, new element #10=w2234, index #10=w2244, new element #11=w2233, index #11=w2243, new element #12=w2232, index #12=w2242, new element #13=w2231, index #13=w2223, new element #14=w2228, index #14=w2222, new element #15=w2227, index #15=w2221, new element #16=w2226, index #16=w2220, new element #17=w2225, index #17=w2219) -> (w2275:u16[])
            }
            frame "saveSettings6_LC_l1_Other" {
              # "Trial"
              # "Tdelay"
              # "Probability"
              # "OnOff"
              # "Block"
              # "Wrong"
              # "Trial"
              # "Tdelay"
              # "Probability"
              # "OnOff"
              # "Block"
              # "Reward"
              n1345 = call "myRIO_BRig_RT_dataLC_Wrong_Block_l1.vi"() -> ("output_Wrong_Block_l1"=w2304:i32)  [unwired: 11 in]
              n1346 = call "myRIO_BRig_RT_dataLC_Wrong_OnOff_l1.vi"() -> ("output_Wrong_OnOff_l1"=w2303:i32)  [unwired: 11 in]
              n1347 = call "myRIO_BRig_RT_dataLC_Wrong_Probability_l1.vi"() -> ("output_Wrong_Probability_l1"=w2302:i32)  [unwired: 11 in]
              n1348 = call "myRIO_BRig_RT_dataLC_Wrong_Tdelay_l1.vi"() -> ("output_Wrong_Tdelay_l1"=w2301:i32)  [unwired: 11 in]
              n1349 = call "myRIO_BRig_RT_dataLC_Wrong_Trial_l1.vi"() -> ("output_Wrong_Trial_l1"=w2300:i32)  [unwired: 11 in]
              n1350 = call "myRIO_BRig_RT_dataLC_Reward_Block_l1.vi"() -> ("output_Reward_Block_l1"=w2316:i32)  [unwired: 11 in]
              n1351 = call "myRIO_BRig_RT_dataLC_Reward_OnOff_l1.vi"() -> ("output_Reward_OnOff_l1"=w2314:i32)  [unwired: 11 in]
              n1352 = call "myRIO_BRig_RT_dataLC_Reward_Probability_l1.vi"() -> ("output_Reward_Probability_l1"=w2310:i32)  [unwired: 11 in]
              n1353 = call "myRIO_BRig_RT_dataLC_Reward_Tdelay_l1.vi"() -> ("output_Reward_Tdelay_l1"=w2308:i32)  [unwired: 11 in]
              n1354 = call "myRIO_BRig_RT_dataLC_Reward_Trial_l1.vi"() -> ("output_Reward_Trial_l1"=w2306:i32)  [unwired: 11 in]
              n1355 = local read "LC_Wrong_OnOff_l1"() -> (w2298:bool)
              n1356 = local read "LC_Wrong_Probability_l1"() -> (w2295:u16)
              n1357 = local read "LC_Wrong_Block_l1"() -> (w2297:u16)
              n1358 = local read "LC_Wrong_Tdelay_l1"() -> (w2294:u16)
              n1359 = local read "LC_Wrong_Trial_l1"() -> (w2293:u16)
              n1360 = local read "LC_Reward_Probability_l1"() -> (w2309:u16)
              n1361 = local read "LC_Reward_Block_l1"() -> (w2315:u16)
              n1362 = local read "LC_Reward_Tdelay_l1"() -> (w2307:u16)
              n1363 = local read "LC_Reward_OnOff_l1"() -> (w2313:bool)
              n1364 = local read "LC_Reward_Trial_l1"() -> (w2305:u16)
              n1365 = Boolean To (0,1)(Boolean=w2298) -> (0, 1=w2299:i16)
              n1366 = Boolean To (0,1)(Boolean=w2313) -> (0, 1=w2312:i16)
              n1367 = To Unsigned Word Integer(number=w2299) -> (unsigned 16bit integer=w2296:u16)
              n1368 = To Unsigned Word Integer(number=w2312) -> (unsigned 16bit integer=w2311:u16)
              n1369 = Replace Array Subset(array=w2317, new element #1=w2315, index #1=w2316, new element #2=w2311, index #2=w2314, new element #3=w2309, index #3=w2310, new element #4=w2307, index #4=w2308, new element #5=w2305, index #5=w2306, new element #6=w2297, index #6=w2304, new element #7=w2296, index #7=w2303, new element #8=w2295, index #8=w2302, new element #9=w2294, index #9=w2301, new element #10=w2293, index #10=w2300) -> (w2318:u16[])
            }
            frame "SaveSettings6_LC_l2_Other" {
              # "Trial"
              # "Tdelay"
              # "Probability"
              # "OnOff"
              # "Block"
              # "Wrong"
              # "Trial"
              # "Tdelay"
              # "Probability"
              # "OnOff"
              # "Block"
              # "Reward"
              n1370 = call "myRIO_BRig_RT_dataLC_Wrong_Block_l2.vi"() -> ("output_Wrong_Block_l2"=w2327:i32)  [unwired: 11 in]
              n1371 = call "myRIO_BRig_RT_dataLC_Wrong_OnOff_l2.vi"() -> ("output_Wrong_OnOff_l2"=w2328:i32)  [unwired: 11 in]
              n1372 = call "myRIO_BRig_RT_dataLC_Wrong_Probability_l2.vi"() -> ("output_Wrong_Probability_l2"=w2329:i32)  [unwired: 11 in]
              n1373 = call "myRIO_BRig_RT_dataLC_Wrong_Tdelay_l2.vi"() -> ("output_Wrong_Tdelay_l2"=w2330:i32)  [unwired: 11 in]
              n1374 = call "myRIO_BRig_RT_dataLC_Wrong_Trial_l2.vi"() -> ("output_Wrong_Trial_l2"=w2331:i32)  [unwired: 11 in]
              n1375 = call "myRIO_BRig_RT_dataLC_Reward_Block_l2.vi"() -> ("output_Reward_Block_l2"=w2332:i32)  [unwired: 11 in]
              n1376 = call "myRIO_BRig_RT_dataLC_Reward_OnOff_l2.vi"() -> ("output_Reward_OnOff_l2"=w2333:i32)  [unwired: 11 in]
              n1377 = call "myRIO_BRig_RT_dataLC_Reward_Probability_l2.vi"() -> ("output_Reward_Probability_l2"=w2334:i32)  [unwired: 11 in]
              n1378 = call "myRIO_BRig_RT_dataLC_Reward_Tdelay_l2.vi"() -> ("output_Reward_Tdelay_l2"=w2335:i32)  [unwired: 11 in]
              n1379 = call "myRIO_BRig_RT_dataLC_Reward_Trial_l2.vi"() -> ("output_Reward_Trial_l2"=w2336:i32)  [unwired: 11 in]
              n1380 = local read "LC_Wrong_OnOff_l2"() -> (w2352:bool)
              n1381 = local read "LC_Wrong_Probability_l2"() -> (w2349:u16)
              n1382 = local read "LC_Wrong_Block_l2"() -> (w2351:u16)
              n1383 = local read "LC_Wrong_Tdelay_l2"() -> (w2348:u16)
              n1384 = local read "LC_Wrong_Trial_l2"() -> (w2347:u16)
              n1385 = local read "LC_Reward_Probability_l2"() -> (w2356:u16)
              n1386 = local read "LC_Reward_Block_l2"() -> (w2360:u16)
              n1387 = local read "LC_Reward_Tdelay_l2"() -> (w2355:u16)
              n1388 = local read "LC_Reward_OnOff_l2"() -> (w2359:bool)
              n1389 = local read "LC_Reward_Trial_l2"() -> (w2354:u16)
              n1390 = Boolean To (0,1)(Boolean=w2352) -> (0, 1=w2353:i16)
              n1391 = Boolean To (0,1)(Boolean=w2359) -> (0, 1=w2358:i16)
              n1392 = To Unsigned Word Integer(number=w2353) -> (unsigned 16bit integer=w2350:u16)
              n1393 = To Unsigned Word Integer(number=w2358) -> (unsigned 16bit integer=w2357:u16)
              n1394 = Replace Array Subset(array=w2361, new element #1=w2360, index #1=w2332, new element #2=w2357, index #2=w2333, new element #3=w2356, index #3=w2334, new element #4=w2355, index #4=w2335, new element #5=w2354, index #5=w2336, new element #6=w2351, index #6=w2327, new element #7=w2350, index #7=w2328, new element #8=w2349, index #8=w2329, new element #9=w2348, index #9=w2330, new element #10=w2347, index #10=w2331) -> (w2362:u16[])
            }
            frame "setSettings_Audio" {
              # "amp_L"
              # "amp_R"
              # "freq_L"
              # "freq_R"
              n1395 = call "myRIO_BRig_RT_dataExp_Audio_amp__L.vi"() -> ("output_Audio_amp__L"=w2387:i32)  [unwired: 11 in]
              n1396 = call "myRIO_BRig_RT_dataExp_Audio_amp__R.vi"() -> ("output_Audio_amp__R"=w2386:i32)  [unwired: 11 in]
              n1397 = call "myRIO_BRig_RT_dataExp_Audio_freq__L.vi"() -> ("output_Audio_freq__L"=w2385:i32)  [unwired: 11 in]
              n1398 = call "myRIO_BRig_RT_dataExp_Audio_freq__R.vi"() -> ("output_Audio_freq__R"=w2384:i32)  [unwired: 11 in]
              n1399 = Index Array(array=w2383, index #1=w2387, index #2=w2386, index #3=w2385, index #4=w2384) -> (element #1=w2382:u16, element #2=w2381:u16, element #3=w2374:u16, element #4=w2372:u16)
              n1400 = To Unsigned Byte Integer(number=w2374) -> (unsigned 8bit integer=w2373:u8)
              n1401 = To Unsigned Byte Integer(number=w2372) -> (unsigned 8bit integer=w2371:u8)
            }
            frame "setSettings_Laser" {
              w2413 = u32 0 ("laser2_selRew_Ndelay")
              # "tDelay"
              # "Wrong l1"
              # "Reward l1"
              n1402 = local read "Laser_Tpeak_l1"() -> (w2424:dbl)
              n1403 = local read "Laser_Tshutter_l1"() -> (w2422:dbl)
              n1404 = local read "Laser_Freq_l1"() -> (w2423:dbl)
              n1405 = local read "Laser_duration_l1"() -> (w2398:u16)
              n1406 = local read "Laser_Tpeak_l2"() -> (w2420:dbl)
              n1407 = local read "Laser_Tshutter_l2"() -> (w2418:dbl)
              n1408 = local read "Laser_Freq_l2"() -> (w2419:dbl)
              n1409 = local read "Laser_duration_l2"() -> (w2397:u16)
              n1410 = local read "CueLed_Freq"() -> (w2407:dbl)
              n1411 = local read "CueLed_Tpeak"() -> (w2408:dbl)
              n1412 = call "myRIO_BRig_RT_dataLC_Reward_Tdelay_l1.vi"() -> ("output_Reward_Tdelay_l1"=w2436:i32)  [unwired: 11 in]
              n1413 = call "myRIO_BRig_RT_dataLC_Wrong_Tdelay_l1.vi"() -> ("output_Wrong_Tdelay_l1"=w2437:i32)  [unwired: 11 in]
              n1414 = local read "FPGA_count2ms"() -> (w2409:dbl)
              n1415 = Index Array(array=w2404, index #1=w2436, index #2=w2437) -> (element #1=w2435:u16, element #2=w2434:u16)
              n1416 = To Double Precision Float(number=w2435) -> (double precision float=w2431:dbl)
              n1417 = To Double Precision Float(number=w2434) -> (double precision float=w2428:dbl)
              n1418 = To Unsigned Word Integer(number=w2409) -> (unsigned 16bit integer=w2425:u16)
              n1419 = call "myRIO_BRig_RT__calc_laser_FPGA_N.vi"("input_FPGA_ms2count"=w2409, "input_Tpeak"=w2424, "input_Freq"=w2423, "input_Tshutter"=w2422, "input_duration"=w2398) -> ("output_laser_Npeak"=w2412:u32, "output_laser_Nvalley"=w2411:u32, "output_laser_Nshutter"=w2410:u32, "output_laser_Nduration"=w2421:u32, "output_laser_Tduration"=w2402:u16)  [unwired: 6 in]
              n1420 = Multiply(x=w2409, y=w2431) -> (x*y=w2432:dbl)
              n1421 = Multiply(x=w2409, y=w2428) -> (x*y=w2429:dbl)
              n1422 = call "myRIO_BRig_RT__calc_laser_FPGA_N__CueLed.vi"("input_FPGA_ms2count"=w2409, "input_Tpeak"=w2408, "input_Freq"=w2407) -> ("output_laser_Npeak"=w2406:u32, "output_laser_Nvalley"=w2405:u32)  [unwired: 11 in]
              n1423 = call "myRIO_BRig_RT__calc_laser_FPGA_N.vi"("input_FPGA_ms2count"=w2409, "input_Tpeak"=w2420, "input_Freq"=w2419, "input_Tshutter"=w2418, "input_duration"=w2397) -> ("output_laser_Npeak"=w2417:u32, "output_laser_Nvalley"=w2416:u32, "output_laser_Nshutter"=w2415:u32, "output_laser_Nduration"=w2414:u32, "output_laser_Tduration"=w2401:u16)  [unwired: 6 in]
              n1424 = Round Toward +Infinity(x=w2432) -> (ceil(x): smallest int >= x=w2433:dbl)
              n1425 = Round Toward +Infinity(x=w2429) -> (ceil(x): smallest int >= x=w2430:dbl)
              n1426 = To Unsigned Long Integer(number=w2433) -> (unsigned 32bit integer=w2427:u32)
              n1427 = To Unsigned Long Integer(number=w2430) -> (unsigned 32bit integer=w2426:u32)
              n1428 = xnode "Read/Write Control"("FPGA VI Reference In"=w2438, "error in"=w2439, "LC_nPeak_l1"=w2412, "LC_nValley_l1"=w2411, "LC_nShutter_l1"=w2410, "LR_reward_nDelay_l1"=w2427, "LR_wrong_nDelay_l1"=w2426, "LR_reward_nTotal_l1"=w2421, "LR_wrong_nTotal_l1"=w2421, "k1__counter_per_ms"=w2425, "LC_nPeak_l2"=w2417, "LC_nValley_l2"=w2416, "LC_nShutter_l2"=w2415, "LR_reward_nDelay_l2"=w2413, "LR_wrong_nDelay_l2"=w2413, "LR_reward_nTotal_l2"=w2414, "LR_wrong_nTotal_l2"=w2414, "CueLed_nPeak"=w2406, "CueLed_nValley"=w2405) -> ("error out"=→"error out":errorcluster)  [unwired: 1 out]
              n1429 = call "myRIO_BRig_RT_dataCurrent_laser1_pulse_duration.vi"() -> ("output_laser1_pulse_duration"=w2400:i32)  [unwired: 11 in]
              n1430 = call "myRIO_BRig_RT_dataCurrent_laser2_pulse_duration.vi"() -> ("output_laser2_pulse_duration"=w2399:i32)  [unwired: 11 in]
              n1431 = Replace Array Subset(array=w2404, new element #1=w2402, index #1=w2400, new element #2=w2401, index #2=w2399) -> (w2403:u16[])
            }
            frame "initBlock" {
              n1432 = local write "nRewards_cur"(u16 0 ("nRewards_cur")) -> ()
              n1433 = call "myRIO_Brig_RT__Case_Exp_State_initBlock__v2.vi"("input_spout"=w2464, "input_dataCurrent"=w2470, "input_dataExp"=w2467, "input_dataBlock"=w2459) -> ("output_state"=w2463:T2, "output_spout"=w2462:enum16{"Left", "Right"}, "idxDataBlock"=w2465:i32, "output_dataCurrent"=w2469:u16[], "output_dataExp"=w2468:u16[], "output_TpB_target"=→"TpB_target":u16, "output_iBlock"=w2460:u16, "output_dataBlock"=w2458:u16[][])  [unwired: 4 in]
              "iBlock" <- w2460
              "cSpout" <- w2462
            }
            frame "initBlock2" {
              n1434 = call "myRIO_BRig_RT__Case_Exp_State_initBlock2.vi"("input_spout"=w2491, "input_dataBlock"=w2492, "input_dataCurrent"=w2490) -> ("idxDataBlock"=w2487:i32, "output_dataBlock"=w2489:u16[][])  [unwired: 7 in]
            }
            frame "initTrial" {
              n1435 = xnode "Read/Write Control"("FPGA VI Reference In"=w2511, "error in"=w2510, "SelectionState"=FALSE) -> ("error out"=w2509:errorcluster)  [unwired: 1 out]
              n1436 = call "myRIO_Brig_RT__Case_Exp_State_initTrial__v2.vi"("input_spout"=w2512, "input_dataBlock"=w2507, "input_dataExp"=w2527, "input_dataCurrent"=w2528) -> ("output_state"=w2529:T2, "output_dataExp"=w2526:u16[], "output_dataCurrent"=w2517:u16[], "output_iTrial"=w2506:u16, "output_SolenoidReward"=→"SolenoidReward":bool)  [unwired: 3 in]
              "iTrial" <- w2506
              n1437 = local write "error out"(w2509) -> ()
            }
            frame "initTrial2" {
              # "trialUntilReward"
              n1438 = call "myRIO_BRig_RT__Case_Exp_subState_LC__initTrial__v3.vi"("input_dataCurrent"=w2543, "input_dataLC"=w2542, "input_spout"=w2544, "input_dataTrial"=w2546) -> ("output_dataTrial"=w2545:u16[][], "output_LR_Wrong_Laser_l2"=w2534:bool, "output_LR_Reward_Laser_l2"=w2535:bool, "output_LR_Reward_Event_l1"=w2541:bool, "output_LR_Wrong_Event_l1"=w2540:bool, "output_LR_Reward_Laser_l1"=w2539:bool, "output_LR_Wrong_Laser_l1"=w2538:bool, "output_LR_Reward_Event_l2"=w2537:bool, "output_LR_Wrong_Event_l2"=w2536:bool)  [unwired: 7 in]
              n1439 = call "myRIO_BRig_RT_dataExp_ItrialUntilReward.vi"() -> ("output_I_trialUntilReward"=w2550:i32)  [unwired: 11 in]
              n1440 = Index Array(array=w2551, index=w2550) -> (element=w2549:u16)
              n1441 = Equal?(x=w2544, y=enum16{"Left", "Right"}."Right") -> (x = y?=w2548:bool)
              n1442 = Not Equal To 0?(x=w2549) -> (x != 0?=w2547:bool)
              n1443 = xnode "Read/Write Control"("FPGA VI Reference In"=w2565, "error in"=w2564, "Left(F)_or_Right(T)"=w2548, "ignoreWrong"=w2547, "LR_reward_Event_l1"=w2541, "LR_wrong_Event_l1"=w2540, "LR_reward_Laser_l1"=w2539, "LR_wrong_Laser_l1"=w2538, "LR_reward_Event_l2"=w2537, "LR_wrong_Event_l2"=w2536, "LR_reward_Laser_l2"=w2535, "LR_wrong_laser_l2"=w2534) -> ("error out"=w2533:errorcluster)  [unwired: 1 out]
              n1444 = local write "error out"(w2533) -> ()
            }
            frame "initTrial3" {
              # "Cue1_CueType"
              n1445 = call "myRIO_BRig_RT_dataExp_CueLed.vi"() -> ("output_CueLed"=w2572:i32)  [unwired: 11 in]
              n1446 = call "myRIO_BRig_RT_arrTrig_init.vi"() -> ("output_arrTrig"=w2576:bool[])  [unwired: 11 in]
              n1447 = Index Array(array=w2573, index=w2572) -> (element=w2571:u16)
              n1448 = call "myRIO_BRig_RT_arrTrig_Cue1_CueType_AudioLed.vi"() -> ("output_arrTrig_Cue1_CueType_AudioLed"=w2574:i32)  [unwired: 11 in]
              n1449 = Not Equal To 0?(x=w2571) -> (x != 0?=w2570:bool)
              n1450 = call "myRIO_BRig_RT__Case_Exp_State_initTrial_dataTrial.vi"("input_spout"=w2591, "input_dataCurrent"=w2578, "input_dataExp"=w2573, "input_dataTrial"=w2593) -> ("output_laserPower_l2"=w2580:u16, "output_dataCurrent"=w2577:u16[], "output_dataTrial"=w2592:u16[][], "output_laserPower_l1"=w2588:u16)  [unwired: 4 in]
              n1451 = To Double Precision Float(number=w2588) -> (double precision float=w2590:dbl)
              n1452 = To Double Precision Float(number=w2580) -> (double precision float=w2583:dbl)
              n1453 = Replace Array Subset(array=w2576, new element=w2570, index=w2574) -> (w2575:bool[])
              n1454 = Divide(x=w2590, y=100.0 ("x")) -> (x/y=w2585:dbl)
              "power_l1" <- w2585
              n1455 = Divide(x=w2583, y=100.0 ("x")) -> (x/y=w2581:dbl)
              "power_l2" <- w2581
              n1456 = call "myRIO__convert__Voltage_to_FPGAvalue.vi"("input_voltage"=w2585) -> ("output_PortC"=w2584:i16)  [unwired: 9 in, 1 out]
              n1457 = call "myRIO__convert__Voltage_to_FPGAvalue.vi"("input_voltage"=w2581) -> ("output_PortC"=w2579:i16)  [unwired: 9 in, 1 out]
              n1458 = xnode "Read/Write Control"("FPGA VI Reference In"=w2587, "error in"=w2586, "AnaOut_0"=w2584, "AnaOut_1"=w2579) -> ("error out"=w2569:errorcluster)  [unwired: 1 out]
              n1459 = local write "error out"(w2569) -> ()
            }
            frame "initTrial4" {
              n1460 = call "myRIO_BRig_RT_dataCurrent_idxDataTrial.vi"() -> ("output_idxDataTrial"=w2617:i32)  [unwired: 11 in]
              n1461 = call "myRIO_BRig_RT_dataTrial_activeRecording.vi"() -> ("output_activeRecording"=w2614:i32)  [unwired: 11 in]
              n1462 = Index Array(array=w2619, index=w2617) -> (element=w2616:u16)
              n1463 = Boolean To (0,1)(Boolean="Recording") -> (0, 1=w2613:i16)
              n1464 = To Long Integer(number=w2616) -> (32bit integer=w2615:i32)
              n1465 = To Unsigned Word Integer(number=w2613) -> (unsigned 16bit integer=w2612:u16)
              n1466 = Replace Array Subset(array=w2618, new element=w2612, index (row)=w2615, index (col)=w2614) -> (w2611:u16[][])
            }
            frame "initTrial_LC_ENL1" {
              n1467 = call "myRIO_BRig_RT__Case_Exp_State_initTrial_LC_ENL1__v4.vi"("input_dataTrial"=w2642, "input_spout"=w2645, "input_arrTrig"=w2639, "input_dataBlock"=w2640, "input_dataLC"=w2646, "input_dataCurrent"=w2644) -> ("output_arrTrig"=w2638:bool[], "output_dataTrial"=w2641:u16[][], "output_dataCurrent"=w2643:u16[])  [unwired: 3 in]
            }
            frame "initTrial_LC_Cue1" {
              n1468 = call "myRIO_BRig_RT__Case_Exp_State_initTrial_LC_Cue1__v4.vi"("input_dataTrial"=w2664, "input_spout"=w2667, "input_arrTrig"=w2661, "input_dataBlock"=w2662, "input_dataLC"=w2668, "input_dataCurrent"=w2666) -> ("output_arrTrig"=w2660:bool[], "output_dataTrial"=w2663:u16[][], "output_dataCurrent"=w2665:u16[])  [unwired: 3 in]
            }
            frame "initTrial_LC_Cue1_2" {
              w2696 = TRUE ("Recording")
              n1469 = local read "Cue1Param_AudioLed_Probability_Switch"() -> (w2689:u16)
              n1470 = local read "Cue1Param_AudioLed_Count_Switch"() -> (w2688:u16)
              n1471 = local read "Cue1Param_AudioLed_Probability_NS"() -> (w2686:u16)
              n1472 = local read "Cue1Param_AudioLed_Count_NS"() -> (w2685:u16)
              n1473 = local read "Cue1Param_CueType_Switch"() -> (w2690:u16)
              n1474 = local read "Cue1Param_CueType_NS"() -> (w2687:u16)
              n1475 = call "myRIO_BRig_RT__Case_Exp_State_initTrial_LC_Cue1_2.vi"("input_CueType_Switch"=w2690, "input_Probability_Switch"=w2689, "input_Count_Switch"=w2688, "input_CueType_NS"=w2687, "input_Probability_NS"=w2686, "input_Count_NS"=w2685, "input_spout"=w2684, "input_dataBlock"=w2683, "input_dataCurrent"=w2694, "input_arrTrig"=w2692) -> ("output_dataCurrent"=w2693:u16[], "output_arrTrig"=w2691:bool[])  [unwired: 8 in]
            }
            frame "initTrial_LC_Sel" {
              n1476 = call "myRIO_BRig_RT__Case_Exp_State_initTrial_LC_Sel__v4.vi"("input_dataTrial"=w2718, "input_spout"=w2721, "input_arrTrig"=w2713, "input_dataBlock"=w2716, "input_dataLC"=w2722, "input_dataCurrent"=w2720) -> ("output_arrTrig"=w2712:bool[], "output_dataTrial"=w2717:u16[][], "output_dataCurrent"=w2719:u16[])  [unwired: 3 in]
              n1477 = local read "Recording"() -> (w2715:bool)
            }
            frame "ENL1_pre" {
              n1478 = call "myRIO_BRig_RT__Case_Exp_State_Enl1Pre__v3.vi"("input_I_lick"=w2740, "input_arrTrig"=w2737, "input_dataCurrent"=w2741) -> ("output_dataCurrent"=w2738:u16[], "output_state"=w2739:T2)  [unwired: 3 in, 4 out]
            }
            frame "ENL1" {
              n1479 = call "myRIO_BRig_RT__Case_Exp_State_ENL1__v3.vi"("I_lick"=w2764, "input_arrTrig"=w2762, "input_state"=w2768, "input_dataCurrent"=w2767) -> ("output_l1_laserOn"=w2760:bool, "output_l1_laserEvent"=w2761:bool, "output_state"=w2765:T2, "output_dataCurrent"=w2766:u16[], "output_l2_laserEvent"=w2759:bool, "output_l2_laserOn"=w2758:bool)  [unwired: 2 in]
            }
            frame "ENL1Penalty_pre" {
              # "Tcycle"
              # "counter"
              n1480 = call "myRIO_BRig_RT_dataCurrent_Tcycle_generic.vi"() -> ("output_Tcycle_generic"=w2803:i32)  [unwired: 11 in]
              n1481 = call "myRIO_BRig_RT_dataCurrent_count_generic.vi"() -> ("output_count_generic"=w2805:i32)  [unwired: 11 in]
              n1482 = call "myRIO_BRig_RT_dataExp_ENL_penalty.vi"() -> ("output_ENL_penalty"=w2798:i32)  [unwired: 11 in]
              n1483 = Index Array(array=w2799, index=w2798) -> (element=w2802:u16)
              n1484 = Replace Array Subset(array=w2800, new element #1=u16 0 ("new element/subarray"), index #1=w2805, new element #2=w2802, index #2=w2803) -> (w2801:u16[])
            }
            frame "ENL1Penalty" {
              n1485 = call "myRIO_BRig_RT__Case_Exp_State_ENL1Penalty.vi"("input_state"=w2823, "input_dataCurrent"=w2827) -> ("output_state"=w2824:T2, "output_dataCurrent"=w2826:u16[])  [unwired: 8 in]
            }
            frame "ENL2_pre" {
            }
            frame "ENL2" {
            }
            frame "ENL2Penalty_pre" {
            }
            frame "ENL2Penalty" {
            }
            frame "Cue1_pre" {
              n1486 = call "myRIO_BRig_RT__Case_Exp_State_Cue1Pre__v3.vi"("input_dataCurrent"=w2915, "input_dataExp"=w2911, "input_arrTrig"=w2908, "input_spout"=w2912) -> ("output_audioR"=w2909:bool, "output_audioL"=w2910:bool, "output_state"=w2913:T2, "output_dataCurrent"=w2914:u16[])  [unwired: 7 in, 5 out]
            }
            frame "Cue1" {
              n1487 = call "myRIO_BRig_RT__Case_Exp_State_Cue1__v3.vi"("I_lick"=w2938, "input_arrTrig"=w2936, "input_state"=w2940, "input_dataCurrent"=w2958) -> ("output_l1_laserOn"=w2934:bool, "output_l1_laserEvent"=w2935:bool, "output_state"=w2939:T2, "output_dataCurrent"=w2957:u16[], "output_l2_laserEvent"=w2933:bool, "output_CueLed_Event"=w2931:bool, "output_l2_laserOn"=w2932:bool)  [unwired: 1 in]
              n1488 = Equal?(x=myRIO_BRig_RT__Case_Exp_stateList."Selection_pre", y=w2939) -> (x = y?=w2943:bool)
              n1489 = xnode "Read/Write Control"("FPGA VI Reference In"=w2942, "error in"=w2941, "SelectionState"=w2943) -> ()  [unwired: 2 out]
            }
            frame "Cue1Penalty_pre" {
              # "Tcycle"
              # "counter"
              n1490 = call "myRIO_BRig_RT_dataCurrent_Tcycle_generic.vi"() -> ("output_Tcycle_generic"=w2990:i32)  [unwired: 11 in]
              n1491 = call "myRIO_BRig_RT_dataCurrent_count_generic.vi"() -> ("output_count_generic"=w2992:i32)  [unwired: 11 in]
              n1492 = call "myRIO_BRig_RT_dataExp_CueLed.vi"() -> ("output_CueLed"=w2970:i32)  [unwired: 11 in]
              n1493 = call "myRIO_BRig_RT_dataExp_Tcycle_Cue1Penalty_Audio.vi"() -> ("output_Tcycle_Cue1Penalty_Audio"=w2971:i32)  [unwired: 11 in]
              n1494 = call "myRIO_BRig_RT_dataExp_Tcycle_Cue1Penalty_LED.vi"() -> ("output_Tcycle_Cue1Penalty_LED"=w2969:i32)  [unwired: 11 in]
              n1495 = Index Array(array=w2986, index #1=w2970, index #2=w2971, index #3=w2969) -> (element #1=w2968:u16, element #2=w2966:u16, element #3=w2965:u16)
              n1496 = Equal To 0?(x=w2968) -> (x = 0?=w2967:bool)
              n1497 = Select(t=w2966, s=w2967, f=w2965) -> (s? t:f=w2964:u16)
              n1498 = Replace Array Subset(array=w2988, new element #1=u16 0 ("new element/subarray"), index #1=w2992, new element #2=w2964, index #2=w2990) -> (w2987:u16[])
            }
            frame "Cue1Penalty" {
              n1499 = call "myRIO_BRig_RT__Case_Exp_State_Cue1Penalty.vi"("input_state"=w3013, "input_dataCurrent"=w3014) -> ("output_state"=w3011:T2, "output_dataCurrent"=w3012:u16[])  [unwired: 8 in]
            }
            frame "Cue2_pre" {
            }
            frame "Cue2" {
            }
            frame "Cue2Penalty_pre" {
            }
            frame "Cue2Penalty" {
            }
            frame "Selection_pre" {
              n1500 = xnode "Read/Write Control"("FPGA VI Reference In"=w3106, "error in"=w3107) -> ("error out"=w3094:errorcluster, "SelectReward"=w3101:bool, "SelectWrong"=w3102:bool)  [unwired: 1 out]
              n1501 = local write "error out"(w3094) -> ()
              n1502 = call "myRIO_BRig_RT__Case_Exp_State_SelectPre__v3.vi"("input_dataCurrent"=w3105, "input_SelectWrong"=w3102, "input_SelectReward"=w3101, "input_dataExp"=w3095, "input_arrTrig"=w3100) -> ("output_state"=w3103:T2, "output_dataCurrent"=w3104:u16[], "output_l1_laserEvent"=w3099:bool, "output_l1_laserOn"=w3098:bool, "output_l2_laserOn"=w3096:bool, "output_l2_laserEvent"=w3097:bool)  [unwired: 5 in]
            }
            frame "Selection" {
              n1503 = xnode "Read/Write Control"("FPGA VI Reference In"=w3137, "error in"=w3136) -> ("error out"=w3124:errorcluster, "SelectReward"=w3131:bool, "SelectWrong"=w3130:bool)  [unwired: 1 out]
              n1504 = local write "error out"(w3124) -> ()
              n1505 = call "myRIO_BRig_RT__Case_Exp_State_Selection__v2.vi"("input_dataCurrent"=w3135, "input_state"=w3133, "input_FPGA_SelectReward"=w3131, "input_FPGA_SelectWrong"=w3130, "input_arrTrig"=w3129) -> ("output_state"=w3132:T2, "output_dataCurrent"=w3134:u16[], "output_LC_Event_l1"=w3128:bool, "output_LC_Laser_l2"=w3125:bool, "output_LC_Event_l2"=w3126:bool, "output_LC_Laser_l1"=w3127:bool)  [unwired: 5 in]
            }
            frame "SelectReward_pre" {
              # "iState"
              # "Tcycle\nReward"
              # "nRewTrials"
              # "Tcycle\nGeneric"
              # "counter"
              n1506 = call "myRIO_BRig_RT_dataCurrent_nRewTrials.vi"() -> ("output_nRewTrials"=w3169:i32)  [unwired: 11 in]
              n1507 = Equal?(x=w3178, y=enum16{"Left", "Right"}."Left") -> (x = y?=w3179:bool)
              n1508 = Index Array(array=w3170, index=w3169) -> (element=w3168:u16)
              n1509 = call "myRIO_BRig_RT_dataExp_Tcycle_Reward__L.vi"() -> ("output_Tcycle_Reward__L"=w3182:i32)  [unwired: 11 in]
              n1510 = call "myRIO_BRig_RT_dataExp_Tcycle_Reward__R.vi"() -> ("output_Tcycle_Reward__R"=w3183:i32)  [unwired: 11 in]
              n1511 = Increment(x=w3168) -> (x+1=w3167:u16)
              n1512 = Select(t=w3182, s=w3179, f=w3183) -> (s? t:f=w3181:i32)
              n1513 = call "myRIO_BRig_RT__Case_Exp_subState_LC__Reward.vi"("input_spout"=w3178, "input_dataCurrent"=w3170, "input_dataLC"=w3177) -> ()  [unwired: 6 in, 2 out]
              n1514 = call "myRIO_BRig_RT_dataCurrent_count_generic.vi"() -> ("output_count_generic"=w3172:i32)  [unwired: 11 in]
              n1515 = call "myRIO_BRig_RT_dataCurrent_Tcycle_generic.vi"() -> ("output_Tcycle_generic"=w3173:i32)  [unwired: 11 in]
              n1516 = Index Array(array=w3184, index=w3181) -> (element=w3174:u16)
              n1517 = call "myRIO_BRig_RT_dataCurrent_iState.vi"() -> ("output_iState"=w3162:i32)  [unwired: 11 in]
              n1518 = Replace Array Subset(array=w3170, new element #1=w3167, index #1=w3169, new element #2=u16 0 ("new element/subarray"), index #2=w3172, new element #3=w3174, index #3=w3173, new element #4=u16 1 ("new element/subarray"), index #4=w3162) -> (w3185:u16[])
            }
            frame "SelectReward" {
              n1519 = call "myRIO_BRig_RT__Case_Exp_State_Reward.vi"("input_dataCurrent"=w3206, "input_state"=w3203, "input_spout"=w3201) -> ("output_dataCurrent"=w3205:u16[], "output_state"=w3204:T2, "output__L"=w3199:bool, "output__R"=w3200:bool)  [unwired: 9 in]
            }
            frame "SelectRewardPost_pre" {
              # "nRewards"
              # "nRewTrials"
              # "Tcycle"
              # "counter"
              n1520 = call "myRIO_BRig_RT_dataBlock_nRewards__L.vi"() -> ("output_nRewards__L"=w3222:i32)  [unwired: 11 in]
              n1521 = call "myRIO_BRig_RT_dataBlock_nRewards__R.vi"() -> ("output_nRewards__R"=w3221:i32)  [unwired: 11 in]
              n1522 = call "myRIO_BRig_RT_dataCurrent_Tcycle_generic.vi"() -> ("output_Tcycle_generic"=w3241:i32)  [unwired: 11 in]
              n1523 = call "myRIO_BRig_RT_dataCurrent_count_generic.vi"() -> ("output_count_generic"=w3243:i32)  [unwired: 11 in]
              n1524 = case shown="\"Left\", Default" w3215 {
                tunnel: w3227 -> [w3248 w3252]
                tunnel: [w3247 w3252] -> w3226
                tunnel: [w3249 w3250] -> w3225
                tunnel: w3224 -> [w3249 w3251]
                frame "Left", Default {
                  n1525 = Increment(x=w3248) -> (x+1=w3247:u16)
                }
                frame "Right" {
                  n1526 = Increment(x=w3251) -> (x+1=w3250:u16)
                }
              }
              "nRewards_Left" <- w3226
              "nRewards_Right" <- w3225
              n1527 = Equal?(x=w3215, y=enum16{"Left", "Right"}."Left") -> (x = y?=w3214:bool)
              n1528 = Select(t=w3222, s=w3214, f=w3221) -> (s? t:f=w3220:i32)
              n1529 = call "myRIO_BRig_RT_dataExp_Tcycle_RewardPost.vi"() -> ("output_Tcycle_RewardPost"=w3237:i32)  [unwired: 11 in]
              n1530 = call "myRIO_BRig_RT_dataCurrent_nRewTrials.vi"() -> ("output_nRewTrials"=w3223:i32)  [unwired: 11 in]
              n1531 = Index Array(array=w3238, index=w3237) -> (element=w3240:u16)
              n1532 = Index Array(array=w3217, index=w3223) -> (element=w3212:u16)
              n1533 = Replace Array Subset(array=w3217, new element #1=u16 0 ("new element/subarray"), index #1=w3243, new element #2=w3240, index #2=w3241) -> (w3239:u16[])
              n1534 = Replace Array Subset(array=w3219, new element=w3212, index (row)=w3213, index (col)=w3220) -> (w3218:u16[][])
              n1535 = local write "nRewards_cur"(w3212) -> ()
            }
            frame "SelectRewardPost" {
              n1536 = call "myRIO_BRig_RT__Case_Exp_State_RewardPost.vi"("input_state"=w3267, "input_dataCurrent"=w3270) -> ("output_state"=w3268:T2, "output_dataCurrent"=w3269:u16[])  [unwired: 8 in]
            }
            frame "SelectWrong_pre" {
              # "iState"
              # "Tcycle"
              # "counter"
              n1537 = call "myRIO_BRig_RT_dataCurrent_Tcycle_generic.vi"() -> ("output_Tcycle_generic"=w3295:i32)  [unwired: 11 in]
              n1538 = call "myRIO_BRig_RT_dataCurrent_count_generic.vi"() -> ("output_count_generic"=w3297:i32)  [unwired: 11 in]
              n1539 = call "myRIO_BRig_RT_dataExp_Tcycle_Wrong.vi"() -> ("output_Tcycle_Wrong"=w3293:i32)  [unwired: 11 in]
              n1540 = call "myRIO_BRig_RT__Case_Exp_subState_LC__Wrong.vi"("input_spout"=w3289, "input_dataCurrent"=w3290, "input_dataLC"=w3287) -> ()  [unwired: 6 in, 2 out]
              n1541 = Index Array(array=w3291, index=w3293) -> (element=w3294:u16)
              n1542 = call "myRIO_BRig_RT_dataCurrent_iState.vi"() -> ("output_iState"=w3281:i32)  [unwired: 11 in]
              n1543 = Replace Array Subset(array=w3290, new element #1=u16 0 ("new element/subarray"), index #1=w3297, new element #2=w3294, index #2=w3295, new element #3=u16 2 ("new element/subarray"), index #3=w3281) -> (w3292:u16[])
            }
            frame "SelectWrong" {
              n1544 = call "myRIO_BRig_RT__Case_Exp_State_Wrong.vi"("input_state"=w3311, "input_dataCurrent"=w3320) -> ("output_state"=w3308:T2, "output_dataCurrent"=w3319:u16[])  [unwired: 8 in]
              n1545 = Not Equal?(x=w3311, y=w3308) -> (x != y?=w3310:bool)
              n1546 = Select(t=myRIO_BRig_RT__Case_Exp_stateList."SelectWrong_post" ("Enum"), s=w3310, f=w3308) -> (s? t:f=w3307:T2)
            }
            frame "SelectWrong_post" {
            }
            frame "SelectTimeout_pre" {
              # "iState"
              # "Tcycle"
              # "counter"
              n1547 = xnode "Read/Write Control"("FPGA VI Reference In"=w3347, "error in"=w3346, "SelectionState"=FALSE) -> ("error out"=w3344:errorcluster)  [unwired: 1 out]
              n1548 = call "myRIO_BRig_RT_dataCurrent_Tcycle_generic.vi"() -> ("output_Tcycle_generic"=w3369:i32)  [unwired: 11 in]
              n1549 = call "myRIO_BRig_RT_dataCurrent_count_generic.vi"() -> ("output_count_generic"=w3367:i32)  [unwired: 11 in]
              n1550 = call "myRIO_BRig_RT_dataExp_Tcycle_Timeout.vi"() -> ("output_Tcycle_Timeout"=w3371:i32)  [unwired: 11 in]
              n1551 = local write "error out"(w3344) -> ()
              n1552 = call "myRIO_BRig_RT__Case_Exp_subState_LC__Timeout.vi"("input_spout"=w3362, "input_dataCurrent"=w3363, "input_dataLC"=w3361) -> ()  [unwired: 6 in, 2 out]
              n1553 = Index Array(array=w3365, index=w3371) -> (element=w3370:u16)
              n1554 = call "myRIO_BRig_RT_dataCurrent_iState.vi"() -> ("output_iState"=w3355:i32)  [unwired: 11 in]
              n1555 = Replace Array Subset(array=w3363, new element #1=u16 0 ("new element/subarray"), index #1=w3367, new element #2=w3370, index #2=w3369, new element #3=u16 3 ("new element/subarray"), index #3=w3355) -> (w3366:u16[])
            }
            frame "SelectTimeout" {
              n1556 = call "myRIO_BRig_RT__Case_Exp_State_Timeout.vi"("input_dataLC"=w3390, "input_state"=w3381, "input_dataCurrent"=w3395) -> ("output_state"=w3382:T2, "output_dataCurrent"=w3394:u16[])  [unwired: 6 in, 1 out]
              n1557 = Not Equal?(x=w3381, y=w3382) -> (x != y?=w3385:bool)
              n1558 = Select(t=myRIO_BRig_RT__Case_Exp_stateList."SelectTimeout_post" ("Enum"), s=w3385, f=w3382) -> (s? t:f=w3383:T2)
            }
            frame "SelectTimeout_post" {
            }
            frame "endTrial1" {
              # "Update dataBlock"
              n1559 = call "myRIO_BRig_RT__Case_Exp_State_endTrial1.vi"("input_spout"=w3428, "input_dataBlock"=w3427, "input_dataCurrent"=w3425) -> ("output_dataBlock"=w3426:u16[][], "output_dataCurrent"=w3424:u16[])  [unwired: 7 in]
            }
            frame "endTrial2" {
              # "update dataTrial"
              n1560 = call "myRIO_BRig_RT__Case_Exp_State_endTrial2.vi"("input_dataExp"=w3439, "input_spout"=w3448, "input_dataTrial"=w3452, "input_dataCurrent"=w3450) -> ("output_dataTrial"=w3451:u16[][], "output_dataCurrent"=w3449:u16[])  [unwired: 6 in]
            }
            frame "endTrial3" {
              # "nRewTrials"
              # "iTrial"
              # "I_blockUntilReward"
              # "TPB"
              # "end block?"
              n1561 = local read "STOP_endTrial"() -> (w3477:bool)
              n1562 = local read "STOP_abort"() -> (w3476:bool)
              n1563 = xnode "Read/Write Control"("FPGA VI Reference In"=w3467, "error in"=w3466, "SelectionState"=FALSE) -> ("error out"=w3460:errorcluster)  [unwired: 1 out]
              n1564 = local read "START"() -> (w3474:bool)
              n1565 = call "myRIO_BRig_RT_dataExp_IblockUntilReward.vi"() -> ("output_I_blockUntilReward"=w3484:i32)  [unwired: 11 in]
              n1566 = Index Array(array=w3470, index=w3484) -> (element=w3468:u16)
              n1567 = Not(x=w3474) -> (.not. x?=w3475:bool)
              n1568 = local write "error out"(w3460) -> ()
              n1569 = Not Equal To 0?(x=w3468) -> (x != 0?=w3482:bool)
              n1570 = Compound Arithmetic op=OR(w3477, w3475, w3476) -> (w3463:bool)
              n1571 = call "myRIO_BRig_RT_dataCurrent_nRewTrials.vi"() -> ("output_nRewTrials"=w3480:i32)  [unwired: 11 in]
              n1572 = call "myRIO_BRig_RT_dataCurrent_iTrial.vi"() -> ("output_iTrial"=w3481:i32)  [unwired: 11 in]
              n1573 = Select(t=w3480, s=w3482, f=w3481) -> (s? t:f=w3479:i32)
              n1574 = call "myRIO_BRig_RT_dataCurrent_TpB.vi"() -> ("output_TpB"=w3483:i32)  [unwired: 11 in]
              n1575 = Index Array(array=w3471, index #1=w3483, index #2=w3479) -> (element #1=w3472:u16, element #2=w3473:u16)
              n1576 = Less Or Equal?(x=w3472, y=w3473) -> (x <= y?=w3464:bool)
              n1577 = Or(x=w3463, y=w3464) -> (x .or. y?=w3461:bool)
              n1578 = Select(t=myRIO_BRig_RT__Case_Exp_stateList."saveData_dataBlock" ("Enum"), s=w3461, f=myRIO_BRig_RT__Case_Exp_stateList."dummyState" ("Enum")) -> (s? t:f=w3469:T2)
            }
            frame "endBlock" {
              # "R"
              # "L"
              # "idxDataBlock"
              n1579 = Equal?(x=w3508, y=enum16{"Left", "Right"}."Left") -> (x = y?=w3507:bool)
              n1580 = call "myRIO_BRig_RT_dataCurrent_idxDataBlockL.vi"() -> ("output_idxDataBlock__L"=w3511:i32)  [unwired: 11 in]
              n1581 = call "myRIO_BRig_RT_dataCurrent_idxDataBlockR.vi"() -> ("output_idxDataBlock__R"=w3510:i32)  [unwired: 11 in]
              n1582 = Increment(x=w3502) -> (x+1=w3501:i32)
              n1583 = local read "START"() -> (w3531:bool)
              n1584 = local read "STOP_endBlock"() -> (w3526:bool)
              n1585 = local read "STOP_endTrial"() -> (w3529:bool)
              n1586 = local read "STOP_abort"() -> (w3528:bool)
              n1587 = Select(t=w3511, s=w3507, f=w3510) -> (s? t:f=w3505:i32)
              n1588 = To Unsigned Word Integer(number=w3501) -> (unsigned 16bit integer=w3503:u16)
              n1589 = Not(x=w3531) -> (.not. x?=w3530:bool)
              n1590 = Replace Array Subset(array=w3506, new element=w3503, index=w3505) -> (w3504:u16[])
              n1591 = Compound Arithmetic op=OR(w3530, w3526, w3529, w3528) -> (w3527:bool)
              n1592 = Select(t=myRIO_BRig_RT__Case_Exp_stateList."endExp" ("Enum"), s=w3527, f=myRIO_BRig_RT__Case_Exp_stateList."dummyState_endBlock" ("Enum")) -> (s? t:f=w3535:T2)
            }
            frame "endExp" {
            }
            frame "commConnect" {
              n1593 = call "myRIO_BRig_RT_comm_webdav_connect.vi"("input_password"="Host Password", "input_username"="Host UserName") -> ("output_Iconnected"=w3556:bool, "output_hSession"=w3574:T6)  [unwired: 7 in, 1 out]
              "Connected To Host?" <- w3556
              n1594 = case shown="False" w3556 {
                frame False {
                  n1595 = One Button Dialog(message="Connection Failed!\nData not being saved!") -> ()  [unwired: 1 in, 1 out]
                }
                frame True {
                }
              }
            }
            frame "commUpload_pre" {
              n1596 = Select(t=myRIO_BRig_RT__Case_Exp_stateList."commUpload_dataBlock" ("Enum"), s=w3581, f=myRIO_BRig_RT__Case_Exp_stateList."endBlock") -> (s? t:f=w3579:T2)
            }
            frame "commUpload_dataBlock" {
              n1597 = call "myRIO_BRig_RT_comm_webdav_uploadFile__data.vi"("input_fileName_prefix"=w3602, "input_fileName"="dataBlock" ("input_filename"), "input_hSession"=w3604) -> ()  [unwired: 8 in, 1 out]
            }
            frame "commUpload_dataCurrent" {
              n1598 = call "myRIO_BRig_RT_comm_webdav_uploadFile__data.vi"("input_fileName_prefix"=w3623, "input_fileName"="dataCurrent" ("input_filename"), "input_hSession"=w3625) -> ()  [unwired: 8 in, 1 out]
            }
            frame "commUpload_dataExp" {
              n1599 = call "myRIO_BRig_RT_comm_webdav_uploadFile__data.vi"("input_fileName_prefix"=w3644, "input_fileName"="dataExp" ("input_filename"), "input_hSession"=w3646) -> ()  [unwired: 8 in, 1 out]
            }
            frame "commUpload_dataLC" {
              n1600 = call "myRIO_BRig_RT_comm_webdav_uploadFile__data.vi"("input_fileName_prefix"=w3665, "input_fileName"="dataLC" ("input_filename"), "input_hSession"=w3667) -> ()  [unwired: 8 in, 1 out]
            }
            frame "commUpload_dataTrial" {
              n1601 = call "myRIO_BRig_RT_comm_webdav_uploadFile__data.vi"("input_fileName_prefix"=w3689, "input_fileName"="dataTrial" ("input_filename"), "input_hSession"=w3691) -> ()  [unwired: 8 in, 1 out]
            }
            frame "saveData_dataBlock" {
              # "idxDataBlockR"
              # "idxDataBlockL"
              n1602 = call "myRIO_BRig_RT_dataCurrent_idxDataBlockL.vi"() -> ("output_idxDataBlock__L"=w3715:i32)  [unwired: 11 in]
              n1603 = call "myRIO_BRig_RT_dataCurrent_idxDataBlockR.vi"() -> ("output_idxDataBlock__R"=w3716:i32)  [unwired: 11 in]
              n1604 = Index Array(array=w3717, index #1=w3715, index #2=w3716) -> (element #1=w3714:u16, element #2=w3713:u16)
              n1605 = Greater?(x=w3714, y=w3713) -> (0:w3712:bool)
              n1606 = Select(t=w3714, s=w3712, f=w3713) -> (s? t:f=w3710:u16)
              n1607 = Increment(x=w3710) -> (x+1=w3709:u16)
              n1608 = To Long Integer(number=w3709) -> (32bit integer=w3708:i32)
              n1609 = Array Subset(array=w3711, length (row)=w3708) -> (w3707:u16[][])  [unwired: 3 in]
              n1610 = call "myRIO_BRig_RT_comm_webdav_saveArrayToFile__2D_u16.vi"("Array"=w3707, "input_filename"="dataBlock") -> ()  [unwired: 10 in]
            }
            frame "saveData_dataCurrent" {
              n1611 = call "myRIO_BRig_RT_comm_webdav_saveArrayToFile__1D_u16.vi"("Array"=w3736, "input_filename"="dataCurrent") -> ()  [unwired: 10 in]
            }
            frame "saveData_dataExp" {
              # "runTime"
              n1612 = Get Date/Time In Seconds() -> (seconds since 1Jan1904=w3764:timestamp)
              n1613 = To Double Precision Float(number=w3764) -> (double precision float=w3763:dbl)
              n1614 = call "myRIO_BRig_RT_dataExp_runTime_seconds.vi"() -> ("output_RunTime_minutes"=w3762:i32)  [unwired: 11 in]
              n1615 = Subtract(x=w3763, y=w3761) -> (x-y=w3758:dbl)
              n1616 = To Unsigned Word Integer(number=w3758) -> (unsigned 16bit integer=w3757:u16)
              n1617 = Replace Array Subset(array=w3756, new element=w3757, index=w3762) -> (w3759:u16[])
              n1618 = call "myRIO_BRig_RT_comm_webdav_saveArrayToFile__1D_u16.vi"("Array"=w3759, "input_filename"="dataExp") -> ()  [unwired: 10 in]
            }
            frame "saveData_dataLC" {
              n1619 = call "myRIO_BRig_RT_comm_webdav_saveArrayToFile__1D_u16.vi"("Array"=w3783, "input_filename"="dataLC") -> ()  [unwired: 10 in]
            }
            frame "saveData_dataTrial" {
              # "idxTrial"
              n1620 = call "myRIO_BRig_RT_dataCurrent_idxDataTrial.vi"() -> ("output_idxDataTrial"=w3807:i32)  [unwired: 11 in]
              n1621 = Index Array(array=w3808, index=w3807) -> (element=w3800:u16)
              n1622 = Increment(x=w3800) -> ()  [unwired: 1 out]
              n1623 = To Long Integer(number=w3800) -> (32bit integer=w3804:i32)
              n1624 = Array Subset(array=w3805, length (row)=w3804) -> (w3806:u16[][])  [unwired: 3 in]
              n1625 = call "myRIO_BRig_RT_comm_webdav_saveArrayToFile__2D_u16.vi"("Array"=w3806, "input_filename"="dataTrial") -> ()  [unwired: 10 in]
            }
            frame "dummyState" {
              n1626 = call "myRIO_BRig_RT_dataCurrent_iTrial.vi"() -> ("output_iTrial"=w3830:i32)  [unwired: 11 in]
              n1627 = Index Array(array=w3831, index=w3830) -> (element=w3829:u16)
              n1628 = Equal?(x=w3829, y=u16 1) -> (x = y?=w3827:bool)
              n1629 = Equal To 0?(x=w3838) -> (x = 0?=w3839:bool)
              n1630 = Select(t=u16 13, s=w3827, f=u16 15) -> (s? t:f=w3824:u16)
              n1631 = Select(t=w3824, s=w3839, f=w3838) -> (s? t:f=w3837:u16)
              n1632 = Decrement(x=w3837) -> (x-1=w3836:u16)
              n1633 = Equal To 0?(x=w3836) -> (x = 0?=w3835:bool)
              n1634 = Select(t=myRIO_BRig_RT__Case_Exp_stateList."initTrial" ("Enum"), s=w3835, f=w3833) -> (s? t:f=w3832:T2)
            }
            frame "dummyState_endBlock" {
              n1635 = call "myRIO_BRig_RT_dataCurrent_iTrial.vi"() -> ("output_iTrial"=w3863:i32)  [unwired: 11 in]
              n1636 = Index Array(array=w3864, index=w3863) -> (element=w3862:u16)
              n1637 = Equal?(x=w3862, y=u16 1) -> (x = y?=w3860:bool)
              n1638 = Equal To 0?(x=w3871) -> (x = 0?=w3872:bool)
              n1639 = Select(t=u16 1, s=w3860, f=u16 3) -> (s? t:f=w3857:u16)
              n1640 = Select(t=w3857, s=w3872, f=w3871) -> (s? t:f=w3870:u16)
              n1641 = Decrement(x=w3870) -> (x-1=w3869:u16)
              n1642 = Equal To 0?(x=w3869) -> (x = 0?=w3868:bool)
              n1643 = Select(t=myRIO_BRig_RT__Case_Exp_stateList."initBlock" ("Enum"), s=w3868, f=w3866) -> (s? t:f=w3865:T2)
            }
          }
          n1644 = call "myRIO_BRig_RT_dataMTrig_main.vi"("input_dataMTrig"=w1666, "input_Solenoid_trig_L"=w1663, "input_Solenoid_trig_R"=w1662, "input_Audio_trig_L"=w1661, "input_Audio_trig_R"=w1660, "input_Laser_trig"=w1659) -> ("output_Laser"=w1594:bool, "output_dataMTrig"=w1665:u16[], "output_Solenoid_L"=w1597:bool, "output_Solenoid_R"=w1655:bool, "output_Audio_L"=w1657:bool, "output_Audio_R"=w1658:bool)  [unwired: 8 in]
          n1645 = Compound Arithmetic op=OR(w1663, w1662, w1661, w1660, w1659) -> (w1664:bool)
          n1646 = case shown="True" w1664 {
            frame False {
            }
            frame True {
              w1703 = FALSE
              n1647 = local write "MTrig_Solenoid_trig__L"(w1703) -> ()
              n1648 = local write "MTrig_Solenoid_trig__R"(w1703) -> ()
              n1649 = local write "MTrig_Audio_trig__L"(w1703) -> ()
              n1650 = local write "MTrig_Audio_trig__R"(w1703) -> ()
              n1651 = local write "MTrig_Laser_trig"(w1703) -> ()
            }
          }
          n1652 = local read "MTrig_Laser_Switch"() -> (w1592:bool)
          n1653 = Not(x=w1592) -> (.not. x?=w1593:bool)
          n1654 = Select(t=w1627, s=w1630, f=w1628) -> (s? t:f=w1629:bool)
          n1655 = And(x=w1594, y=w1593) -> (x .and. y?=w1588:bool)
          n1656 = And(x=w1594, y=w1592) -> (x .and. y?=w1590:bool)
          n1657 = Or(x=w1591, y=w1590) -> (x .or. y?=w1581:bool)
          n1658 = Or(x=w1590, y=w1589) -> (x .or. y?=w1580:bool)
          n1659 = Or(x=w1587, y=w1588) -> (x .or. y?=w1583:bool)
          n1660 = Or(x=w1588, y=w1586) -> (x .or. y?=w1582:bool)
          n1661 = Or(x=w1596, y=w1597) -> (x .or. y?=w1585:bool)
          n1662 = Or(x=w1656, y=w1655) -> (x .or. y?=w1584:bool)
          n1663 = case shown="False" w1683 {
            tunnel: w1680 -> [w1705 w1713]
            tunnel: w1682 -> [_ w1710]
            tunnel: w1681 -> [_ w1709]
            tunnel: w1571 -> [_ w1708]
            tunnel: w1653 -> [_ w1707]
            tunnel: [w1705 w1712] -> w1679
            tunnel: [w1704 w1711] -> w1678
            tunnel: w1579 -> [w1704 w1706]
            frame False {
            }
            frame True {
              n1664 = call "myRIO_BRig_RT__Case_Exp__recordLick.vi"("intput_state__trialEnd"=w1707, "intput_state__trialStart"=w1708, "input_lick__R"=w1709, "input_lick__L"=w1710, "input_dataCurrent"=w1706, "input_dataLick"=w1713) -> ("output_dataCurrent"=w1711:u16[], "output_dataLick"=w1712:u16[][])  [unwired: 4 in]
            }
          }
          n1665 = Or(x=w1657, y=w1642) -> (x .or. y?=w1631:bool)
          n1666 = Or(x=w1641, y=w1658) -> (x .or. y?=w1654:bool)
          n1667 = Or(x=w1684, y="STOP_abort") -> (x .or. y?=w1686:bool)
          n1668 = Select(t=w1617, s=w1618, f=w1616) -> (s? t:f=w1607:u16)
          n1669 = Select(t=w1578, s=w1620, f=w1619) -> (s? t:f=w1606:u16)
          n1670 = Select(t=u16 0, s=w1623, f=w1622) -> (s? t:f=w1609:u16)
          n1671 = xnode "Read/Write Control"("FPGA VI Reference In"=w1633, "error in"=w1632, "A6_Act"=w1629, "audioTrigger_L"=w1631, "audioAmp_L"=w1667, "audioFreq_L_kHz"=w1640, "audioTrigger_R"=w1654, "audioAmp_R"=w1668, "audioFreq_R_kHz"=w1669, "CueLed_Event"=w1595, "A3_SL"=w1585, "A1_SR"=w1584, "LC_Event_l1"=w1583, "LC_Laser_l1"=w1582, "LC_Event_l2"=w1581, "LC_Laser_l2"=w1580) -> ("FPGA VI Reference Out"=w1677:refnum<k20>, "error out"=w1676:errorcluster, "AnaIn_0"=w1600:i16, "AnaIn_1"=w1608:i16)
          n1672 = call "myRIO_BRig_RT_dataAnalog_enterData__PortC.vi"("input_iState"=w1571, "input_AI0"=w1600, "input_iEvent"=w1609, "input_AI1"=w1608, "input_iTrial"=w1607, "input_iBlock"=w1606, "input_index"=w1610, "input_dataAnalog"=w1626) -> ("output_dataAnalog"=w1625:u16[][])  [unwired: 3 in]
          n1673 = call "myRIO_BRig_RT_TCP__v3__PortC.vi"("input_hTCP"=w1614, "input_AI1"=w1608, "input_AI0"=w1600, "input_I_connected_TCP"=w1611, "input_iBlock"=w1606, "input_spout"=w1605, "input_iTrial"=w1607, "input_error"=w1612, "input_countTrial"=w1602, "input_iState"=w1571) -> ("output_hTCP"=w1613:refnum<k5>, "output_countTrial"=w1601:u16, "output_error"=w1575:errorcluster)  [unwired: 3 in]
          n1674 = call "test_myRIO_Exp_tLoop.vi"("input_error"=w1575, "input_Threshold"=w1572, "input_timestamp"=w1573, "input_state"=w1571) -> ("output_Threshold"=w1569:bool, "output_duration"=→"tLoop":dbl, "error out"=w1574:errorcluster)  [unwired: 5 in]
          "Threshold" <- w1569
          n1675 = node-c288() -> ()  [unwired: 1 in, 1 out]
          n1676 = Increment(x=w1609) -> (x+1=w1615:u16)
          n1677 = Increment(x=w1610) -> (x+1=w1624:i32)
          "cState" <- w1571
        }
        n1678 = node-c288(w1519) -> ()  [unwired: 1 out]
        n1679 = flat-sequence {
          tunnel: w1515 -> [w1564]
          tunnel: w1514 -> [w1563]
          tunnel: [w1562] -> w1507
          tunnel: [w1561] -> w1506
          tunnel: [w1567] -> w1508
          tunnel: [w1568] -> w1513
          tunnel: w1507 -> [w1568]
          tunnel: w1506 -> [w1567]
          frame #0 {
            w1558 = u8 0
            w1559 = u16 0 ("AudioLeft_phase_inc")
            w1560 = FALSE
            n1680 = xnode "Read/Write Control"("FPGA VI Reference In"=w1564, "error in"=w1563, "Counts_Reset"=TRUE, "audioTrigger_L"=w1560, "audioFreq_L_kHz"=w1558, "audioAmp_L"=w1559, "audioTrigger_R"=w1560, "audioFreq_R_kHz"=w1558, "audioAmp_R"=w1559, "A3_SL"=w1560, "A1_SR"=w1560, "A6_Act"=w1560) -> ("FPGA VI Reference Out"=w1562:refnum<k20>, "error out"=w1561:errorcluster)
          }
          frame #1 {
            w1566 = FALSE ("START")
            n1681 = local write "START"(w1566) -> ()
            n1682 = local write "STOP_endTrial"(w1566) -> ()
            n1683 = local write "STOP_endBlock"(w1566) -> ()
          }
        }
        n1684 = stacked-sequence {
          tunnel: w1491 -> [w1538 _]
          tunnel: w1489 -> [w1539 _]
          tunnel: w1488 -> [_ w1544]
          tunnel: w1487 -> [_ w1543]
          tunnel: w1486 -> [_ w1542]
          tunnel: w1485 -> [w1532 _]
          tunnel: w1465 -> [w1529 _]
          tunnel: w1464 -> [w1528 _]
          frame #0 {
            n1685 = call "myRIO_BRig_RT_dataCurrent_idxDataLick.vi"() -> ("output_idxDataLick"=w1533:i32)  [unwired: 11 in]
            n1686 = Index Array(array=w1532, index=w1533) -> (element=w1535:u16)
            n1687 = Array Subset(array=w1529, length (row)=w1528) -> (w1530:u16[][])  [unwired: 3 in]
            n1688 = Increment(x=w1535) -> (x+1=w1536:u16)
            n1689 = call "myRIO_BRig_RT_comm_webdav_saveArrayToFile__1D_u16.vi"("Array"=w1539, "input_filename"="dataMTrig") -> ()  [unwired: 10 in]
            n1690 = To Long Integer(number=w1536) -> (32bit integer=w1534:i32)
            n1691 = Array Subset(array=w1538, length (row)=w1534) -> (w1537:u16[][])  [unwired: 3 in]
            n1692 = call "myRIO_BRig_RT_comm_webdav_saveArrayToFile__2D_u16.vi"("Array"=w1537, "input_filename"="dataLick") -> ()  [unwired: 10 in]
            n1693 = call "myRIO_BRig_RT_comm_webdav_saveArrayToFile__2D_u16.vi"("Array"=w1530, "input_filename"="dataAnalog") -> ()  [unwired: 10 in]
          }
          frame #1 {
            n1694 = case shown="True" w1544 {
              tunnel: w1543 -> [_ w1546]
              tunnel: w1542 -> [_ w1545]
              frame False {
              }
              frame True {
                n1695 = stacked-sequence {
                  tunnel: w1546 -> [w1548 w1555 w1557]
                  tunnel: w1545 -> [w1549 w1554 _]
                  frame #0 {
                    n1696 = call "myRIO_BRig_RT_comm_webdav_uploadFile__announce.vi"("input_addText"=TRUE, "input_fileName_prefix"=w1549, "intput_fileName"="curExp_end", "intput_hSession"=w1548) -> ("output_Isuccess"=w1547:bool)  [unwired: 6 in, 1 out]
                    n1697 = case shown="True" w1547 {
                      frame False {
                        n1698 = One Button Dialog(message="!!! Warning !!! Your data is located at C:\\BehaviorRig\\commTransfer") -> ()  [unwired: 1 in, 1 out]
                      }
                      frame True {
                        n1699 = Wait (ms)(milliseconds to wait=u32 20) -> ()  [unwired: 1 out]
                      }
                    }
                  }
                  frame #1 {
                    n1700 = call "myRIO_BRig_RT__endExp_sendData.vi"("input_fileName_prefix"=w1554, "input_hSession"=w1555) -> ()  [unwired: 8 in, 2 out]
                  }
                  frame #2 {
                    n1701 = local write "Connected To Host?"(FALSE ("Connected To Host?")) -> ()
                    n1702 = call <vilib>:"Close Session.vi"("session handle"=w1557) -> ()  [unwired: 14 in, 1 out]
                  }
                }
              }
            }
          }
        }
      }
    }
    n1703 = local read "STOP_abort"() -> (w44:bool)
  }
  n1704 = case shown="True" w5 {
    tunnel: w4 -> [_ w3895]
    tunnel: w3 -> [_ w3894]
    frame False {
    }
    frame True {
      n1705 = call "myRIO__TCP_disconnect_forWrite.vi"("input_error"=w3894, "input_hTCP"=w3895) -> ()  [unwired: 9 in, 1 out]
    }
  }
  n1706 = xnode "Read/Write Control"("FPGA VI Reference In"=w16, "error in"=w15, "FPGA_Stop"=TRUE) -> ("FPGA VI Reference Out"=w21:refnum<k20>, "error out"=w22:errorcluster)
  n1707 = xnode "Close FPGA VI Reference"("FPGA VI Reference In"=w21, "error in"=w22) -> ("error out"=w20:errorcluster)
  n1708 = call <vilib>:"Reset myRIO.vi"("error in (no error)"=w20) -> ()  [unwired: 10 in, 1 out]
